vi "FP_Tracker_2.1.vi"(8 "error in (no error)":errorcluster, 11 "Settings file path":path=path "D:/Users/Dmitriy/CData/CloudStation/Tracker_repository/SubVi's/Tracker_settings.tcf") -> (0 "error out":errorcluster)   [LabVIEW 2018]
uses:
  <vilib>/Utility/config.llb/Config Data RefNum.ctl
  <vilib>/Utility/miscctls.llb/LVPoint32TypeDef.ctl
  SubVi's/Controls/CTL_Data_flow_control_cluster.ctl
  <vilib>/Instr/_visa.llb/VISA Flush IO Buffer Mask.ctl
  <vilib>/Utility/miscctls.llb/LVPointTypeDef.ctl
  <vilib>/Utility/miscctls.llb/LVOffsetAndMultiplierTypeDef.ctl
  <vilib>/Utility/miscctls.llb/LVRangeTypeDef.ctl
  <vilib>/Platform/TimedLoop/XDataNode/timing_clust.ctl
  <vilib>/Platform/TimedLoop/XDataNode/nitl_modes.ctl
  <vilib>/Platform/TimedLoop/XDataNode/wakeup.ctl
  <vilib>/Instr/_visa.llb/VISA Open Access Mode.ctl
  <vilib>/Utility/sysdir.llb/System Directory Type.ctl
  <vilib>/Utility/miscctls.llb/LVBoundsTypeDef.ctl
  <vilib>/ChannelSupport/Lossy Behavior.ctl
  <extravilib>/ChannelInstances/Lossy Stream-a[.](str)/Read With Abort.vi
  <extravilib>/ChannelInstances/Lossy Stream-a[.,.](str)/Read With Abort.vi
  <extravilib>/ChannelInstances/Lossy Stream-a[.](str)/Write With Abort.vi
  <extravilib>/ChannelInstances/Lossy Stream-a[.,.](str)/Write With Abort.vi
  <extravilib>/ChannelInstances/Lossy Stream-a[.](str)/EndpointRead.vi
  <extravilib>/ChannelInstances/Lossy Stream-a[.,.](str)/EndpointRead.vi
  <extravilib>/ChannelInstances/Lossy Stream-a[.](str)/Endpoint.vi
  <extravilib>/ChannelInstances/Lossy Stream-a[.,.](str)/Endpoint.vi
  SubVi's/SW_Globals.vi
  <vilib>/Platform/TimedLoop/scheduler/LVUserAPI/_suppVIs/Create_1kHz_TSource.vi
  <extravilib>/ChannelInstances/Lossy Stream-a[.](str)/Instantiate.vi
  <extravilib>/ChannelInstances/Lossy Stream-a[.,.](str)/Instantiate.vi
  <extravilib>/ChannelInstances/Lossy Stream-a[.](str)/)Channel.vi
  <resource>/ChannelSupport/_ChannelSupport/WaitIfNeeded.vi
  <extravilib>/ChannelInstances/Lossy Stream-a[.,.](str)/)Channel.vi
  <vilib>/Utility/file.llb/Write Delimited Spreadsheet (I64).vi
  <vilib>/Platform/TimedLoop/XDataNode/XDataNode.xnode
  <vilib>/Utility/config.llb/NI_LVConfig.lvlib
  Tracker.lvlib
  <vilib>/Utility/file.llb/Write Delimited Spreadsheet (string).vi
  <extravilib>/ChannelInstances/Lossy Stream-a[.,.](str).lvlib
  <vilib>/Platform/TimedLoop/XDataNode/XDNodeRunTimeDep.lvlib
  <vilib>/Analysis/NI_AALBase.lvlib
  <extravilib>/ChannelInstances/Lossy Stream-a[.](str).lvlib
  <vilib>/Utility/file.llb/Read Delimited Spreadsheet (string).vi
  Common_Resources.lvlib
panel:
  out "TTLs":u32[](array[numeric])
  in  "Zones preference empty initialized array":i32[](array[numeric])
  out "Timed structure (Streaming) and VISA error(s)":errorcluster
  out "VISA streaming error out":errorcluster
  out "Latest frame":string[](array[string])
  out "Serial port opened":bool
  in  "Open serial port":bool
  out "FP size change error":errorcluster
  out "FPS status":i32=80
  out "Data flow controls":T1
  in  "Streaming":bool
  out "write status":bool
  out "Last send packet size, bytes":u32
  out "PP status":string
  out "DAQ status":string
  out "Stop TTL is fired":bool
  out "Start TTL is fired":bool
  out "IO paramaters loaded from file":bool
  out "IO parameters loaded cluster":T2
  out "Settings load path":path caption="selected path"
  in  "\"Stop at\" enabled":bool
  in  "Serial OUT name":refnum<visa-resource-name>="Serial_Output"
  out "Output to the external terminal":string="00:00:00.000\t0.000000\t0.000000\t0.000000\t0.000000\t00.000000\t0.000000\t0\t0.000\r\n"
  in  "Twisted neck":bool
  in  "Bridge horizontal offset":sgl min=-70 max=70 step=0.1 format="%#.1g"
  in  "Name Prefix":string="SavedTrack"
  in  "Stop record at":dbl=600.0 caption="Stop at" min=0.0 max=43200.0 step=60.0 format="%<%H:%M:%S>t"
  out "Adv. Stim. set":bool
  in  "Save files First Call":bool=TRUE
  in  "Record start First Call":bool=TRUE
  out "Time per sample mean":dbl format="%0.2f"
  out "Time per sample SD":dbl format="%0.2f"
  out "Save iteration duration":i64
  out "standard deviation":dbl format="%0.2f"
  out "mean":dbl format="%0.2f"
  in  "Type of histogram":u8
  out "TTL 4 counter":u32
  out "TTL 3 counter":u32
  out "TTL 2 counter":u32
  out "TTL 1 counter":u32
  out "Full track plotting":u32
  out "Full track preparation":u32
  out "Main queue":refnum<queue>
  in  "Map index (analysis)":i32
  in  "Full trace color":u32(colorbox)=16711680
  out "Current TTL status":u8
  out "TTL inputs":u8[](array[numeric])
  out "TTL outputs":u8[](array[numeric])
  out "Start/Stop in config":u32
  out "Start/Stop out pulses config":u32
  out "Changed IO":bool
  out "Sync capability":u8
  in  "IO parameters string":string
  out "Reset STIM":bool
  out "Reset REG":bool
  out "Init plot":bool=TRUE
  out "Zones preference array (loaded)":dbl[][](array[numeric])
  out "Current zone":dbl[](array[numeric])
  out "Absolute timestamp (rec)":dbl[](array[numeric])
  in  "Colors for Stim. setup":T3(array[cluster])=[{"Not Selected"=1143775, "Not Selected"=1143775}, {"Not Selected"=14517504, "Not Selected"=14517504}, {"Not Selected"=1976113, "Not Selected"=1976113}, {"Not Selected"=2575993, "Not Selected"=2575993}]
  out "Record":bool
  out "Stopped":bool
  out "Reset starting pulse":bool
  out "TTL is long enough":bool
  out "Started":bool
  out "Coords":T4={"Horizontal"=316, "Vertical"=127}
  out "Button":u16=1
  out "Settings file path":path
  out "Track path":path
  out "Index of the last recorded timepoint":i32
  out "ceil(x): smallest int >= x":dbl
  out "Application Directory":path
  out "Path to the settings file":path=path "D:/Users/Dmitriy/CData/CloudStation/Tracker_repository/Tracker_settings.tcf"
  out "Eff. save interval":sgl=7.981
  out "Relative timestamp (rec)":dbl[](array[numeric])
  out "alpha rot. angle":dbl[](array[numeric])
  out "Y coord":dbl[](array[numeric])
  out "X coord":dbl[](array[numeric])
  out "Zones allocation array":i32[](array[numeric])
  out "Zones presence array":bool[](array[boolean])
  in  "Stop Button":bool
  out "Path to the latest saved temp file":path
  out "Temp file ready":bool
  out "Pixels per mm":dbl=1.1663076923076923
  out "Settings file refnum out":T5
  out "Current User":string="Researcher"
  in  "Main tab control":enum32{"Settings", "Recording", "Analysis"}(tab)
  in  "Set advanced stimulus":bool
  in  "Load settings":bool
  out "IO status indicator":T6
  in  "Set IO config":bool
  in  "Jump to Analysis":bool
  in  "Reset stimuli":bool
  in  "Stimulus presets":T7(array[cluster]) {"TTL out" items=["1"=1, "2"=2, "1 + 2"=3]; "Stimulus, s" min=0 max=10000 step=0.1; "Time, s" min=0 max=10000 step=0.1; "Event type" items=["Time spent in zone", "Future options"]}
  in  "Zone-based stimulus setup":T8(radio)=enum."Zone 13"
  out "Ready":bool=TRUE
  in  "Re-check HW connection":bool
  in  "Reset regions":bool
  in  "Start Tracking button":bool
  in  "Starting angle BORDER":i16
  in  "N segments BORDER":u8=5 min=1 max=12
  in  "N segments MIDFIELD":u8=3 max=8
  in  "Starting angle MIDFIELD":i16=30
  in  "Radius, mm MIDFIELD":u16=110
  in  "Radius, mm CENTER":u16=50 min=5 step=1
  out "Board size":string="Large"
  in  "Cage diameter, mm":u16(ring)=333 items=["180 mm"=180, "240 mm"=240, "290 mm"=290, "325 mm"=325, "327 mm"=327, "333 mm"=333]
  out "Segments diagram":picture
  out "HW info":string
  out "Port":string="Large"
  in  "Expand/hide stream panel (Set)":bool
  out "Run times distrib. indicator":bool
  out "IO pulses count":string
  in  "Bridge swap":bool
  in  "Reset barplot":bool
  out "Mouse speed digi":dbl=0.28949046360238656 caption="Mouse speed" format="%05.1f"
  out "Histograms (normalized)":dbl[](graph)=[0.0, 0.0, 0.0, 0.0, 0.0, 0.0, 0.0, 1.0, 0.0, 0.0, 0.0, 0.0, 0.0, 0.0] caption="Zone preference (normalized)"
  in  "Multiplyer of chart RX":u8(slide)=1 min=1 max=10 step=1 scale=1.0..6.0
  in  "Zones presence indicator":T9={"01"=TRUE, "02"=TRUE, "03"=TRUE, "04"=TRUE, "05"=TRUE, "06"=TRUE, "07"=TRUE, "08"=TRUE, "09"=TRUE, "10"=TRUE, "11"=TRUE, "12"=TRUE, "13"=TRUE}
  in  "Zones":bool=TRUE
  in  "Record/Stop":bool
  out "Diagram at recording":picture caption="Mouse track"
  in  "Trace, s":u16(slide)=5 max=30 step=1 scale=0.0..30.0
  in  "Data filtering":u16(ring)=5 items=["None"=0, "Kalman 1/3"=2, "Kalman 1/8"=3, "SG 3/5"=4, "SG 3/11"=5, "SG 3/31"=6]
  out "Record timestamp":dbl format="%<%H:%M:%S%3u>t"
  out "Current Time":timestamp=timestamp(3610093053.229 s since 1904-01-01) format="%<%H:%M:%S %d.%m.%Y>T"
  in  "Exit (recording)":bool
  out "Mouse speed":waveform(dbl)(graph)={"t0"=timestamp(3610093053.229 s since 1904-01-01), "dt"=1.0, "Y"=[0.28949046360238656]}
  in  "Bridge offset":sgl min=-150 max=150 step=0.1 format="%#.1g"
  out "TTL IO 1 (recording)":bool caption="IO 1"
  out "TTL IO 2 (recording)":bool caption="IO 2"
  out "TTL IO 3 (recording)":bool caption="IO 3"
  out "TTL IO 4 (recording)":bool caption="IO 4"
  out "TTL REC":bool
  out "Mouse running, perc. of time":dbl=0.28949046360238656 caption="Run, %" format="%05.2f"
  out "Zones presense indicator":bool=TRUE
  out "Speed distrib. indicator":bool
  out "Run lengts distrib. indicator":bool
  in  "Additional record settings":bool caption="Add. recording settings"
  in  "Expand/hide stream panel (Rec)":bool
  out "Key_pressed":string
  in  "Back to Settings":bool
  out "Data loading progress":dbl(slide) scale=0.0..100.0
  in  "Speed":u16(ring)=3 items=["25"=75, "10"=30, "6"=18, "4"=12, "2"=6, "1"=3, "2/3"=2, "1/3"=1]
  in  "Timeline":dbl(slide) min=0.0 step=1.0 scale=0.0..656.633 scale format="%<%H:%M:%S>t"
  in  "Multiplyer of chart RX 2":u8(slide)=1 min=1 max=10 step=1 scale=1.0..6.0
  out "Diagram at analysis":picture caption="Mouse track"
  in  "Play/Pause":bool
  out "Recorded at time":timestamp format="%<%H:%M:%S %d.%m.%Y>T"
  out "Recorded timestamp":dbl format="%<%H:%M:%S%3u>t"
  in  "Zones (analysis)":bool=TRUE caption="Zones"
  out "Mouse speed 2":waveform(dbl)(graph) caption="Mouse speed"
  out "Mouse speed digi 2":dbl format="%05.1f"
  out "Zones allocation (normalized) in analysis":dbl[](graph) caption="Zone preference (normalized)"
  out "Recorded by":string
  in  "Trace in analysis, s":u16(slide)=2 caption="Trace, s" max=30 step=1 scale=0.0..30.0
  in  "Open File":bool
  out "Bridge swap (analysis)":bool caption="Swapped"
  in  "Show heatmap (analysis)":bool caption="Heat map"
  in  "Show full track (analysis)":bool caption="Full track"
  out "Bridge Vertical offset (analysis)":sgl caption="Br. offset" min=-60 max=60 step=0.1 format="%#.1g"
  out "TTL IO 2 (analysis)":bool
  out "TTL IO 1 (analysis)":bool
  out "TTL IO 3 (analysis)":bool
  out "TTL IO 4 (analysis)":bool
  in  "Expand/hide stream panel (An)":bool
  out "Click coords, mm":cluster{"X":dbl, "Y":dbl} {"Y" format="%.1f"; "X" format="%.1f"}
  # "v.2.1.10.6"
  # "Cage segmentation"
  # "BORDER"
  # "CENTER"
  # "MIDFIELD"
  # "v.2.1.10.6"
  # "v.2.1.10.6"
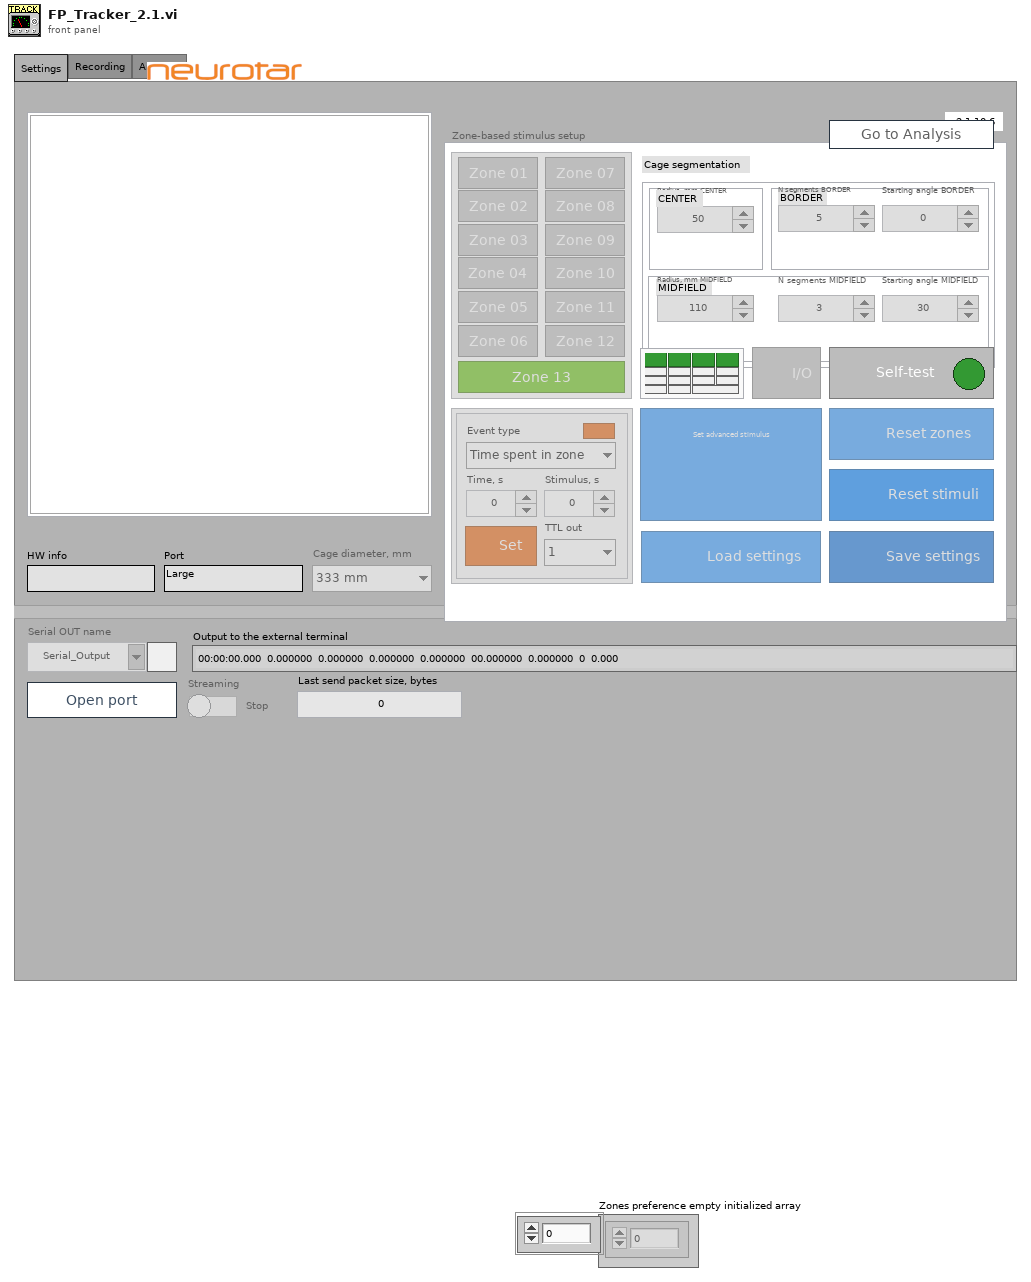
[diagram p1: front panel]
types:
  T1 = typedef "Common_Resources.lvlib/CTL_Data_flow_control_cluster.ctl" = cluster{"Data acquisition status":refnum<notifier>, "Play/Pause status":refnum<notifier>, "Complete stop":refnum<notifier>, "Temp file ready for processing":refnum<notifier>, "Has been recorded":refnum<notifier>, "Recording now":refnum<notifier>, "Path to the latest complete temp file":refnum<notifier>, "(Final) Data file is saved":refnum<notifier>, "Data loaded":refnum<notifier>}
  T2 = cluster{"SYNC configuration":u16, "IO 1 configuration":u16, "IO 2 configuration":u16, "IO 3 configuration":u16, "IO 4 configuration":u16, "Activate ext. RS-232":u16, "IO inversion config.":u16}
  T3 = cluster{"Not Selected":u32, "Not Selected":u32}[]
  T4 = typedef "LVPoint32TypeDef.ctl" = cluster{"Horizontal":i32, "Vertical":i32}
  T5 = typedef "NI_LVConfig.lvlib/Config Data RefNum.ctl" = refnum<k1>
  T6 = cluster{"IO1":bool, "IO2":bool, "IO3":bool, "IO4":bool, "Z1":bool, "Z2":bool, "Z3":bool, "Z4":bool, "St1":bool, "St2":bool, "St3":bool, "St4":bool, "Syn1":bool, "Syn2":bool, "RS-232 ext. activated":bool}
  T7 = cluster{"Event type":u16, "Time, s":sgl, "Stimulus, s":sgl, "Set/Clear":bool, "TTL out":u16, "Stim. has been set":bool}[]
  T8 = enum32{"No Selection", "Zone 01", "Zone 02", "Zone 03", "Zone 04", "Zone 05", "Zone 06", "Zone 07", "Zone 08", "Zone 09", "Zone 10", "Zone 11", "Zone 12", "Zone 13"}
  T9 = cluster{"01":bool, "02":bool, "03":bool, "04":bool, "05":bool, "06":bool, "07":bool, "08":bool, "09":bool, "10":bool, "11":bool, "12":bool, "13":bool}
  T10 = cluster{"SG coefficients 3/5":cluster{"0th order SG coefficients":dbl[], "1st order SG coefficients":dbl[]}, "SG coefficients 3/11":cluster{"0th order SG coefficients":dbl[], "1st order SG coefficients":dbl[]}, "SG coefficients 3/31":cluster{"0th order SG coefficients":dbl[], "1st order SG coefficients":dbl[]}, "SG coefficients 3/51":cluster{"0th order SG coefficients":dbl[], "1st order SG coefficients":dbl[]}}
  T11 = cluster{"Numeric Control":u32, "Numeric Control":u32}[]
  T12 = enum8{"Enabled", "Disabled", "Disabled and Grayed Out"}
  T13 = typedef "XDNodeRunTimeDep.lvlib/timing_clust.ctl" = cluster{"Expected End [f-1]":u64, "Actual End [f-1]":u64, "Finished Late? [f-1]":bool, "Expected End [i-1]":u64, "Actual End [i-1]":u64, "Finished Late? [i-1]":bool, "Expected Start [i]":u64, "Actual Start [i]":u64, "Expected Start [f]":u64, "Actual Start [f]":u64, "Source Name":string, "Structure Name":string, "Period":i64, "Deadline":i64, "Offset":i64, "Start":i64, "Priority":i32, "Timeout":i32, "Mode":T14, "Wakeup Reason":T15, "Error":errorcluster, "Source Type":string, "Secondary Source Type":string, "Global End Time":u64, "Global Start Time":u64, "Frame Duration":u64, "Iteration Duration":u64, "Assigned CPU":i32, "I/O Scan Engine Mode":u32}
  T14 = typedef "XDNodeRunTimeDep.lvlib/nitl_modes.ctl" = enum32{"No Change", "Process missed periods, maintain original phase", "Discard missed periods, maintain original phase", "Process missed periods, ignore original phase", "Discard missed periods, ignore original phase"}
  T15 = typedef "XDNodeRunTimeDep.lvlib/wakeup.ctl" = enum32{"Normal", "Aborted", "Asynchronous wakeup", "Timing source error", "Timed loop error", "Timeout"}
  T16 = cluster{"Read buffer":string, "Timestamp":timestamp}
  T17 = cluster{"Data acquisition status":refnum<notifier>, "Play/Pause status":refnum<notifier>, "Complete stop":refnum<notifier>, "Temp file ready for processing":refnum<notifier>, "Has been recorded":refnum<notifier>, "Recording now":refnum<notifier>, "Path to the latest complete temp file":refnum<notifier>, "Final CSV saved":refnum<notifier>, "Data loaded":refnum<notifier>}
  T18 = typedef "VISA Flush IO Buffer Mask.ctl" = u16
  T19 = typedef "LVBoundsTypeDef.ctl" = cluster{"Width":u32, "Height":u32}
  T20 = cluster{"Amount of border segments":u8, "Border segments starting angle":i16, "Amount of midfield segments":u8, "Midfield segments starting angle":i16, "Midfield segments outer radius, mm":u16, "Amount of central segments":u8, "Center segment outer radius, mm":u16, "Diameter of the cage, mm":u16, "R-gap between segments, mm":u8}
  T21 = typedef "LVRangeTypeDef.ctl" = cluster{"Minimum":dbl, "Maximum":dbl, "Increment":dbl, "Minor Increment":dbl, "Start":dbl}
  T22 = cluster{"Temporary file output path":path, "Density map array output path":path, "Recording settings output path":path, "Density map picture output path":path, "Layout picture output path":path, "Path to the settings file":path, "Path to TDMS file":path, "TDMS file reference":refnum<k34>}
  T23 = cluster{"Zones preference array (loaded)":dbl[][], "TTL inputs":u8[], "TTL outputs":u8[], "Stimulus presets array (loaded)":cluster{"Event type":u16, "Time, s":sgl, "Stimulus, s":sgl, "Set/Clear":bool, "TTL out":u16, "Stim. has been set":bool}[], "Absolute timestamp":dbl[], "Relative timestamp":dbl[], "X coord":dbl[], "Y coord":dbl[], "alpha rot. angle":dbl[], "Current zone":dbl[], "Acquisition settings cluster out":cluster{"Researcher name":string, "N segments MIDFIELD":u8, "N segments BORDER":u8, "Radius, mm CENTER":u16, "Radius, mm MIDFIELD":u16, "Starting angle MIDFIELD":i16, "Starting angle BORDER":i16, "Cage diameter, mm":u16, "Bridge swap":bool, "Bridge V. offset":sgl, "Twisted neck":bool, "Offset H.":sgl, "Name prefix":string, "Stop at":dbl, "\"Stop at\" enabled":bool, "Settings loaded OK":bool}, "Data column names":string[]}
  T24 = cluster{"Absolute timestamp (DBL)":dbl[], "Relative timestamp (DBL)":dbl[], "Zones normalized allocation array":dbl[][], "Coordinates and speed":dbl[][], "Current zone and TTLs":u8[][], "Acquisition settings cluster out":cluster{"Researcher name":string, "N segments MIDFIELD":u8, "N segments BORDER":u8, "Radius, mm CENTER":u16, "Radius, mm MIDFIELD":u16, "Starting angle MIDFIELD":i16, "Starting angle BORDER":i16, "Cage diameter, mm":u16, "Bridge swap":bool, "Bridge V. offset":sgl, "Twisted neck":bool, "Offset H.":sgl, "Name prefix":string, "Stop at":dbl, "\"Stop at\" enabled":bool, "Settings loaded OK":bool}, "Stimulus presets array":cluster{"Event type":u16, "Time, s":sgl, "Stimulus, s":sgl, "Set/Clear":bool, "TTL out":u16, "Stim. has been set":bool}[]}
  T25 = cluster{"Researcher name":string, "N segments MIDFIELD":u8, "N segments BORDER":u8, "Radius, mm CENTER":u16, "Radius, mm MIDFIELD":u16, "Starting angle MIDFIELD":i16, "Starting angle BORDER":i16, "Cage diameter, mm":u16, "Bridge swap":bool, "Bridge V. offset":sgl, "Twisted neck":bool, "Offset H.":sgl, "Name prefix":string, "Stop at":dbl, "\"Stop at\" enabled":bool, "Settings loaded OK":bool}
  T26 = typedef "imagedata.ctl" = cluster{"image type":i32, "image depth":i32, "image":u8[], "mask":u8[], "colors":u32[], "Rectangle":cluster{"left":i16, "top":i16, "right":i16, "bottom":i16}}
  T27 = cluster{"Fonts scale factor":dbl, "Pixels per mm":dbl, "Radius of displayed outer segments, pix":dbl, "Radius of displayed midfield segments, pix":dbl, "Radius of displayed central segment, pix":dbl}
  T28 = cluster{"Width":u16, "Style":enum32{"Solid", "Dash", "Dot", "DashDot", "DashDotDot"}}
  T29 = cluster{"N segments BORDER":u8, "Starting angle BORDER":i16, "N segments MIDFIELD":u8, "Starting angle MIDFIELD":i16, "Radius, mm MIDFIELD":u16, "Amount of central segments":u8, "Radius, mm CENTER":u16}
  T30 = typedef "LVOffsetAndMultiplierTypeDef.ctl" = cluster{"Offset":dbl, "Multiplier":dbl}
  T31 = enum32{"No Selection", "Zone 01", "Zone 02", "Zone 03", "Zone 04", "Zone 05", "Zone 06", "Zone 07", "Zone 08", "Zone 09", "Zone 10", "Zone 11", "Zone 12", "Zone 13", "Zone 14"}
  T32 = enum32{"Page Enabled", "Page Disabled", "Page Disabled & Grayed"}
  T33 = typedef "LVPointTypeDef.ctl" = cluster{"Horizontal":i16, "Vertical":i16}
  T34 = enum32{"invalid app kind", "Development System", "Run Time System", "Student Edition", "Embedded LabVIEW", "Evaluation", "Custom"}
  T35 = cluster{"Researcher name":string, "N segments MIDFIELD":u8, "N segments BORDER":u8, "Radius, mm CENTER":u16, "Radius, mm MIDFIELD":u16, "Starting angle MIDFIELD":i16, "Starting angle BORDER":i16, "Cage diameter, mm":u16, "Bridge swap":bool, "Bridge V. offset":sgl, "Twisted neck":bool, "Offset H.":sgl, "Name prefix":string, "Stop at":dbl, "\"Stop at\" enabled":bool, "Data filtering":u16, "Settings loaded OK":bool}
  T36 = cluster{"Event type":u16, "Dur., s":sgl, "Stim., s":sgl, "Set/Clear":bool, "TTL out N":u16, "Stim. has been set":bool}[]
  T37 = typedef "Common_Resources.lvlib/CTL_IO_status_indicator.ctl" = cluster{"IO1":bool, "IO2":bool, "IO3":bool, "IO4":bool, "St1":bool, "St2":bool, "St3":bool, "St4":bool, "Z1":bool, "Z2":bool, "Z3":bool, "Z4":bool, "Syn1":bool, "Syn2":bool, "RS-232 ext. activated":bool}
  T38 = cluster{"0th order SG coefficients":dbl[], "1st order SG coefficients":dbl[]}
  T39 = typedef "Lossy Behavior.ctl" = enum16{"drop oldest element", "skip this write"}
  T40 = cluster{"Offset V.":sgl, "Offset H.":sgl, "Bridge swap":bool, "Turn magnets 90 deg.":bool, "Twisted neck":bool}
  T41 = typedef "Lossy Stream-a[.](str).lvlib/)Channel.ctl" = refnum<queue>
  T42 = typedef "Lossy Stream-a[.,.](str).lvlib/)Channel.ctl" = refnum<queue>
  T43 = cluster{"Read buffer":string, "Timestamp":timestamp}[]
  T44 = typedef "LVRectTypeDef.ctl" = cluster{"Left":i16, "Top":i16, "Right":i16, "Bottom":i16}
  T45 = typedef "eventvkey.ctl" = enum16{"ASCII", "Enter", "Return", "Shift", "Ctrl", "Alt", "Cmd", "Opt", "Caps", "NumLock", "Clear", "Break", "Up", "Down", "Left", "Right", "Insert", "Delete", "Home", "End", "PageUp", "PageDown", "Escape", "Help", "Pause", "ScrollLock", "F1", "F2", "F3", "F4", "F5", "F6", "F7", "F8", "F9", "F10", "F11", "F12", "F13", "F14", "F15", "F16", "F17", "F18", "F19", "F20", "F21", "F22", "F23", "F24", "Play", "VolumeUp", "VolumeDown", "Mute", "Two Byte Char"}
  T46 = typedef "VISA Open Access Mode.ctl" = u32
  T47 = cluster{"Event type":u16, "Cond., s":sgl, "Stim., s":sgl, "Set/Clear":bool, "TTL out N":u16, "Stim. has been set":bool}
  T48 = cluster{"Offset V.":sgl, "Offset H.":sgl, "Bridge swap":bool, "Twisted neck":bool, "Name prefix":string, "Stop at":dbl, "\"Stop at\" enabled":bool}
  T49 = cluster{"N segments BORDER":u8, "Starting angle BORDER":i16, "N segments MIDFIELD":u8, "Starting angle MIDFIELD":i16, "Radius, mm MIDFIELD":u16, "Amount of central segments":u8, "Radius, mm CENTER":u16, "Bridge swap":bool, "Bridge V. offset":sgl, "Twisted neck":bool, "Offset H.":sgl, "Zones configuration":string[], "IO parameters string":string, "Cage diameter, mm":u16, "Name prefix":string, "Stop at":dbl, "\"Stop at\" enabled":bool, "Data filtering":u16}
  T50 = cluster{"SYNC configuration":bool, "IO 1 configuration":bool, "IO 2 configuration":bool, "IO 3 configuration":bool, "IO 4 configuration":bool, "Activate ext. RS-232":bool, "IO inversion config.":bool}
  T51 = cluster{"Event type":u16, "Cond., s":sgl, "Stim., s":sgl, "Set/Clear":bool, "TTL out N":u16, "Stim. has been set":bool}[]
  T52 = cluster{"Event type":u16, "Time, s":sgl, "Stimulus, s":sgl, "Set/Clear":bool, "TTL out":u16, "Stim. has been set":bool}
  T53 = typedef "System Directory Type.ctl" = i32
  T54 = cluster{"N segments BORDER":u8, "Starting angle BORDER":i16, "N segments MIDFIELD":u8, "Starting angle MIDFIELD":i16, "Radius, mm MIDFIELD":u16, u8, "Radius, mm CENTER":u16, "Cage diameter, mm":u16, i32}
  T55 = cluster{"N segments BORDER":u8, "Starting angle BORDER":i16, "N segments MIDFIELD":u8, "Starting angle MIDFIELD":i16, "Radius, mm MIDFIELD":u16, "N segments CENTER":u8, "Radius, mm CENTER":u16, "Cage diameter, mm":u16, "R-gap":i32}
  T56 = cluster{"Zone[1]":bool, "Zone[2]":bool, "Zone[3]":bool, "Zone[4]":bool, "Zone[5]":bool, "Zone[6]":bool, "Zone[7]":bool, "Zone[8]":bool, "Zone[9]":bool, "Zone[10]":bool, "Zone[11]":bool, "Zone[12]":bool, "Zone[13]":bool}
  T57 = typedef "LVStringsAndValuesArrayTypeDef_U16.ctl" = cluster{"String":string, "Value":u16}[]
  T58 = typedef "LVPositionTypeDef.ctl" = cluster{"Left":i32, "Top":i32}
  T59 = cluster{"Numeric Control":dbl, "Numeric Control":dbl}
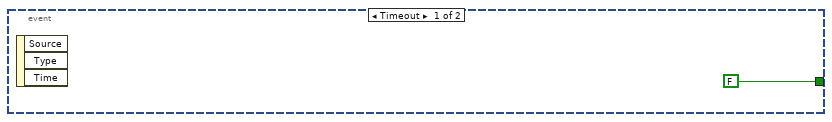
[diagram p4: hidden frame]
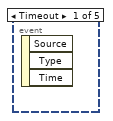
[diagram p7: hidden frame]
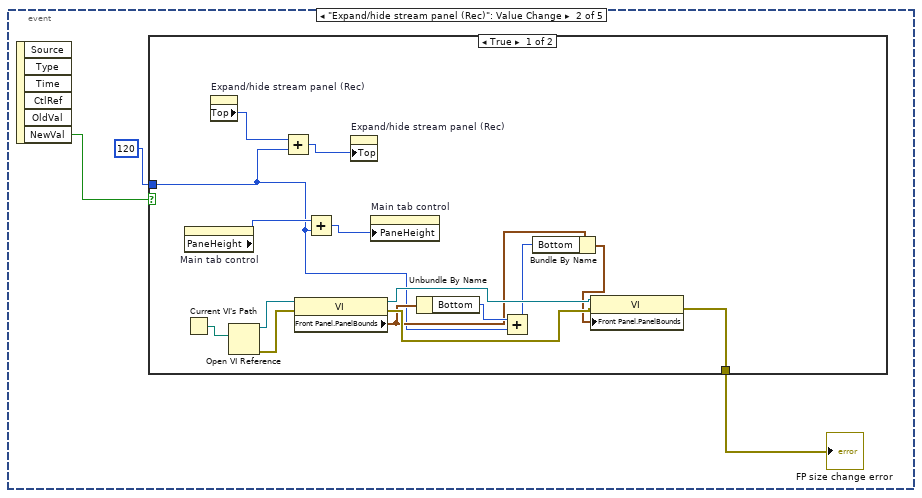
[diagram p8: hidden frame]
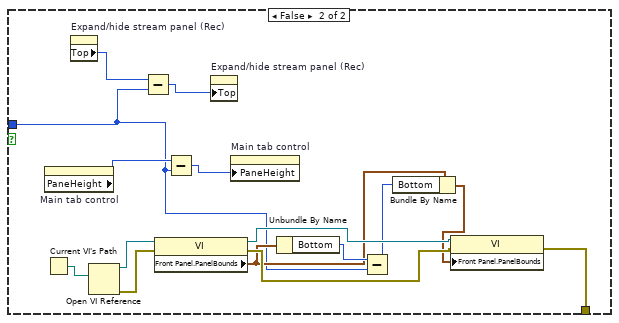
[diagram p9: hidden frame]
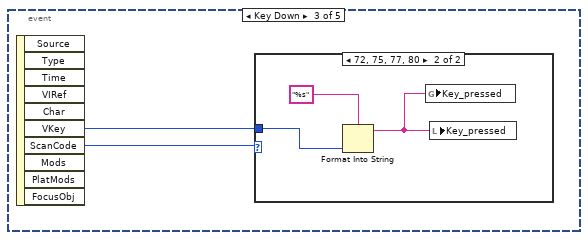
[diagram p10: hidden frame]
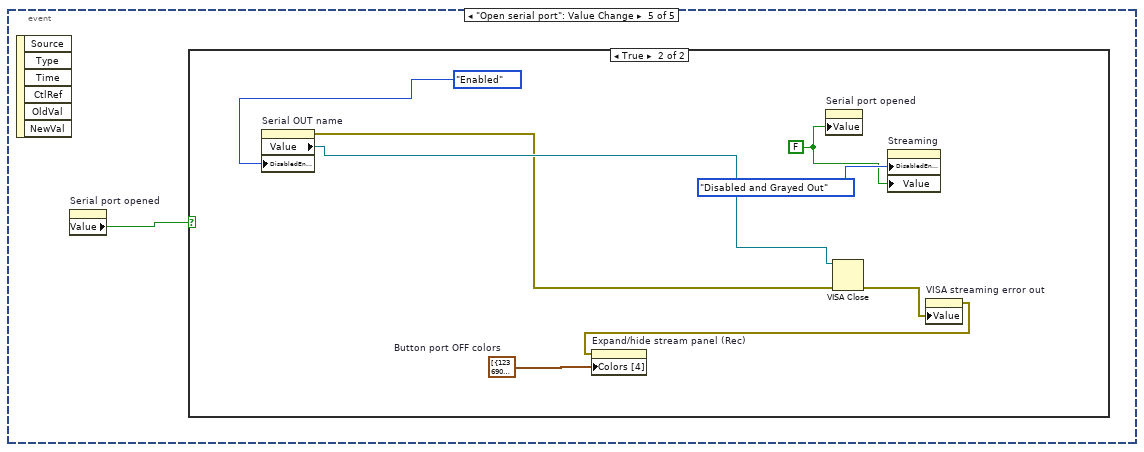
[diagram p13: hidden frame]
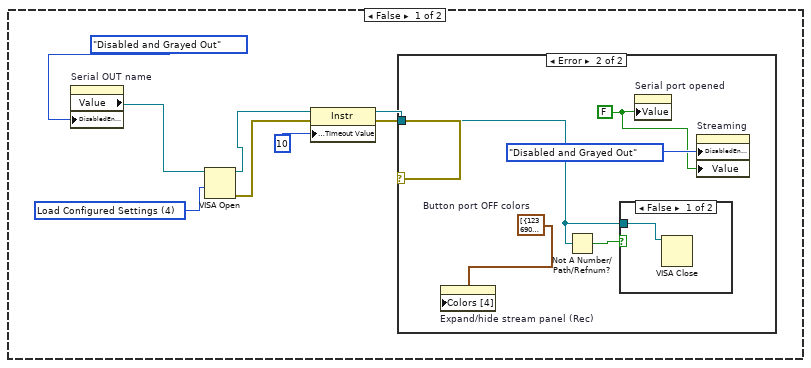
[diagram p14: hidden frame]
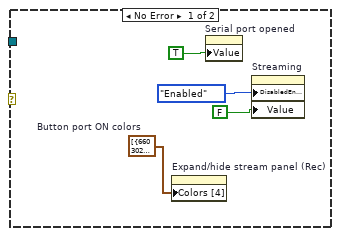
[diagram p15: hidden frame]
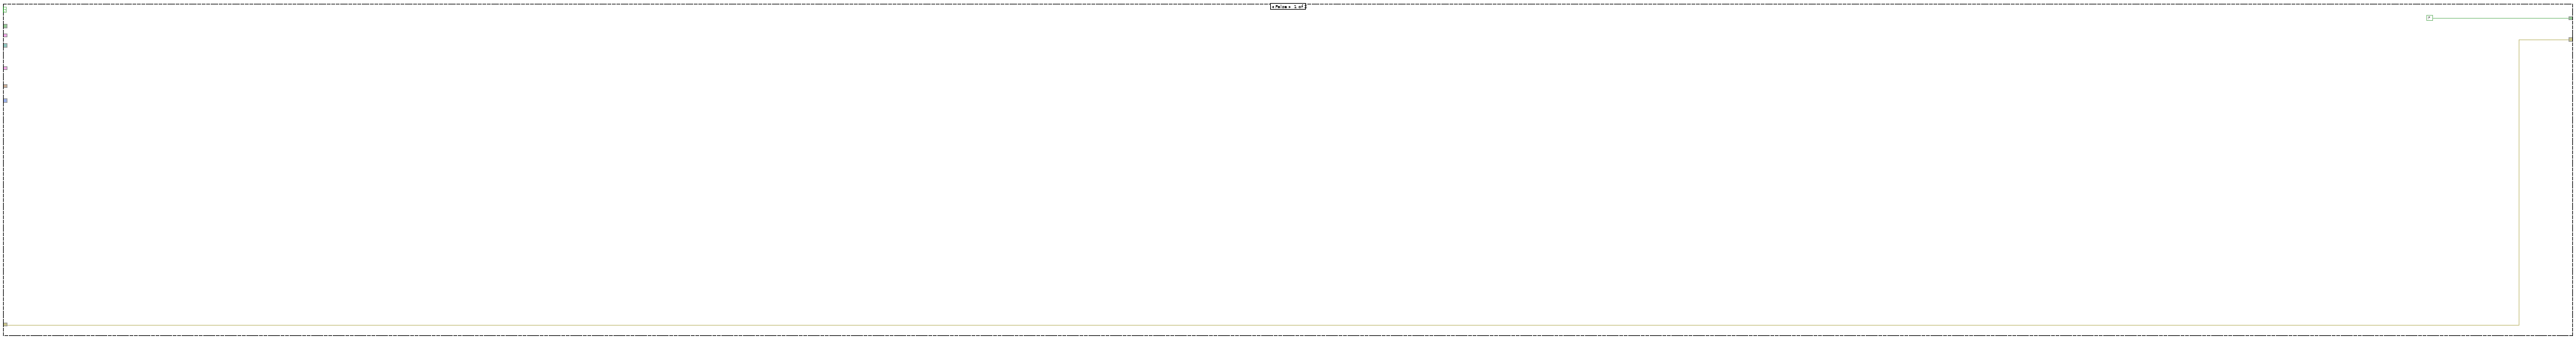
[diagram p17: hidden frame]
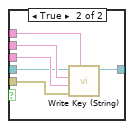
[diagram p20: hidden frame]
diagram:
  w21 = u16 3 items=["3/5", "3/11", "3/31", "3/51"] ("Select filter length")
  w23 = u16 2 items=["3/5", "3/11", "3/31", "3/51"] ("Select filter length")
  w27 = u16 1 items=["3/5", "3/11", "3/31", "3/51"] ("Select filter length")
  w31 = u16 0 items=["3/5", "3/11", "3/31", "3/51"] ("Select filter length")
  w40 = i64 37 ("Period")
  w48 = i64 23 ("Period")
  n1 = node-c288(w18, i64 1 ("Period"), 65000 ("Priority")) -> (w57:T13)
  n2 = disable-structure shown="Default" {
    disable-tunnel: [w69] -> w37
    frame Enabled {
      w68 = T12."Disabled and Grayed Out" ("Disabled")
      n3 = property on="Cage diameter, mm" class="Ring (strict)"("DisabledEnum"=w68) -> ()  [unwired: 2 in, 2 out]
      n4 = property on="Load settings" class="Bool (strict)"("DisabledEnum"=w68) -> ()  [unwired: 2 in, 2 out]
      n5 = property on="Set IO config" class="Bool"("DisabledEnum"=w68) -> ()  [unwired: 2 in, 2 out]
      n6 = property on="Starting angle MIDFIELD" class="DigNum (strict)"("DisabledEnum"=w68) -> ()  [unwired: 2 in, 2 out]
      n7 = property on="N segments MIDFIELD" class="DigNum (strict)"("DisabledEnum"=w68) -> ()  [unwired: 2 in, 2 out]
      n8 = property on="Radius, mm MIDFIELD" class="DigNum (strict)"("DisabledEnum"=w68) -> ()  [unwired: 2 in, 2 out]
      n9 = property on="Starting angle BORDER" class="DigNum (strict)"("DisabledEnum"=w68) -> ()  [unwired: 2 in, 2 out]
      n10 = property on="N segments BORDER" class="DigNum (strict)"("DisabledEnum"=w68) -> ()  [unwired: 2 in, 2 out]
      n11 = property on="Radius, mm CENTER" class="DigNum (strict)"("DisabledEnum"=w68) -> ()  [unwired: 2 in, 2 out]
      n12 = property on="Start Tracking button" class="Bool"("DisabledEnum"=w68) -> ()  [unwired: 2 in, 2 out]
      n13 = property on="Reset stimuli" class="Bool (strict)"("DisabledEnum"=w68) -> ()  [unwired: 2 in, 2 out]
      n14 = property on="Reset regions" class="Bool (strict)"("DisabledEnum"=w68) -> (error out=w69:errorcluster)  [unwired: 2 in, 1 out]
      n15 = property on="Zone-based stimulus setup" class="RadioBtnsControl (strict)"("DisabledEnum"=w68) -> ()  [unwired: 2 in, 2 out]
      n16 = property on="Set advanced stimulus" class="Bool (strict)"("DisabledEnum"=w68) -> ()  [unwired: 2 in, 2 out]
    }
  }
  n17 = property on="Re-check HW connection" class="Bool"(error in=w37, "DisabledEnum"=T12."Disabled and Grayed Out" ("Disabled")) -> (error out=w62:errorcluster)  [unwired: 1 in, 1 out]
  n18 = property on="Ready" class="Bool (strict)"(error in=w62, "Value"=FALSE ("Ready"), "Colors [4]"=T11 [{"Numeric Control"=16749459, "Numeric Control"=16749459}, {"Numeric Control"=1988894, "Numeric Control"=3381555}, {"Numeric Control"=4934475, "Numeric Control"=7895160}, {"Numeric Control"=994319, "Numeric Control"=1657881}]) -> (error out=w33:errorcluster)  [unwired: 1 in, 1 out]
  n19 = node-c288(w18, i64 1201 ("Period"), 50 ("Priority")) -> (w46:T13)
  n20 = timed-loop {
    tunnel: w67 -> [w70]
    tunnel: [w73] -> w38
    tunnel: [w89] -> w1
    tunnel: [w74] -> w64
    tunnel: [w88] -> w17
    tunnel: w33 -> [w84]
    tunnel: [w77] -> w58
    timing: w46 -> [_]
    timing-out: [_] -> w45
    stop <- w72 stop-if-true
    n21 = node-c288() -> ()  [unwired: 1 in, 1 out]
    n22 = property on="Re-check HW connection" class="Bool"(error in=w84, "DisabledEnum"=T12."Enabled" ("Disabled")) -> (error out=w83:errorcluster)  [unwired: 1 in, 1 out]
    n23 = First Call?() -> (First Call?: T/F=w75:bool)
    n24 = property on="Ready" class="Bool (strict)"(error in=w83) -> (error out=w87:errorcluster, "Value"=w86:bool)  [unwired: 1 in, 1 out]
    n25 = Or(x=w75, y="Re-check HW connection") -> (x .or. y?=w76:bool)
    n26 = Not(x=w86) -> (.not. x?=w82:bool)
    n27 = And(x=w82, y=w76) -> (x .and. y?=w81:bool)
    n28 = case shown="True" w81 {
      tunnel: w70 -> [w95 w125]
      tunnel: [w93 w124] -> w89
      tunnel: [w95 w123] -> w74
      tunnel: [w92 w122] -> w88
      tunnel: [w96 w97] -> w78
      tunnel: [FALSE ("Instrument OK?") w112] -> w73
      tunnel: w87 -> [w96 w100]
      frame False {
        n29 = local read "Data flow controls"() -> (w92:T1)
        n30 = local read "Main queue"() -> (w93:refnum<queue>)
      }
      frame True {
        w121 = T16 {"Read buffer"="", "Timestamp"=timestamp(3605695211.9516535 s since 1904-01-01)}  # Data frame example
        n31 = call <vilib>:"Set Busy.vi"("error in (no error)"=w100) -> ("error out"=w99:errorcluster)  [unwired: 9 in, 1 out]
        n32 = property on="Ready" class="Bool (strict)"(error in=w99, "Colors [4]"=T11 [{"Numeric Control"=16749459, "Numeric Control"=16176658}, {"Numeric Control"=1988894, "Numeric Control"=3381555}, {"Numeric Control"=4934475, "Numeric Control"=7895160}, {"Numeric Control"=994319, "Numeric Control"=1657881}]) -> (error out=w110:errorcluster)  [unwired: 1 in, 1 out]
        n33 = Obtain Queue(name (unnamed)="Data flow", element data type=w121, error in (no error)=w110) -> (queue out=w124:refnum<queue>, error out=w119:errorcluster)  [unwired: 2 in, 1 out]
        "Main queue" <- w124
        n34 = call "HW_Setup.vi"("error in"=w119, "Traget FPS"=80, "VISA resource name in"=w125) -> ("FPS status"=→"FPS status":i32, "Instrument OK?"=w112:bool, "Data flow controls"=w122:T1, "VISA resource name out"=w123:refnum<visa-resource-name>, "Version information"=w109:string, "Sensor board size"=w102:string, "error out"=w98:errorcluster)  [unwired: 1 in, 1 out]
        "Ready" <- w112
        "Board size" <- w102
        "Data flow controls" <- w122
        n35 = String Length(string=w109) -> (length=w116:i32)
        n36 = Equal?(x=w109, y="1.1.4") -> (x = y?=w106:bool)
        n37 = Greater Than 0?(x=w116) -> (x > 0?=w115:bool)
        n38 = Concatenate Strings(w102, ", FW: " ("string"), w109) -> (w114:string)
        n39 = Select(t=u8 0, s=w106, f=u8 1) -> (s? t:f=→"Sync capability":u8)
        n40 = Select(t=w114, s=w115, f="Not connected") -> (s? t:f=→"HW info":string)
        n41 = call <vilib>:"Unset Busy.vi"("error in (no error)"=w98) -> ("error out"=w97:errorcluster)  [unwired: 10 in]
      }
    }
    n42 = property on="Jump to Analysis" class="Bool (strict)"() -> ("Value"=w71:bool)  [unwired: 2 in, 2 out]
    n43 = Or(x=w73, y=w71) -> (x .or. y?=w72:bool)
    n44 = global write "SW_Globals.vi" "VISA resource name"(w74) -> ()
    n45 = property on="Ready" class="Bool (strict)"(error in=w78, "Colors [4]"=T11 [{"Numeric Control"=16749459, "Numeric Control"=16749459}, {"Numeric Control"=1988894, "Numeric Control"=3381555}, {"Numeric Control"=4934475, "Numeric Control"=7895160}, {"Numeric Control"=994319, "Numeric Control"=1657881}]) -> (error out=w77:errorcluster)  [unwired: 1 in, 1 out]
    n46 = node-c288() -> ()  [unwired: 1 in, 1 out]
  }
  n47 = node-c288(w45) -> ()  [unwired: 1 out]
  n48 = property on="Re-check HW connection" class="Bool"(error in=w58, "DisabledEnum"=T12."Disabled and Grayed Out" ("Disabled")) -> (error out=w35:errorcluster)  [unwired: 1 in, 1 out]
  n49 = timed-loop "In this loop raw data from the device is obtained and TTLs are fired" {
    tunnel: w64 -> [w148]
    tunnel: w35 -> [w147]
    tunnel: w17 -> [w127]
    tunnel: w1 -> [w152]
    timing: w57 -> [_]
    timing-out: [_] -> w56
    stop <- w129 stop-if-true
    # "In this loop raw data from the device is obtained and TTLs are fired"
    n50 = node-c288() -> (w146:i64)  [unwired: 1 in]
    n51 = Unbundle By Name(w127) -> ("Complete stop"=w136:refnum<notifier>, "Recording now"=w135:refnum<notifier>, "Has been recorded"=w134:refnum<notifier>)
    n52 = disable-structure shown="Disabled" {
      disable-tunnel: w146 -> [w184 _]
      frame Disabled {
        n53 = Build Array(w184) -> (w182:i64[])
        n54 = call "FL_Last_N_Samples_1D.vi"("BufferLengthSamples"=u32 500, "Input Array"=w182) -> ("Output Array"=w183:dbl[])
        n55 = call <vilib>:"Std Deviation and Variance.vi"("X"=w183) -> ("mean"=→"mean":dbl, "standard deviation"=→"standard deviation":dbl)  [unwired: 1 in, 1 out]
      }
      frame Enabled {
      }
    }
    n56 = property on="Start/Stop out pulses config" class="DigNum (strict)"() -> ("Value"=w149:u32)  [unwired: 2 in, 2 out]
    n57 = Get Notifier Status(notifier=w134) -> (current notification=w133:bool)  [unwired: 1 in, 4 out]
    n58 = Get Notifier Status(notifier=w136) -> (current notification=w129:bool)  [unwired: 1 in, 4 out]
    n59 = Get Notifier Status(notifier=w135) -> (current notification=w131:bool)  [unwired: 1 in, 4 out]
    n60 = Not(x=w131) -> (.not. x?=w130:bool)
    n61 = Greater Than 0?(x=w149) -> (x > 0?=w150:bool)
    n62 = And(x=w130, y=w133) -> (x .and. y?=w132:bool)
    n63 = case "Inside this case structure TTL can be fired at the start of the recording" shown="True" w131 {
      tunnel: w150 -> [_ w198]
      tunnel: w147 -> [w187 w197]
      tunnel: [w187 w196] -> w153
      tunnel: w148 -> [w188 w195]
      tunnel: [w188 w194] -> w155
      tunnel: [w186 w193] -> w154
      tunnel: w152 -> [w186 w192]
      tunnel: w149 -> [_ w191]
      frame False {
        n64 = First Call?() -> (First Call?: T/F=w185:bool)
        n65 = case shown="True" w185 {
          frame False {
          }
          frame True {
            n66 = Get Date/Time In Seconds() -> (seconds since 1Jan1904=w189:timestamp)
            n67 = global write "SW_Globals.vi" "Recording start timestamp"(w189) -> ()
          }
        }
      }
      frame True {
        n68 = property on="Start TTL is fired" class="Bool (strict)"() -> ("Value"=w190:bool)  [unwired: 2 in, 2 out]
        n69 = case shown="False" w190 {
          tunnel: w198 -> [w215 _]
          tunnel: w197 -> [w214 w257]
          tunnel: [w199 w257] -> w196
          tunnel: w195 -> [w213 w256]
          tunnel: [w212 w256] -> w194
          tunnel: [w210 w255] -> w193
          tunnel: w192 -> [w211 w255]
          tunnel: w191 -> [w202 _]
          tunnel: w191 -> [w201 _]
          frame False {
            n70 = flat-sequence {
              tunnel: w211 -> [w228]
              tunnel: w213 -> [w229]
              tunnel: w214 -> [w226]
              tunnel: w215 -> [w227]
              tunnel: [w227] -> w209
              tunnel: [w226] -> w208
              tunnel: [w229] -> w207
              tunnel: [w228] -> w206
              tunnel: w201 -> [w216]
              tunnel: [w234] -> w205
              tunnel: [w239] -> w204
              tunnel: [w238] -> w203
              tunnel: w209 -> [w231]
              tunnel: w208 -> [w237]
              tunnel: w207 -> [w236]
              tunnel: w206 -> [w240]
              tunnel: w202 -> [w230]
              tunnel: [w251] -> w199
              tunnel: [w253] -> w210
              tunnel: [w254] -> w212
              tunnel: w203 -> [w251]
              tunnel: w204 -> [w253]
              tunnel: w205 -> [w254]
              frame #0 {
                n71 = Number To Boolean Array(number=w216) -> (Boolean array=w220:bool[])
                n72 = Index Array(array=w220, index=3) -> (element=w222:bool)
                n73 = Index Array(array=w220, index=2) -> (element=w223:bool)
                n74 = Index Array(array=w220, index=1) -> (element=w224:bool)
                n75 = Index Array(array=w220, index=0) -> (element=w225:bool)
                n76 = property on="TTL IO 4 (recording)" class="Bool (strict)"("Value"=w222) -> ()  [unwired: 2 in, 2 out]
                n77 = property on="TTL IO 3 (recording)" class="Bool (strict)"("Value"=w223) -> ()  [unwired: 2 in, 2 out]
                n78 = property on="TTL IO 2 (recording)" class="Bool (strict)"("Value"=w224) -> ()  [unwired: 2 in, 2 out]
                n79 = property on="TTL IO 1 (recording)" class="Bool (strict)"("Value"=w225) -> ()  [unwired: 2 in, 2 out]
              }
              frame #1 {
                n80 = call "SW_Fire_TTL_at_start_universal.vi"("TTL port(s) config to fire"=w230, "TTL pulse length, ms"=100.0, "error in (no error)"=w237, "Serial Port In"=w236, "Close VISA (T)"=FALSE, "Start/stop signaling (F)"=w231) -> ("error out"=w235:errorcluster, "Serial Port Out"=w234:refnum<visa-resource-name>)  [unwired: 3 in, 1 out]
                n81 = Flush Queue(queue=w240, error in (no error)=w235) -> (queue out=w239:refnum<queue>, error out=w238:errorcluster)  [unwired: 1 out]
              }
              frame #2 {
                n82 = Get Date/Time In Seconds() -> (seconds since 1Jan1904=w252:timestamp)
                n83 = Number To Boolean Array(number=u32 0) -> (Boolean array=w247:bool[])
                n84 = global write "SW_Globals.vi" "Recording start timestamp"(w252) -> ()
                n85 = Index Array(array=w247, index=2) -> (element=w244:bool)
                n86 = Index Array(array=w247, index=1) -> (element=w243:bool)
                n87 = Index Array(array=w247, index=0) -> (element=w242:bool)
                n88 = Index Array(array=w247, index=3) -> (element=w245:bool)
                n89 = property on="TTL IO 3 (recording)" class="Bool (strict)"("Value"=w244) -> ()  [unwired: 2 in, 2 out]
                n90 = property on="TTL IO 2 (recording)" class="Bool (strict)"("Value"=w243) -> ()  [unwired: 2 in, 2 out]
                n91 = property on="TTL IO 1 (recording)" class="Bool (strict)"("Value"=w242) -> ()  [unwired: 2 in, 2 out]
                n92 = property on="TTL IO 4 (recording)" class="Bool (strict)"("Value"=w245) -> ()  [unwired: 2 in, 2 out]
              }
            }
            n93 = property on="Start TTL is fired" class="Bool (strict)"(error in=w199, "Value"=TRUE ("Start TTL is fired")) -> ()  [unwired: 1 in, 2 out]
          }
          frame True {
          }
        }
      }
    }
    n94 = Or(x=w132, y=w129) -> (x .or. y?=w156:bool)
    n95 = disable-structure shown="Disabled" {
      disable-tunnel: w138 -> [w178 _]
      disable-tunnel: w137 -> [w177 _]
      frame Disabled {
        n96 = Subtract(x=w178, y=w177) -> (x-y=w172:dbl)
        n97 = Multiply(x=1000.0, y=w172) -> (x*y=w170:dbl)
        n98 = Build Array(w170) -> (w171:dbl[])
        n99 = call "FL_Last_N_Samples_1D.vi"("BufferLengthSamples"=u32 1000, "Input Array"=w171) -> ("Output Array"=w173:dbl[])
        n100 = call <vilib>:"Std Deviation and Variance.vi"("X"=w173) -> ("mean"=→"Time per sample mean":dbl, "standard deviation"=→"Time per sample SD":dbl)  [unwired: 1 in, 1 out]
      }
      frame Enabled {
      }
    }
    n101 = disable-structure shown="Disabled" {
      disable-tunnel: w127 -> [w165 _]
      frame Disabled {
        n102 = Unbundle By Name(w165) -> ("Data acquisition status"=w164:refnum<notifier>, "Play/Pause status"=w162:refnum<notifier>)
        n103 = Get Notifier Status(notifier=w164) -> (current notification=→"DAQ status":string)  [unwired: 1 in, 4 out]
        n104 = Get Notifier Status(notifier=w162) -> (current notification=→"PP status":string)  [unwired: 1 in, 4 out]
      }
      frame Enabled {
      }
    }
    n105 = flat-sequence {
      tunnel: w153 -> [w259]
      tunnel: w154 -> [w260]
      tunnel: w155 -> [w261]
      tunnel: w127 -> [w262]
      tunnel: [w262] -> w145
      tunnel: [w261] -> w144
      tunnel: [w260] -> w143
      tunnel: [w259] -> w142
      tunnel: [w258] -> w137
      tunnel: w145 -> [w268]
      tunnel: w144 -> [w265]
      tunnel: w143 -> [w264]
      tunnel: w142 -> [w263]
      tunnel: [w269] -> w141
      tunnel: [w267] -> w140
      tunnel: [w266] -> w139
      tunnel: [w271] -> w159
      tunnel: [w272] -> w160
      tunnel: [w273] -> _
      tunnel: w141 -> [w273]
      tunnel: w140 -> [w272]
      tunnel: w139 -> [w271]
      tunnel: [w270] -> w138
      frame #0 {
        n106 = call <vilib>:"High Resolution Relative Seconds.vi"() -> ("relative seconds"=w258:dbl)
      }
      frame #1 {
        n107 = call "HW_Stream_raw_data_enq.vi"("error in"=w263, "Queue in"=w264, "Data flow controls in"=w268, "VISA resource name in"=w265) -> ("error out"=w266:errorcluster, "Data flow controls out"=w269:T17, "VISA resource name out"=w267:refnum<visa-resource-name>)  [unwired: 4 in, 1 out]
      }
      frame #2 {
        n108 = call <vilib>:"High Resolution Relative Seconds.vi"() -> ("relative seconds"=w270:dbl)
      }
    }
    n109 = case "Inside this case structure TTL can be fired at the end of the recording" shown="True" w156 {
      selector: w156 -> [w298 w304]
      tunnel: w160 -> [w299 w307]
      tunnel: [w300 w309] -> w158
      tunnel: w159 -> [w300 w308]
      tunnel: [w299 w306] -> w157
      tunnel: w150 -> [_ w305]
      tunnel: [w298 w304] -> w151
      tunnel: w149 -> [_ w303]
      tunnel: w149 -> [_ w302]
      frame False {
      }
      frame True {
        n110 = property on="Stop TTL is fired" class="Bool (strict)"() -> ("Value"=w301:bool)  [unwired: 2 in, 2 out]
        n111 = case shown="False" w301 {
          tunnel: [w311 w357] -> w309
          tunnel: w308 -> [w322 w357]
          tunnel: w307 -> [w321 w356]
          tunnel: [w320 w356] -> w306
          tunnel: w305 -> [w319 _]
          tunnel: w303 -> [w312 _]
          tunnel: w302 -> [w313 _]
          frame False {
            n112 = flat-sequence {
              tunnel: w319 -> [w334]
              tunnel: w321 -> [w335]
              tunnel: w322 -> [w333]
              tunnel: [w333] -> w316
              tunnel: [w335] -> w315
              tunnel: [w334] -> w314
              tunnel: w313 -> [w323]
              tunnel: [w343] -> w318
              tunnel: [w342] -> w317
              tunnel: w316 -> [w340]
              tunnel: w315 -> [w337]
              tunnel: w314 -> [w338]
              tunnel: w312 -> [w336]
              tunnel: [w355] -> w320
              tunnel: [w354] -> w311
              tunnel: w318 -> [w354]
              tunnel: w317 -> [w355]
              frame #0 {
                n113 = Number To Boolean Array(number=w323) -> (Boolean array=w329:bool[])
                n114 = Index Array(array=w329, index=3) -> (element=w327:bool)
                n115 = Index Array(array=w329, index=2) -> (element=w326:bool)
                n116 = Index Array(array=w329, index=1) -> (element=w325:bool)
                n117 = Index Array(array=w329, index=0) -> (element=w324:bool)
                n118 = property on="TTL IO 4 (recording)" class="Bool (strict)"("Value"=w327) -> ()  [unwired: 2 in, 2 out]
                n119 = property on="TTL IO 3 (recording)" class="Bool (strict)"("Value"=w326) -> ()  [unwired: 2 in, 2 out]
                n120 = property on="TTL IO 2 (recording)" class="Bool (strict)"("Value"=w325) -> ()  [unwired: 2 in, 2 out]
                n121 = property on="TTL IO 1 (recording)" class="Bool (strict)"("Value"=w324) -> ()  [unwired: 2 in, 2 out]
              }
              frame #1 {
                n122 = call "SW_Fire_TTL_at_stop_universal.vi"("TTL port(s) config to fire"=w336, "TTL pulse length, ms"=200.0, "error in (no error)"=w340, "Serial Port In"=w337, "Close VISA (T)"=FALSE, "Start/stop signaling (F)"=w338) -> ("error out"=w343:errorcluster, "Serial Port Out"=w342:refnum<visa-resource-name>)  [unwired: 3 in, 1 out]
              }
              frame #2 {
                n123 = Number To Boolean Array(number=u32 0) -> (Boolean array=w347:bool[])
                n124 = Index Array(array=w347, index=2) -> (element=w350:bool)
                n125 = Index Array(array=w347, index=1) -> (element=w351:bool)
                n126 = Index Array(array=w347, index=0) -> (element=w352:bool)
                n127 = Index Array(array=w347, index=3) -> (element=w349:bool)
                n128 = property on="TTL IO 3 (recording)" class="Bool (strict)"("Value"=w350) -> ()  [unwired: 2 in, 2 out]
                n129 = property on="TTL IO 2 (recording)" class="Bool (strict)"("Value"=w351) -> ()  [unwired: 2 in, 2 out]
                n130 = property on="TTL IO 1 (recording)" class="Bool (strict)"("Value"=w352) -> ()  [unwired: 2 in, 2 out]
                n131 = property on="TTL IO 4 (recording)" class="Bool (strict)"("Value"=w349) -> ()  [unwired: 2 in, 2 out]
              }
            }
            n132 = property on="Stop TTL is fired" class="Bool (strict)"(error in=w311, "Value"=TRUE ("Start/Stop TTL is fired")) -> ()  [unwired: 1 in, 2 out]
          }
          frame True {
          }
        }
      }
    }
    n133 = case shown="True" w151 {
      tunnel: w157 -> [w280 w283]
      tunnel: w158 -> [w279 w284]
      tunnel: [w280 w281] -> w128
      tunnel: [w279 w282] -> w126
      frame False {
      }
      frame True {
        n134 = First Call?() -> (First Call?: T/F=w285:bool)
        n135 = case shown="True" w285 {
          tunnel: w284 -> [w286 w294]
          tunnel: w283 -> [w287 w293]
          tunnel: [w287 w289] -> w281
          tunnel: [w286 w291] -> w282
          frame False {
          }
          frame True {
            w288 = T18 16 items=["Flush Receive Buffer"=16, "Write Transmit Buffer to Device"=32, "Flush Receive Buffer (No I/O)"=64, "Flush Transmit Buffer"=128] ("Mask")
            n136 = Concatenate Strings("SYNC=0" ("string"), "\r") -> (w297:string)
            n137 = VISA Write(VISA resource name=w293, write buffer=w297, error in (no error)=w294) -> (VISA resource name out=w290:refnum<visa-resource-name>, error out=w292:errorcluster)  [unwired: 1 out]
            n138 = VISA Flush I/O Buffer(VISA resource name=w290, mask (16)=w288, error in (no error)=w292) -> (VISA resource name out=w289:refnum<visa-resource-name>, error out=w291:errorcluster)
          }
        }
      }
    }
    n139 = case shown="True" w129 {
      tunnel: w127 -> [_ w168]
      tunnel: w126 -> [_ w167]
      tunnel: w128 -> [_ w166]
      frame False {
      }
      frame True {
        n140 = call "HW_Stop_acq_and_close_VISA.vi"("error in"=w167, "Data flow controls in"=w168, "VISA resource name in"=w166) -> ()  [unwired: 2 out]
      }
    }
    n141 = node-c288(w126) -> ()  [unwired: 1 out]
  }
  n142 = case shown="False" w38 {
    frame True {
      w358 = T12."Enabled" ("Disabled")
      n143 = global read "SW_Globals.vi" "IO inversion config."() -> (w359:u16)
      n144 = global read "SW_Globals.vi" "VISA resource name"() -> (w361:refnum<visa-resource-name>)
      n145 = global read "SW_Globals.vi" "IO ports config"() -> (w360:bool[])
      n146 = property on="Load settings" class="Bool (strict)"("DisabledEnum"=w358) -> ()  [unwired: 2 in, 2 out]
      n147 = call "HW_Set_IO_Dir_on_ECU.vi"("IO ports config"=w360, "VISA resource name"=w361, "IO inversion config."=w359) -> ()  [unwired: 1 in, 2 out]
      n148 = property on="Cage diameter, mm" class="Ring (strict)"("DisabledEnum"=w358) -> ()  [unwired: 2 in, 2 out]
      n149 = property on="Set IO config" class="Bool"("DisabledEnum"=w358) -> ()  [unwired: 2 in, 2 out]
      n150 = property on="Starting angle MIDFIELD" class="DigNum (strict)"("DisabledEnum"=w358) -> ()  [unwired: 2 in, 2 out]
      n151 = property on="N segments MIDFIELD" class="DigNum (strict)"("DisabledEnum"=w358) -> ()  [unwired: 2 in, 2 out]
      n152 = property on="Radius, mm MIDFIELD" class="DigNum (strict)"("DisabledEnum"=w358) -> ()  [unwired: 2 in, 2 out]
      n153 = property on="Starting angle BORDER" class="DigNum (strict)"("DisabledEnum"=w358) -> ()  [unwired: 2 in, 2 out]
      n154 = property on="N segments BORDER" class="DigNum (strict)"("DisabledEnum"=w358) -> ()  [unwired: 2 in, 2 out]
      n155 = property on="Radius, mm CENTER" class="DigNum (strict)"("DisabledEnum"=w358) -> ()  [unwired: 2 in, 2 out]
      n156 = property on="Start Tracking button" class="Bool"("DisabledEnum"=w358) -> ()  [unwired: 2 in, 2 out]
      n157 = property on="Reset stimuli" class="Bool (strict)"("DisabledEnum"=w358) -> ()  [unwired: 2 in, 2 out]
      n158 = property on="Reset regions" class="Bool (strict)"("DisabledEnum"=w358) -> ()  [unwired: 2 in, 2 out]
      n159 = property on="Zone-based stimulus setup" class="RadioBtnsControl (strict)"("DisabledEnum"=w358) -> ()  [unwired: 2 in, 2 out]
      n160 = property on="Set advanced stimulus" class="Bool (strict)"("DisabledEnum"=w358) -> ()  [unwired: 2 in, 2 out]
    }
    frame False {
      w362 = T12."Disabled and Grayed Out" ("Disabled")
      n161 = disable-structure shown="Disabled" {
        disable-tunnel: w362 -> [w363 _]
        frame Disabled {
          n162 = property on="Load settings" class="Bool (strict)"("DisabledEnum"=w363) -> ()  [unwired: 2 in, 2 out]
        }
        frame Enabled {
        }
      }
      n163 = property on="Set advanced stimulus" class="Bool (strict)"("DisabledEnum"=w362) -> ()  [unwired: 2 in, 2 out]
      n164 = property on="Cage diameter, mm" class="Ring (strict)"("DisabledEnum"=w362) -> ()  [unwired: 2 in, 2 out]
      n165 = property on="Set IO config" class="Bool"("DisabledEnum"=w362) -> ()  [unwired: 2 in, 2 out]
      n166 = property on="Starting angle MIDFIELD" class="DigNum (strict)"("DisabledEnum"=w362) -> ()  [unwired: 2 in, 2 out]
      n167 = property on="N segments MIDFIELD" class="DigNum (strict)"("DisabledEnum"=w362) -> ()  [unwired: 2 in, 2 out]
      n168 = property on="Radius, mm MIDFIELD" class="DigNum (strict)"("DisabledEnum"=w362) -> ()  [unwired: 2 in, 2 out]
      n169 = property on="Starting angle BORDER" class="DigNum (strict)"("DisabledEnum"=w362) -> ()  [unwired: 2 in, 2 out]
      n170 = property on="N segments BORDER" class="DigNum (strict)"("DisabledEnum"=w362) -> ()  [unwired: 2 in, 2 out]
      n171 = property on="Radius, mm CENTER" class="DigNum (strict)"("DisabledEnum"=w362) -> ()  [unwired: 2 in, 2 out]
      n172 = property on="Start Tracking button" class="Bool"("DisabledEnum"=w362) -> ()  [unwired: 2 in, 2 out]
      n173 = property on="Reset stimuli" class="Bool (strict)"("DisabledEnum"=w362) -> ()  [unwired: 2 in, 2 out]
      n174 = property on="Reset regions" class="Bool (strict)"("DisabledEnum"=w362) -> ()  [unwired: 2 in, 2 out]
      n175 = property on="Zone-based stimulus setup" class="RadioBtnsControl (strict)"("DisabledEnum"=w362) -> ()  [unwired: 2 in, 2 out]
      n176 = property on="Set advanced stimulus" class="Bool (strict)"("DisabledEnum"=w362) -> ()  [unwired: 2 in, 2 out]
    }
  }
  n177 = node-c288(w56) -> ()  [unwired: 1 out]
  n178 = node-c288(w18, i64 139 ("Period"), 100 ("Priority")) -> (w54:T13)  [unwired: 1 in]
  n179 = timed-loop "This loop is used only for data loading purposes (that is why it is made relatively slow)" {
    tunnel: w17 -> [w368]
    timing: w54 -> [_]
    timing-out: [_] -> w53
    stop <- w365 stop-if-true
    n180 = node-c288() -> ()  [unwired: 1 in, 1 out]
    n181 = Unbundle By Name(w368) -> ("Has been recorded"=w367:refnum<notifier>, "(Final) Data file is saved"=w374:refnum<notifier>, "Data loaded"=w373:refnum<notifier>, "Complete stop"=w366:refnum<notifier>)
    n182 = Get Notifier Status(notifier=w367) -> (current notification=w370:bool)  [unwired: 1 in, 4 out]
    n183 = Get Notifier Status(notifier=w374) -> (current notification=w372:bool)  [unwired: 1 in, 4 out]
    n184 = Get Notifier Status(notifier=w373) -> (current notification=w369:bool)  [unwired: 1 in, 4 out]
    n185 = Get Notifier Status(notifier=w366) -> (current notification=w365:bool)  [unwired: 1 in, 4 out]
    n186 = Not(x=w369) -> (.not. x?=w371:bool)
    n187 = Compound Arithmetic op=AND(w370, w372, w371) -> (w364:bool)
    n188 = case shown="True" w364 {
      tunnel: w368 -> [_ w502]
      frame False {
      }
      frame True {
        w417 = FALSE
        w423 = T12."Disabled and Grayed Out" ("Disabled")
        w446 = 7
        # "Y coord"
        # "X coord"
        # "Background color"
        # "Histogram"
        # "Diagram with zones"
        # "Diagram no zones"
        n189 = call <vilib>:"Set Busy.vi"() -> ("error out"=w377:errorcluster)  [unwired: 10 in, 1 out]
        n190 = property on="Show heatmap (analysis)" class="Bool (strict)"(error in=w377, "DisabledEnum"=w423, "Val(Sgnl)"=w417) -> (error out=w422:errorcluster)  [unwired: 1 in, 1 out]
        n191 = property on="Show full track (analysis)" class="Bool (strict)"("DisabledEnum"=w423, "Val(Sgnl)"=w417) -> (error out=w421:errorcluster)  [unwired: 2 in, 1 out]
        n192 = property on="Zones (analysis)" class="Bool (strict)"("DisabledEnum"=w423, "Val(Sgnl)"=w417) -> (error out=w420:errorcluster)  [unwired: 2 in, 1 out]
        n193 = property on="Play/Pause" class="Bool (strict)"("DisabledEnum"=w423) -> (error out=w419:errorcluster)  [unwired: 2 in, 1 out]
        n194 = Merge Errors(w422, w421, w420, w419) -> (w418:errorcluster)
        n195 = global read "SW_Globals.vi" "Cluster of paths"() -> (w382:T22)
        n196 = property on="Data loading progress" class="Slide (strict)"(error in=w418, "DisabledEnum"=T12."Disabled" ("Disabled"), "Value"=0.0 ("Data loading progress")) -> (error out=w500:errorcluster)  [unwired: 1 in, 1 out]
        n197 = Unbundle By Name(w382) -> ("Path to TDMS file"=w397:path)
        n198 = control-ref of="Data loading progress"() -> (w503:refnum<vi>)
        n199 = property on="Play/Pause" class="Bool (strict)"(error in=w500, "DisabledEnum"=T12."Disabled and Grayed Out" ("Disabled")) -> (error out=w498:errorcluster)  [unwired: 1 in, 1 out]
        n200 = call <vilib>:"Get File Extension.vi"("file"=w397) -> ("lowercase file extension"=w396:string)  [unwired: 6 in, 4 out]
        n201 = Equal?(x=w396, y="tdms") -> (x = y?=w393:bool)
        n202 = case shown="True" w393 {
          tunnel: w503 -> [w538 w546]
          tunnel: w502 -> [w540 w545]
          tunnel: w498 -> [w537 w544]
          tunnel: [w536 w543] -> w460
          tunnel: [_ w542] -> w415
          tunnel: w382 -> [w539 w541]
          tunnel: [w535 _] -> w392
          frame False {
            # "Load CSV"
            n203 = call "SW_Load_data_for_Analysis.vi"("Data flow controls"=w540, "Cluster of paths input"=w539, "Progress bar reference"=w538, "error in (no error)"=w537) -> ("Loaded data"=w535:T23, "error out"=w536:errorcluster)  [unwired: 3 in, 11 out]
          }
          frame True {
            # "Load TDMS"
            n204 = call "SW_Load_data_for_Analysis_from_TDMS.vi"("error in (no error)"=w544, "Progress bar reference"=w546, "Cluster of paths input"=w541, "Data flow controls"=w545) -> ("error out"=w543:errorcluster, "Loaded data"=w542:T24)  [unwired: 3 in, 3 out]
          }
        }
        n205 = case shown="True" w393 {
          tunnel: w415 -> [_ w534]
          tunnel: [w511 w533] -> w391
          tunnel: [w526 w532] -> w414
          tunnel: [w525 w531] -> w413
          tunnel: [w524 w530] -> w412
          tunnel: [w513 w529] -> w408
          tunnel: [w523 w528] -> w405
          tunnel: [w512 w527] -> w399
          tunnel: w392 -> [w522 _]
          frame False {
            n206 = Unbundle By Name(w522) -> ("Absolute timestamp"=w525:dbl[], "Relative timestamp"=w524:dbl[], "Zones preference array (loaded)"=w523:dbl[][], "Stimulus presets array (loaded)"=w526:T7, "Acquisition settings cluster out"=w511:T25, "X coord"=w521:dbl[], "Y coord"=w520:dbl[], "alpha rot. angle"=w519:dbl[], "alpha rot. angle"=w518:dbl[], "Current zone"=w515:dbl[], "TTL inputs"=w517:u8[], "TTL outputs"=w516:u8[])
            n207 = To Unsigned Byte Integer(number=w515) -> (unsigned 8bit integer=w514:u8[])
            n208 = Build Array(w521, w520, w519, w518) -> (w512:dbl[][])
            n209 = Build Array(w514, w517, w516) -> (w513:u8[][])
          }
          frame True {
            n210 = Unbundle By Name(w534) -> ("Absolute timestamp (DBL)"=w531:dbl[], "Relative timestamp (DBL)"=w530:dbl[], "Zones normalized allocation array"=w528:dbl[][], "Coordinates and speed"=w527:dbl[][], "Current zone and TTLs"=w529:u8[][], "Stimulus presets array"=w532:T7, "Acquisition settings cluster out"=w533:T25)
          }
        }
        "Relative timestamp (rec)" <- w412
        "Absolute timestamp (rec)" <- w413
        "Zones preference array (loaded)" <- w405
        n211 = Index Array "TTL Inputs"(array=w408, index (row)=1) -> (element=→"TTL inputs":u8[])  [unwired: 1 in]
        n212 = Index Array "TTL Outputs"(array=w408, index (row)=2) -> (element=→"TTL outputs":u8[])  [unwired: 1 in]
        n213 = Index Array "X coord"(array=w399, index (row)=0) -> (element=w403:dbl[])  [unwired: 1 in]
        "X coord" <- w403
        n214 = Index Array "Current zone"(array=w408, index (row)=0) -> (element=→"Current zone":u8[])  [unwired: 1 in]
        n215 = Index Array "Y coord"(array=w399, index (row)=1) -> (element=w401:dbl[])  [unwired: 1 in]
        "Y coord" <- w401
        n216 = Unbundle By Name(w391) -> ("Twisted neck"=w390:bool, "Offset H."=w389:sgl, "Name prefix"=w388:string, "Stop at"=w387:dbl, "\"Stop at\" enabled"=w386:bool)
        n217 = property on="Data loading progress" class="Slide (strict)"(error in=w460, "DisabledEnum"=T12."Disabled and Grayed Out" ("Disabled")) -> (error out=w427:errorcluster)  [unwired: 1 in, 1 out]
        n218 = Index Array "alpha"(array=w399, index (row)=2) -> (element=→"alpha rot. angle":dbl[])  [unwired: 1 in]
        n219 = property on="Twisted neck" class="Bool (strict)"("Value"=w390) -> ()  [unwired: 2 in, 2 out]
        n220 = property on="\"Stop at\" enabled" class="Bool (strict)"("Value"=w386) -> ()  [unwired: 2 in, 2 out]
        n221 = property on="Bridge horizontal offset" class="DigNum (strict)"("Value"=w389) -> ()  [unwired: 2 in, 2 out]
        n222 = property on="Name Prefix" class="Str"("Value"=w388) -> ()  [unwired: 2 in, 2 out]
        n223 = property on="Stop record at" class="DigNum (strict)"("Value"=w387) -> ()  [unwired: 2 in, 2 out]
        n224 = for {
          tunnel: w414 -> [w632] mode=indexing
          tunnel: [w630] -> w384 mode=indexing if=w629
          i -> [w631]
          n225 = Unbundle By Name(w632) -> ("Stim. has been set"=w629:bool)
          n226 = To Unsigned Byte Integer(number=w631) -> (unsigned 8bit integer=w630:u8)
        }
        n227 = Unbundle By Name(w391) -> ("Bridge V. offset"=w416:sgl, "Bridge swap"=→"Bridge swap (analysis)":bool, "Cage diameter, mm"=w468:u16, "N segments BORDER"=w467:u8, "Starting angle BORDER"=w466:i16, "N segments MIDFIELD"=w465:u8, "Starting angle MIDFIELD"=w464:i16, "Radius, mm MIDFIELD"=w463:u16, "Radius, mm CENTER"=w462:u16, "Researcher name"=w488:string)
        "Bridge Vertical offset (analysis)" <- w416
        n228 = Array Max & Min(array=w412) -> (max value=w495:dbl, max index (indices)=→"Index of the last recorded timepoint":i32, min value=w494:dbl)  [unwired: 1 out]
        n229 = property on="Bridge offset" class="DigNum (strict)"("Value"=w416) -> ()  [unwired: 2 in, 2 out]
        n230 = Concatenate Strings("Recorded by " ("string"), w488) -> (→"Recorded by":string)
        n231 = Compound Arithmetic op=unknown(w467, w465, u32 1 ("value")) -> (w476:u32)
        n232 = Round To Nearest(number=w494) -> (nearest integer value=w492:dbl)
        n233 = global write "SW_Globals.vi" "Active segments amount"(w476) -> ()
        n234 = Bundle By Name(cluster=T20 {"Amount of border segments"=8, "Border segments starting angle"=0, "Amount of midfield segments"=4, "Midfield segments starting angle"=0, "Midfield segments outer radius, mm"=60, "Amount of central segments"=1, "Center segment outer radius, mm"=30, "Diameter of the cage, mm"=180, "R-gap between segments, mm"=10} ("Input cluster of parameters"), "Diameter of the cage, mm"=w468, "Amount of border segments"=w467, "Border segments starting angle"=w466, "Amount of midfield segments"=w465, "Midfield segments starting angle"=w464, "Midfield segments outer radius, mm"=w463, "Center segment outer radius, mm"=w462) -> (w385:T20)
        n235 = property on="Timeline" class="Slide (strict)"(error in=w427, "Scale.Maximum"=w495, "Scale.Minimum"=w492, "Value"=w492, "DisabledEnum"=T12."Disabled and Grayed Out" ("Disabled")) -> (error out=w489:errorcluster)  [unwired: 1 in, 1 out]
        n236 = Unbundle By Name(w382) -> ("Layout picture output path"=w381:path)
        n237 = Increment(x=w476) -> (x+1=w475:u32)
        n238 = property on="Diagram at analysis" class="Pict"(error in=w489) -> (error out=w383:errorcluster, "Bounds"=w470:T19)  [unwired: 1 in, 1 out]
        n239 = flat-sequence "Full track preparation (array of clusters)" {
          tunnel: [w589] -> w434
          tunnel: w424 -> [w599]
          tunnel: w425 -> [w598]
          tunnel: w401 -> [w597]
          tunnel: w403 -> [w595]
          tunnel: [w593] -> w440
          tunnel: [w596] -> w439
          tunnel: w434 -> [w596]
          tunnel: [w628] -> w441
          tunnel: w440 -> [w628]
          tunnel: w439 -> [w627]
          tunnel: [w627] -> w437
          tunnel: [w626] -> w438
          frame #0 {
            n240 = Tick Count (ms)() -> (millisecond timer value=w589:u32)
          }
          frame #1 {
            n241 = Array Size(array=w595) -> (size(s)=w594:i32)
            n242 = for {
              N: w594 -> [w601]
              tunnel: w595 -> [w617]
              tunnel: w597 -> [w616]
              tunnel: [w611] -> w591 mode=indexing
              tunnel: w598 -> [w614]
              tunnel: w599 -> [w610]
              i -> [w602]
              n243 = Increment(x=w602) -> (x+1=w603:i32)
              n244 = Equal?(x=w602, y=w603) -> (x = y?=w604:bool)
              n245 = Quotient & Remainder(x=w602, y=1200) -> (x-y*floor(x/y)=w606:i32)  [unwired: 1 out]
              n246 = Equal To 0?(x=w606) -> (x = 0?=w605:bool)
              n247 = Or(x=w604, y=w605) -> (x .or. y?=w600:bool)
              n248 = Index Array(array=w617, index=w602) -> (element=w608:dbl)
              n249 = Index Array(array=w616, index=w602) -> (element=w609:dbl)
              n250 = case shown="True" w600 {
                tunnel: w602 -> [_ w622]
                tunnel: w601 -> [_ w621]
                frame False {
                }
                frame True {
                  n251 = Increment(x=w622) -> (x+1=w623:i32)
                  n252 = Divide(x=w623, y=w621) -> (x/y=w625:dbl)
                  n253 = Multiply(x=w625, y=20.0) -> (x*y=w620:dbl)
                  n254 = Add(x=40.0, y=w620) -> (x+y=w618:dbl)
                  n255 = local write "Data loading progress"(w618) -> ()
                }
              }
              n256 = Multiply(x=w614, y=w608) -> (x*y=w613:dbl)
              n257 = Multiply(x=w614, y=w609) -> (x*y=w612:dbl)
              n258 = Bundle(w613, w612) -> (w615:cluster{dbl, dbl})  [unwired: 1 in]
              n259 = Add(x=w615, y=w610) -> (x+y=w611:cluster{dbl, dbl})
            }
            n260 = Delete From Array(array=w591, length=1, index=0) -> (array with subset deleted=w593:cluster{dbl, dbl}[])  [unwired: 1 out]
          }
          frame #2 {
            n261 = Tick Count (ms)() -> (millisecond timer value=w626:u32)
          }
        }
        n262 = call <vilib>:"Check if File or Folder Exists.vi"("path"=w381) -> ("file or folder exists?"=w380:bool)  [unwired: 8 in, 2 out]
        n263 = Bundle By Name(cluster=T21 {"Minimum"=0.0, "Maximum"=14.0, "Increment"=1.0, "Minor Increment"=1.0, "Start"=0.0} ("X Scale.Range"), "Maximum"=w475) -> (w474:T21)
        n264 = global write "SW_Globals.vi" "Regions to track"(w384) -> ()
        n265 = property on="Diagram at analysis" class="Pict"() -> ("Bounds"=w455:T19)  [unwired: 2 in, 2 out]
        n266 = case shown="False" w380 {
          tunnel: w385 -> [w510 _]
          tunnel: w384 -> [w508 _]
          tunnel: w383 -> [w507 _]
          tunnel: w381 -> [w504 _]
          frame False {
            n267 = call "SW_Generate_Segmented_Plot_v3.vi"("Draw Area Size"=cluster{"Width":dbl, "Height":dbl} {"Width"=1200.0, "Height"=1200.0}, "Regions to mark set"=w508, "Input cluster of parameters"=w510, "Error In"=w507) -> ("Zones layout output"=w506:picture)  [unwired: 6 in, 5 out]
            n268 = call <vilib>:"Picture to Pixmap.vi"("picture"=w506) -> ("image data"=w505:T26)  [unwired: 9 in, 1 out]
            n269 = call <vilib>:"Write PNG File.vi"("image data"=w505, "path to PNG file"=w504) -> ()  [unwired: 8 in, 2 out]
          }
          frame True {
          }
        }
        n270 = control-ref of="Zones allocation array"() -> (w482:refnum<vi>)
        n271 = property on="Zones allocation (normalized) in analysis" class="WFGraph (strict)"("XScale.Range"=w474) -> ()  [unwired: 2 in, 2 out]
        n272 = call "SW_Generate_Segmented_Plot_v3.vi"("Draw Area Size"=w470, "Regions to mark set"=w384, "Input cluster of parameters"=w385, "Error In"=w383) -> ("Zones layout output"=w445:picture, "No zones image"=w443:picture, "Array of the pixel to color correspondences"=w472:u32[][], "Array of the segment to color correspondences"=w473:u32[][], "Cluster of image geometrical and scaling parameters"=w471:T27, "Error Out"=w461:errorcluster)  [unwired: 6 in]
        n273 = control-ref of="Diagram at analysis"() -> (w426:refnum<vi>)
        n274 = global write "SW_Globals.vi" "Diagram"(w445) -> ()
        n275 = Unbundle By Name(w471) -> ("Pixels per mm"=w425:dbl)
        n276 = property class="Arr (strict)"(reference=w482, error in=w461) -> (reference out=w480:refnum<vi>, error out=w479:errorcluster, "Value"=w483:i32[])
        n277 = global write "SW_Globals.vi" "Diagram no zones"(w443) -> ()
        n278 = global write "SW_Globals.vi" "Array of the pixel to color correspondences"(w472) -> ()
        n279 = global write "SW_Globals.vi" "Array of the segment to color correspondences"(w473) -> ()
        n280 = Quotient & Remainder(x=w455, y=T19 {"Width"=2, "Height"=2}) -> (floor(x/y)=w424:T19)  [unwired: 1 out]
        n281 = call <vilib>:"Picture to Pixmap.vi"("picture"=w443) -> ("image data"=w444:T26)  [unwired: 9 in, 1 out]
        n282 = call <vilib>:"Picture to Pixmap.vi"("picture"=w445) -> ("image data"=w459:T26)  [unwired: 9 in, 1 out]
        n283 = call <vilib>:"Unflatten Pixmap.vi"("image data"=w444) -> ("24-bit pixmap"=w442:u32[][])  [unwired: 4 in, 6 out]
        n284 = call <vilib>:"Unflatten Pixmap.vi"("image data"=w459) -> ("24-bit pixmap"=w458:u32[][])  [unwired: 4 in, 6 out]
        n285 = Array Size(array=w483) -> (size(s)=w485:i32)
        n286 = call "SW_Gen_2D_Histogram.vi"("Picture reference in"=w426, "Pixels per mm"=w425, "Y coord array"=w401, "X coord array"=w403, "Bounds"=w424) -> ("8-bit density map"=w378:u8[][], "24-bit pixmap"=w379:u32[][])  [unwired: 4 in, 1 out]
        n287 = local write "Pixels per mm"(w425) -> ()
        n288 = Array Size(array=w379) -> (size(s)=w454:i32[])
        n289 = Initialize Array(0 ("element"), w485) -> (w481:i32[])
        n290 = property class="Arr (strict)"(reference=w480, error in=w479, "Value"=w481) -> ()  [unwired: 2 out]
        n291 = Index Array(array=w454, index=0) -> (element=w450:i32)
        n292 = Index Array(array=w454, index=1) -> (element=w448:i32)
        n293 = Subtract(x=w450, y=w446) -> (x-y=w449:i32)
        n294 = Subtract(x=w448, y=w446) -> (x-y=w447:i32)
        n295 = Index Array(array=w379, index (row)=w449, index (col)=w447) -> (element=w451:u32)
        n296 = Subtract(x=w438, y=w437) -> (x-y=→"Full track preparation":u32)
        n297 = flat-sequence {
          tunnel: w441 -> [w548]
          tunnel: w443 -> [w549]
          tunnel: w445 -> [w550]
          tunnel: [w550] -> w433
          tunnel: [w549] -> w432
          tunnel: [w548] -> w431
          tunnel: [w547] -> w429
          tunnel: w457 -> [w579]
          tunnel: w435 -> [w565]
          tunnel: w433 -> [w551]
          tunnel: w432 -> [w574]
          tunnel: w431 -> [w562]
          tunnel: w378 -> [w554]
          tunnel: [w588] -> w430
          frame #0 {
            n298 = Tick Count (ms)() -> (millisecond timer value=w547:u32)
          }
          frame #1 {
            w563 = T28 {"Width"=2, "Style"=enum."Solid"} ("pen")
            n299 = global read "SW_Globals.vi" "Cluster of paths"() -> (w559:T22)
            n300 = call <vilib>:"Flatten Pixmap.vi"("24-bit pixmap"=w565) -> ("image data"=w553:T26)  [unwired: 10 in]
            n301 = call <vilib>:"Flatten Pixmap.vi"("24-bit pixmap"=w579) -> ("image data"=w552:T26)  [unwired: 10 in]
            n302 = call <vilib>:"Draw Flattened Pixmap.vi"("image data"=w553) -> ("new picture"=w560:picture)  [unwired: 8 in]
            n303 = call <vilib>:"Draw Flattened Pixmap.vi"("image data"=w552) -> ("new picture"=w567:picture)  [unwired: 8 in]
            n304 = Unbundle By Name(w559) -> ("Density map array output path"=w555:path, "Density map picture output path"=w557:path)
            n305 = call <vilib>:"Check if File or Folder Exists.vi"("path"=w557) -> ("file or folder exists?"=w558:bool)  [unwired: 8 in, 2 out]
            n306 = call <vilib>:"Check if File or Folder Exists.vi"("path"=w555) -> ("file or folder exists?"=w556:bool)  [unwired: 8 in, 2 out]
            n307 = call "SW_Make_Track_overlay.vi"("Pen properties"=w563, "Full track array"=w562, "Full trace color"="Full trace color", "Picture in"=w551) -> ("Picture out"=w576:picture)  [unwired: 3 in]
            n308 = call "SW_Make_Track_overlay.vi"("Pen properties"=w563, "Full track array"=w562, "Full trace color"="Full trace color", "Picture in"=w560) -> ("Picture out"=w561:picture)  [unwired: 3 in]
            n309 = call "SW_Make_Track_overlay.vi"("Pen properties"=w563, "Full track array"=w562, "Full trace color"="Full trace color", "Picture in"=w567) -> ("Picture out"=w566:picture)  [unwired: 3 in]
            n310 = call "SW_Make_Track_overlay.vi"("Pen properties"=w563, "Full track array"=w562, "Full trace color"="Full trace color", "Picture in"=w574) -> ("Picture out"=w577:picture)  [unwired: 3 in]
            n311 = global write "SW_Globals.vi" "Density map with zones"(w567) -> ()
            n312 = global write "SW_Globals.vi" "Density map no zones"(w560) -> ()
            n313 = call <vilib>:"Picture to Pixmap.vi"("picture"=w576) -> ("image data"=w575:T26)  [unwired: 9 in, 1 out]
            n314 = call <vilib>:"Picture to Pixmap.vi"("picture"=w561) -> ("image data"=w571:T26)  [unwired: 9 in, 1 out]
            n315 = call <vilib>:"Picture to Pixmap.vi"("picture"=w566) -> ("image data"=w570:T26)  [unwired: 9 in, 1 out]
            n316 = call <vilib>:"Picture to Pixmap.vi"("picture"=w577) -> ("image data"=w578:T26)  [unwired: 9 in, 1 out]
            n317 = call <vilib>:"Draw Flattened Pixmap.vi"("image data"=w575) -> ("new picture"=w573:picture)  [unwired: 8 in]
            n318 = call <vilib>:"Draw Flattened Pixmap.vi"("image data"=w571) -> ("new picture"=w569:picture)  [unwired: 8 in]
            n319 = call <vilib>:"Draw Flattened Pixmap.vi"("image data"=w570) -> ("new picture"=w568:picture)  [unwired: 8 in]
            n320 = call <vilib>:"Draw Flattened Pixmap.vi"("image data"=w578) -> ("new picture"=w572:picture)  [unwired: 8 in]
            n321 = global write "SW_Globals.vi" "Full track with zones"(w573) -> ()
            n322 = global write "SW_Globals.vi" "Full track with no zones"(w572) -> ()
            n323 = global write "SW_Globals.vi" "Density map with zones and full track"(w568) -> ()
            n324 = global write "SW_Globals.vi" "Density map with no zones and with full track"(w569) -> ()
            n325 = case shown="False" w558 {
              tunnel: w557 -> [w583 _]
              tunnel: w552 -> [w582 _]
              frame False {
                n326 = call <vilib>:"Write PNG File.vi"("image data"=w582, "path to PNG file"=w583) -> ()  [unwired: 8 in, 2 out]
              }
              frame True {
              }
            }
            n327 = case shown="False" w556 {
              tunnel: w555 -> [w581 _]
              tunnel: w554 -> [w580 _]
              frame False {
                n328 = call-poly <vilib>:"Write Delimited Spreadsheet.vi"("file path (dialog if empty)"=w581, "2D data"=w580) -> ()  [unwired: 12 in, 2 out]
              }
              frame True {
              }
            }
          }
          frame #2 {
            w587 = T12."Enabled" ("Disabled")
            n329 = local write "Data loading progress"(100.0 ("Data loading progress")) -> ()
            n330 = property on="Zones (analysis)" class="Bool (strict)"("DisabledEnum"=w587) -> ()  [unwired: 2 in, 2 out]
            n331 = property on="Play/Pause" class="Bool (strict)"("DisabledEnum"=w587) -> ()  [unwired: 2 in, 2 out]
            n332 = property on="Show full track (analysis)" class="Bool (strict)"("DisabledEnum"=w587, "Val(Sgnl)"=TRUE ("Value (Signaling)")) -> (error out=w584:errorcluster)  [unwired: 2 in, 1 out]
            n333 = property on="Show heatmap (analysis)" class="Bool (strict)"("DisabledEnum"=w587) -> ()  [unwired: 2 in, 2 out]
            n334 = Tick Count (ms)() -> (millisecond timer value=w588:u32)
            n335 = call <vilib>:"Unset Busy.vi"("error in (no error)"=w584) -> ()  [unwired: 10 in, 1 out]
          }
        }
        n336 = call "SW_Create_density_overlay.vi"("Background color"=w451, "Density histogram"=w379, "Diagram with zones"=w458, "Diagram no zones"=w442) -> ("Density map with zones"=w457:u32[][], "Density map no zones"=w435:u32[][])
        n337 = Subtract(x=w430, y=w429) -> (x-y=→"Full track plotting":u32)
      }
    }
    n338 = node-c288() -> ()  [unwired: 1 in, 1 out]
  }
  n339 = node-c288(w53) -> ()  [unwired: 1 out]
  n340 = disable-structure shown="Disabled" {
    disable-tunnel: _ -> [w634 _]
    disable-tunnel: _ -> [w633 _]
    frame Disabled {
      n341 = node-c288(w633, i64 499 ("Period"), 800 ("Priority")) -> (w639:T13)
      n342 = timed-loop "Loop where temporary files are transferred to permanent location and data saved" {
        tunnel: w634 -> [w666]
        tunnel: [w651] -> w637
        timing: w639 -> [_]
        timing-out: [_] -> w638
        stop <- w652 stop-if-true
        n343 = node-c288() -> (→"Save iteration duration":i64)  [unwired: 1 in]
        n344 = flat-sequence {
          tunnel: w666 -> [w927]
          tunnel: [w927] -> w665
          tunnel: w665 -> [w928]
          tunnel: [w930] -> w663
          tunnel: [w929] -> w662
          tunnel: [w928] -> w664
          frame #0 {
            n345 = Wait (ms)(milliseconds to wait=u32 521) -> ()  [unwired: 1 out]
          }
          frame #1 {
            n346 = Unbundle By Name(w928) -> ("Path to the latest complete temp file"=w930, "Temp file ready for processing"=w929)
          }
        }
        n347 = Get Notifier Status(notifier=w662) -> (error out=w661:errorcluster)  [unwired: 1 in, 4 out]
        n348 = Get Notifier Status(notifier=w663, error in (no error)=w661) -> (current notification=w657:path)  [unwired: 4 out]
        n349 = feedback-in #1(w657) -> ()
        n350 = feedback #1(path "") -> (w659:path)
        n351 = local read "Starting angle MIDFIELD"() -> (w647:i16)
        n352 = local read "Starting angle BORDER"() -> (w649:i16)
        n353 = local read "N segments MIDFIELD"() -> (w648:u8)
        n354 = local read "Radius, mm MIDFIELD"() -> (w646:u16)
        n355 = local read "N segments BORDER"() -> (w650:u8)
        n356 = Not Equal?(x=w659, y=w657) -> (x != y?=w658:bool)
        n357 = local read "Radius, mm CENTER"() -> (w644:u16)
        n358 = Not Equal?(x=path "", y=w657) -> (x != y?=w656:bool)
        n359 = Bundle By Name(cluster=T29 {"N segments BORDER"=0, "Starting angle BORDER"=0, "N segments MIDFIELD"=0, "Starting angle MIDFIELD"=0, "Radius, mm MIDFIELD"=0, "Amount of central segments"=0, "Radius, mm CENTER"=0} ("output cluster 2"), "N segments BORDER"=w650, "Starting angle BORDER"=w649, "N segments MIDFIELD"=w648, "Starting angle MIDFIELD"=w647, "Radius, mm MIDFIELD"=w646, "Amount of central segments"=u8 1, "Radius, mm CENTER"=w644) -> (w643:T29)
        n360 = And(x=w656, y=w658) -> (x .and. y?=w653:bool)
        n361 = local read "Cage diameter, mm"() -> (w642:u16)
        n362 = global read "SW_Globals.vi" "Cluster of paths"() -> (w667:T22)
        n363 = case shown="True" w653 {
          tunnel: w667 -> [_ w691]
          tunnel: w664 -> [_ w690]
          tunnel: errorcluster {"status"=FALSE, "code"=0, "source"=""} ("error constant") -> [w672 w689]
          tunnel: w653 -> [_ w688]
          tunnel: w657 -> [_ w687]
          tunnel: [FALSE w678] -> w652
          tunnel: [w672 w679] -> w651
          tunnel: w643 -> [_ w682]
          tunnel: w642 -> [_ w681]
          frame False {
          }
          frame True {
            n364 = flat-sequence {
              tunnel: w687 -> [w761]
              tunnel: w688 -> [w760]
              tunnel: w691 -> [w746]
              tunnel: w689 -> [w759]
              tunnel: [w758] -> w695
              tunnel: w690 -> [w757]
              tunnel: [w757] -> w694
              tunnel: [w746] -> w685
              tunnel: w682 -> [w745]
              tunnel: w681 -> [w744]
              tunnel: w695 -> [w901]
              tunnel: [w901] -> w693
              tunnel: [w900] -> w692
              tunnel: w694 -> [w900]
              tunnel: w685 -> [w899]
              tunnel: [w899] -> w684
              tunnel: w693 -> [w909]
              tunnel: w692 -> [w908]
              tunnel: w684 -> [w905]
              tunnel: [w910] -> w676
              tunnel: [w913] -> w675
              tunnel: [w908] -> w674
              tunnel: [w905] -> w673
              tunnel: [w923] -> w683
              tunnel: [w924] -> w677
              tunnel: [w921] -> w680
              tunnel: [w925] -> w686
              tunnel: w676 -> [w925]
              tunnel: w675 -> [w921]
              tunnel: w674 -> [w924]
              tunnel: w673 -> [w923]
              frame #0 {
                n365 = Unbundle By Name(w746) -> ("Density map array output path"=w751:path, "Layout picture output path"=w754:path, "Recording settings output path"=w753:path, "Density map picture output path"=w752:path, "Path to the settings file"=w743:path)
                n366 = case shown="True" "Save files First Call" {
                  selector: "Save files First Call" -> [w762 w775]
                  tunnel: [w765 w878] -> w750
                  tunnel: w761 -> [w765 w878]
                  tunnel: w751 -> [w763 w865]
                  tunnel: w754 -> [_ w863]
                  tunnel: w753 -> [_ w861]
                  tunnel: w752 -> [_ w833]
                  tunnel: w759 -> [w764 w830]
                  tunnel: [w764 w829] -> w749
                  tunnel: [w763 w770] -> w747
                  tunnel: w745 -> [_ w792]
                  tunnel: w744 -> [_ w790]
                  tunnel: w743 -> [_ w810]
                  tunnel: [w762 w775] -> w742
                  frame False {
                  }
                  frame True {
                    w809 = "Vertical offset" ("key")
                    w802 = "Mouse snout orientation swap?" ("key")
                    w776 = "Recording settings" ("key")
                    n367 = Unbundle By Name(w792) -> ("N segments BORDER"=w791:u8, "Starting angle BORDER"=w789:i16, "N segments MIDFIELD"=w788:u8, "Starting angle MIDFIELD"=w787:i16, "Radius, mm MIDFIELD"=w786:u16, "Radius, mm CENTER"=w784:u16)
                    n368 = property on="Save files First Call" class="Bool (strict)"("Value"=FALSE ("Save files First Call")) -> ()  [unwired: 2 in, 2 out]
                    n369 = Bundle By Name(cluster=T20 {"Amount of border segments"=8, "Border segments starting angle"=0, "Amount of midfield segments"=4, "Midfield segments starting angle"=0, "Midfield segments outer radius, mm"=60, "Amount of central segments"=1, "Center segment outer radius, mm"=30, "Diameter of the cage, mm"=180, "R-gap between segments, mm"=10} ("Input cluster of parameters"), "Diameter of the cage, mm"=w790, "Amount of border segments"=w791, "Border segments starting angle"=w789, "Amount of midfield segments"=w788, "Midfield segments starting angle"=w787, "Midfield segments outer radius, mm"=w786, "Center segment outer radius, mm"=w784) -> (w785:T20)
                    n370 = global read "SW_Globals.vi" "Regions to track"() -> (w795:u8[])
                    n371 = Build Array("X1_raw", "Y1_raw", "X2_raw", "Y2_raw", "Absolute_timestamp", "Relative_timestamp", "R", "phi", "alpha", "X", "Y", "w", "Current_zone", "Zones_preference", "TTL_inputs", "TTL_outputs", "Speed_mm_per_s", "Frame_OK") -> (w766:string[])
                    n372 = call-poly <vilib>:"Write Delimited Spreadsheet.vi"("file path (dialog if empty)"=w865, "1D data"=w766, "append to file? (new file:F)"=FALSE, "error in (no error)"=w830) -> ("new file path (Not A Path if cancelled)"=w771:path, "error out"=w768:errorcluster)  [unwired: 10 in]
                    n373 = Set Permissions(7:i16 384 ("permissions"), 8:w768, 11:w771) -> (0:w767:errorcluster, 3:w770:path)  [unwired: 2 in]
                    n374 = call "SW_Generate_Segmented_Plot_v3.vi"("Draw Area Size"=cluster{"Width":dbl, "Height":dbl} {"Width"=1200.0, "Height"=1200.0}, "Regions to mark set"=w795, "Input cluster of parameters"=w785, "Error In"=w767) -> ("Zones layout output"=w796:picture, "Error Out"=w797:errorcluster)  [unwired: 6 in, 4 out]
                    n375 = call <vilib>:"Picture to Pixmap.vi"("picture"=w796) -> ("image data"=w862:T26)  [unwired: 9 in, 1 out]
                    n376 = local read "Current User"() -> (w836:string)
                    n377 = call <vilib>:"Write PNG File.vi"("error in (no error)"=w797, "image data"=w862, "path to PNG file"=w863) -> ("error out"=w843:errorcluster)  [unwired: 7 in, 1 out]
                    n378 = call <vilib>:"Open Config Data.vi"("error in (no error)"=w843, "configuration file path"=w861) -> ("refnum"=w841:T5)  [unwired: 7 in, 2 out]
                    n379 = Strip Path(path=w833) -> (name=w832:string)  [unwired: 1 out]
                    n380 = call <vilib>:"Write Key (String).vi"("section"=w776, "value"=w836, "key"="Researcher", "refnum"=w841) -> ("error out"=w838:errorcluster, "refnum out"=w840:T5)  [unwired: 5 in, 1 out]
                    n381 = Unbundle By Name(w792) -> ("N segments MIDFIELD"=w828:u8, "N segments BORDER"=w827:u8, "Radius, mm CENTER"=w826:u16, "Radius, mm MIDFIELD"=w825:u16, "Starting angle MIDFIELD"=w824:i16, "Starting angle BORDER"=w823:i16)
                    n382 = call <vilib>:"Write Key (String).vi"("section"=w776, "error in (no error)"=w838, "value"=w832, "key"="Track name", "refnum"=w840) -> ("error out"=w837:errorcluster, "refnum out"=w839:T5)  [unwired: 4 in, 1 out]
                    n383 = call <vilib>:"Write Key (I32).vi"("section"=w776, "error in (no error)"=w837, "value"=w828, "key"="Amount of midfield segments", "refnum"=w839) -> ("error out"=w859:errorcluster, "refnum out"=w858:T5)  [unwired: 4 in, 1 out]
                    n384 = call <vilib>:"Write Key (I32).vi"("section"=w776, "error in (no error)"=w859, "value"=w827, "key"="Amount of border segments", "refnum"=w858) -> ("error out"=w855:errorcluster, "refnum out"=w856:T5)  [unwired: 4 in, 1 out]
                    n385 = call <vilib>:"Write Key (I32).vi"("section"=w776, "error in (no error)"=w855, "value"=w826, "key"="Center segment outer radius, mm", "refnum"=w856) -> ("error out"=w852:errorcluster, "refnum out"=w853:T5)  [unwired: 4 in, 1 out]
                    n386 = call <vilib>:"Write Key (I32).vi"("section"=w776, "error in (no error)"=w852, "value"=w825, "key"="Midfield segments outer radius, mm", "refnum"=w853) -> ("error out"=w849:errorcluster, "refnum out"=w850:T5)  [unwired: 4 in, 1 out]
                    n387 = call <vilib>:"Write Key (I32).vi"("section"=w776, "error in (no error)"=w849, "value"=w824, "key"="Midfield segments starting angle", "refnum"=w850) -> ("error out"=w847:errorcluster, "refnum out"=w846:T5)  [unwired: 4 in, 1 out]
                    n388 = call <vilib>:"Write Key (I32).vi"("section"=w776, "error in (no error)"=w847, "value"=w823, "key"="Border segments starting angle", "refnum"=w846) -> ("error out"=w845:errorcluster, "refnum out"=w844:T5)  [unwired: 4 in, 1 out]
                    n389 = local read "Current User"() -> (w801:string)
                    n390 = property on="Bridge offset" class="DigNum (strict)"() -> ("Value"=w808:sgl)  [unwired: 2 in, 2 out]
                    n391 = call <vilib>:"Write Key (I32).vi"("section"=w776, "error in (no error)"=w845, "value"=w790, "key"="Cage diameter, mm", "refnum"=w844) -> ("error out"=w815:errorcluster, "refnum out"=w812:T5)  [unwired: 4 in, 1 out]
                    n392 = call <vilib>:"Open Config Data.vi"("configuration file path"=w810) -> ("error out"=w807:errorcluster, "refnum"=w805:T5)  [unwired: 8 in, 1 out]
                    n393 = property on="Bridge swap" class="Bool (strict)"() -> ("Value"=w803:bool)  [unwired: 2 in, 2 out]
                    n394 = call <vilib>:"Write Key (Double).vi"("use system decimal point (T)"=FALSE, "section"=w801, "error in (no error)"=w807, "value"=w808, "key"=w809, "refnum"=w805) -> ("error out"=w804:errorcluster, "refnum out"=w800:T5)  [unwired: 3 in, 1 out]
                    n395 = call <vilib>:"Write Key (Double).vi"("use system decimal point (T)"=FALSE, "section"=w776, "error in (no error)"=w815, "value"=w808, "key"=w809, "refnum"=w812) -> ("error out"=w814:errorcluster, "refnum out"=w813:T5)  [unwired: 3 in, 1 out]
                    n396 = call <vilib>:"Write Key (Boolean).vi"("section"=w801, "error in (no error)"=w804, "value"=w803, "key"=w802, "refnum"=w800) -> ("error out"=w799:errorcluster, "refnum out"=w798:T5)  [unwired: 4 in, 1 out]
                    n397 = call <vilib>:"Write Key (Boolean).vi"("section"=w776, "error in (no error)"=w814, "value"=w803, "key"=w802, "refnum"=w813) -> ("error out"=w819:errorcluster, "refnum out"=w820:T5)  [unwired: 4 in, 1 out]
                    n398 = call <vilib>:"Close Config Data.vi"("error in (no error)"=w799, "refnum"=w798) -> ()  [unwired: 8 in, 2 out]
                    n399 = property on="Stimulus presets" class="Arr (strict)"(error in=w819) -> (error out=w779:errorcluster, "Value"=w821:T7)  [unwired: 1 in, 1 out]
                    n400 = for {
                      tunnel: w821 -> [w891] mode=indexing
                      tunnel: w820 -> [w884]
                      tunnel: [w888] -> w780
                      tunnel: w776 -> [w879]
                      i -> [w887]
                      n401 = Unbundle By Name(w891) -> ("Stim. has been set"=w889:bool)
                      n402 = Flatten To JSON(anything=w891) -> (JSON string=w890:string, 11:w881:errorcluster)  [unwired: 2 in]
                      n403 = Format Value(string ("")="Zone " ("string"), format string="%02d", value (0)=w887) -> (output string=w882:string)
                      n404 = call <vilib>:"Remove Key.vi"("section"=w879, "error in (no error)"=w881, "key"=w882, "refnum"=w884) -> ("error out"=w880:errorcluster, "refnum out"=w883:T5)  [unwired: 5 in, 1 out]
                      n405 = case shown="False" w889 {
                        tunnel: w890 -> [_ w898]
                        tunnel: w880 -> [_ w897]
                        tunnel: [w892 w896] -> w888
                        tunnel: w882 -> [_ w895]
                        tunnel: w883 -> [w892 w894]
                        tunnel: w879 -> [_ w893]
                        frame False {
                        }
                        frame True {
                          n406 = call <vilib>:"Write Key (String).vi"("section"=w893, "error in (no error)"=w897, "value"=w898, "key"=w895, "refnum"=w894) -> ("refnum out"=w896:T5)  [unwired: 4 in, 2 out]
                        }
                      }
                    }
                    n407 = property on="IO parameters string" class="Str"(error in=w779) -> (error out=w781:errorcluster, "Value"=w782:string)  [unwired: 1 in, 1 out]
                    n408 = call <vilib>:"Write Key (String).vi"("section"=w776, "error in (no error)"=w781, "value"=w782, "key"="IO ports configuration", "refnum"=w780) -> ("error out"=w778:errorcluster, "refnum out"=w777:T5)  [unwired: 4 in, 1 out]
                    n409 = call <vilib>:"Close Config Data.vi"("error in (no error)"=w778, "refnum"=w777) -> ("error out"=w829:errorcluster)  [unwired: 8 in, 1 out]
                  }
                }
                n410 = call-poly <vilib>:"Read Delimited Spreadsheet.vi"("file path (dialog if empty)"=w750, "error in (no error)"=w749) -> ("all rows"=w741:string[][], "error out"=w748:errorcluster)  [unwired: 8 in, 4 out]
                n411 = Array Subset(array=w741, index (row)=1 ("index")) -> (w740:string[][])  [unwired: 3 in]
                n412 = Select(t=w740, s=w742, f=w741) -> (s? t:f=w737:string[][])
                n413 = call-poly <vilib>:"Write Delimited Spreadsheet.vi"("file path (dialog if empty)"=w747, "format (%s)"="%s", "2D data"=w737, "append to file? (new file:F)"=TRUE, "error in (no error)"=w748) -> ("error out"=w758:errorcluster)  [unwired: 9 in, 1 out]
                "Path to the latest saved temp file" <- w761
                "Temp file ready" <- w760
              }
              frame #1 {
                n414 = Wait (ms)(milliseconds to wait=u32 257 ("millisecond multiple")) -> ()  [unwired: 1 out]
              }
              frame #2 {
                n415 = Unbundle By Name(w908) -> ("Recording now"=w904, "Has been recorded"=w903, "Path to the latest complete temp file"=w919, "Temp file ready for processing"=w920)
                n416 = Send Notification(notification=FALSE, notifier=w920, error in (no error)=w909) -> (error out=w918:errorcluster)  [unwired: 1 out]
                n417 = Get Notifier Status(notifier=w919, error in (no error)=w918) -> (current notification=w906:path, error out=w917:errorcluster)  [unwired: 3 out]
                n418 = Delete(path (use dialog)=w906, error in=w917) -> (error out=w912:errorcluster)  [unwired: 3 in, 2 out]
                n419 = Get Notifier Status(notifier=w903, error in (no error)=w912) -> (current notification=w914:bool, error out=w911:errorcluster)  [unwired: 3 out]
                n420 = Get Notifier Status(notifier=w904, error in (no error)=w911) -> (current notification=w916:bool, error out=w910:errorcluster)  [unwired: 3 out]
                n421 = Not(x=w916) -> (.not. x?=w915:bool)
                n422 = And(x=w915, y=w914) -> (x .and. y?=w913:bool)
              }
              frame #3 {
                n423 = Wait (ms)(milliseconds to wait=u32 257 ("millisecond multiple")) -> ()  [unwired: 1 out]
              }
            }
            n424 = case "Case Here data saving will be finalized" shown="True" w680 {
              selector: w680 -> [w697 w710]
              tunnel: w686 -> [w696 w699]
              tunnel: [w697 w710] -> w678
              tunnel: w683 -> [_ w711]
              tunnel: [w696 w707] -> w679
              tunnel: w677 -> [_ w704]
              frame False {
              }
              frame True {
                n425 = Unbundle By Name(w711) -> ("Density map picture output path"=w705:path, "Density map array output path"=w701:path)
                n426 = Set Permissions(7:i16 438 ("permissions"), 8:w699, 11:w701) -> (0:w698:errorcluster, 3:w702:path)  [unwired: 2 in]
                n427 = while {
                  tunnel: w702 -> [w720]
                  tunnel: w705 -> [w718]
                  tunnel: w698 -> [w722]
                  tunnel: [w721] -> w708
                  tunnel: w704 -> [w719]
                  tunnel: [w719] -> w703
                  i -> [w715]
                  stop <- w712 stop-if-true
                  n428 = flat-sequence {
                    tunnel: w722 -> [w726]
                    tunnel: w720 -> [w724]
                    tunnel: w718 -> [w723]
                    tunnel: [w725] -> w717
                    tunnel: [w723] -> w714
                    tunnel: w717 -> [w729]
                    tunnel: [w729] -> w716
                    tunnel: w714 -> [w727]
                    tunnel: [w727] -> w713
                    tunnel: [w736] -> w721
                    tunnel: w716 -> [w736]
                    tunnel: w715 -> [w732]
                    tunnel: w713 -> [w731]
                    tunnel: [w730] -> w712
                    frame #0 {
                      n429 = Move(source path=w724, error in=w726, 10:w723) -> (error out=w725:errorcluster)  [unwired: 2 in, 2 out]
                    }
                    frame #1 {
                      n430 = Wait (ms)(milliseconds to wait=u32 500) -> ()  [unwired: 1 out]
                    }
                    frame #2 {
                      n431 = call <vilib>:"Check if File or Folder Exists.vi"("path"=w731) -> ("file or folder exists?"=w735:bool)  [unwired: 8 in, 2 out]
                      n432 = Greater?(x=w732, y=9) -> (0:w734:bool)
                      n433 = Or(x=w734, y=w735) -> (x .or. y?=w730:bool)
                    }
                  }
                }
                n434 = Unbundle By Name(w703) -> ("(Final) Data file is saved"=w709)
                n435 = Send Notification(notification=TRUE, notifier=w709, error in (no error)=w708) -> (error out=w707:errorcluster)  [unwired: 1 out]
              }
            }
          }
        }
        n436 = node-c288() -> ()  [unwired: 1 in, 1 out]
      }
      "error out" <- w637
      n437 = node-c288(w638) -> ()  [unwired: 1 out]
    }
    frame Enabled {
    }
  }
  n438 = while {
    stop <- w937 stop-if-true
    # "Only deals with application closing and stopping"
    n439 = event shown="[1] Panel Close?" {
      selector: _ -> [_ _]
      dyn-events: _ -> [_ _]
      timeout: 500 -> [_ _]
      tunnel: [FALSE TRUE] -> w937
      event Timeout {
        n440 = event-data() -> ()  [unwired: 1 in, 3 out]
      }
      event Panel Close? {
        w943 = T18 128 items=["Flush Receive Buffer"=16, "Write Transmit Buffer to Device"=32, "Flush Receive Buffer (No I/O)"=64, "Flush Transmit Buffer"=128] ("Mask")
        w941 = FALSE ("Serial port opened")
        n441 = event-data() -> ()  [unwired: 1 in, 4 out]
        n442 = property on="Serial OUT name" class="VISAName"() -> (error out=w944:errorcluster, "Value"=w942:refnum<visa-resource-name>)  [unwired: 2 in, 1 out]
        n443 = VISA Flush I/O Buffer(VISA resource name=w942, mask (16)=w943, error in (no error)=w944) -> (VISA resource name out=w945:refnum<visa-resource-name>, error out=w946:errorcluster)
        n444 = VISA Clear(VISA resource name=w945, error in (no error)=w946) -> (VISA resource name out=w948:refnum<visa-resource-name>, error out=w947:errorcluster)
        n445 = VISA Close(VISA resource name=w948, error in (no error)=w947) -> (error out=w950:errorcluster)
        n446 = call <vilib>:"Clear Errors.vi"("error in (no error)"=w950) -> ("error out"=w951:errorcluster)  [unwired: 5 in, 1 out]
        n447 = property on="Serial port opened" class="Bool (strict)"(error in=w951, "Value"=w941) -> (error out=w949:errorcluster)  [unwired: 1 in, 1 out]
        n448 = property on="Streaming" class="Bool (strict)"(error in=w949, "Value"=w941) -> (error out=w955:errorcluster)  [unwired: 1 in, 1 out]
        n449 = Current VI's Path() -> (path=w952:path)
        n450 = Open VI Reference(vi path=w952, error in (no error)=w955) -> (vi reference=w953:refnum<vi>, error out=w954:errorcluster)  [unwired: 4 in]
        n451 = invoke class="VI" method="FP.Close"(reference=w953, error in=w954) -> ()  [unwired: 1 in, 3 out]
        n452 = event-data() -> ()  [unwired: 2 in, 1 out]
      }
    }
  }
  n453 = flat-sequence "Things to run at the very beginning of the program" {
    tunnel: [w966] -> w67
    tunnel: [w1086] -> w36
    tunnel: [w994] -> w18
    frame #0 {
      w956 = ""
      w957 = T11 [{"Numeric Control"=12369084, "Numeric Control"=12369084}, {"Numeric Control"=16757760, "Numeric Control"=16757760}, {"Numeric Control"=1976113, "Numeric Control"=8355711}, {"Numeric Control"=3355443, "Numeric Control"=6710886}]  # Button port OFF colors
      w1040 = T11 [{"Numeric Control"=9868950, "Numeric Control"=15790320}, {"Numeric Control"=8388608, "Numeric Control"=8388608}, {"Numeric Control"=4934475, "Numeric Control"=7895160}, {"Numeric Control"=994319, "Numeric Control"=1657881}]  # TTL IO In colors
      w1041 = T11 [{"Numeric Control"=9868950, "Numeric Control"=15790320}, {"Numeric Control"=1988894, "Numeric Control"=3381555}, {"Numeric Control"=4934475, "Numeric Control"=7895160}, {"Numeric Control"=994319, "Numeric Control"=1657881}]  # TTL IO Out colors
      w1064 = T12."Enabled" ("Disabled")
      w1095 = FALSE ("Recording has been started with TTL")
      w971 = "Researcher"
      w1123 = enum32{"Settings", "Recording", "Analysis"}."Settings" ("Main tab control")
      w1130 = enum32{"Settings", "Recording", "Analysis"}."Analysis" ("Main tab control")
      w1138 = enum32{"Settings", "Recording", "Analysis"}."Recording" ("Main tab control")
      n454 = property on="Open serial port" class="Bool (strict)"("Value"=FALSE ("Open serial port")) -> ()  [unwired: 2 in, 2 out]
      n455 = property on="Expand/hide stream panel (Rec)" class="Bool (strict)"("Value"=FALSE ("Expand/hide stream panel (Rec)")) -> ()  [unwired: 2 in, 2 out]
      n456 = property on="Streaming" class="Bool (strict)"("DisabledEnum"=T12."Disabled and Grayed Out" ("Disabled")) -> ()  [unwired: 2 in, 2 out]
      n457 = property on="IO paramaters loaded from file" class="Bool (strict)"("Value"=FALSE ("IO paramaters loaded from file")) -> ()  [unwired: 2 in, 2 out]
      n458 = call-poly <vilib>:"Create Timing Source.vi"("error in (no error)"="error in (no error)", "name (in)"="1 kHz") -> ("error out"=w993:errorcluster, "name (out)"=w994:string)  [unwired: 8 in]
      n459 = property on="Jump to Analysis" class="Bool (strict)"(error in=w993, "Value"=FALSE ("Jump to Analysis")) -> (error out=w1034:errorcluster)  [unwired: 1 in, 1 out]
      n460 = property on="IO parameters string" class="Str"(error in=w1034, "Value"="[12,1,1,0,0,0]" ("IO parameters string")) -> (error out=w1062:errorcluster)  [unwired: 1 in, 1 out]
      n461 = property on="Pane" class="Pane"(error in=w1062) -> (error out=w1072:errorcluster, "Decos[]"=w1073:refnum<vi>[])  [unwired: 1 in, 1 out]
      n462 = for {
        tunnel: w1073 -> [w1160] mode=indexing
        tunnel: w1072 -> [w1158]
        tunnel: [w1157] -> w1066
        n463 = property class="Decor"(reference=w1160, error in=w1158, "Visible"=FALSE) -> (error out=w1157:errorcluster)  [unwired: 1 out]
      }
      n464 = property on="Bridge offset" class="DigNum (strict)"(error in=w1066, "DisabledEnum"=w1064) -> (error out=w1065:errorcluster)  [unwired: 1 in, 1 out]
      n465 = property on="Back to Settings" class="Bool (strict)"(error in=w1065, "DisabledEnum"=w1064, "Visible"=FALSE) -> (error out=w1075:errorcluster)  [unwired: 1 in, 1 out]
      n466 = call "FL_Gen_Bins_for_RunTimes.vi"("Min time, s"=0.5 ("Min run, m"), "N bins"=u16 11, "Max time, s"=10.0 ("Max run, m")) -> ("Bins array"=w1001:dbl[])  [unwired: 1 in]
      n467 = Array Size(array=w1001) -> (size(s)=w1003:i32)
      n468 = Initialize Array(u32 0 ("element"), w1003) -> (w1005:u32[])
      n469 = global write "SW_Globals.vi" "Run Times distribution array"(w1005) -> ()
      n470 = call "FL_Gen_Bins_for_RunLengths.vi"("Min run, m"=0.2, "N bins"=u16 11, "Max run, m"=2.0) -> ("Bins array"=w1009:dbl[])  [unwired: 1 in]
      n471 = Array Size(array=w1009) -> (size(s)=w1011:i32)
      n472 = Initialize Array(u32 0 ("element"), w1011) -> (w1008:u32[])
      n473 = global write "SW_Globals.vi" "Run Lengts distribution array"(w1008) -> ()
      n474 = global write "SW_Globals.vi" "Run Times bins array"(w1001) -> ()
      n475 = property on="Expand/hide stream panel (Rec)" class="Bool (strict)"("Colors [4]"=w957) -> ()  [unwired: 2 in, 2 out]
      n476 = global write "SW_Globals.vi" "Run Lengths bins array"(w1009) -> ()
      n477 = property class="App"() -> ("App.Kind"=w1109:T34)  [unwired: 2 in, 2 out]
      n478 = property on="Ready" class="Bool (strict)"(error in=w1075, "Value"=FALSE ("Ready")) -> (error out=w1033:errorcluster)  [unwired: 1 in, 1 out]
      n479 = global write "SW_Globals.vi" "Run time, s"(0.0 ("Run time, s")) -> ()
      n480 = case shown="\"invalid app kind\", Default" w1109 {
        tunnel: [w1187 w1188 w1189] -> w1102
        frame "invalid app kind", Default {
          n481 = call <vilib>:"Application Directory.vi"() -> ("Application Directory"=w1187:path)
          "Application Directory" <- w1187
        }
        frame "Run Time System" {
          n482 = call <vilib>:"Application Directory.vi"() -> ("Application Directory"=w1188:path)
        }
        frame "Development System" {
          n483 = Current VI's Path() -> (path=w1190:path)
          n484 = Strip Path(path=w1190) -> (stripped path=w1189:path)  [unwired: 1 out]
        }
      }
      n485 = property on="TTL 1 counter" class="DigNum (strict)"("Value"=0 ("TTL 1 counter")) -> ()  [unwired: 2 in, 2 out]
      n486 = property on="TTL 2 counter" class="DigNum (strict)"("Value"=0 ("TTL 1 counter")) -> ()  [unwired: 2 in, 2 out]
      n487 = property on="TTL 3 counter" class="DigNum (strict)"("Value"=0 ("TTL 1 counter")) -> ()  [unwired: 2 in, 2 out]
      n488 = property on="TTL 4 counter" class="DigNum (strict)"("Value"=0 ("TTL 1 counter")) -> ()  [unwired: 2 in, 2 out]
      n489 = global write "SW_Globals.vi" "Recording start timestamp"(timestamp(0 s since 1904-01-01) ("Recording start timestamp")) -> ()
      n490 = call "SW_Generate_Color_Ramp.vi"() -> ("Colors array"=w1115:u32[])  [unwired: 2 in]
      n491 = property on="Zone-based stimulus setup" class="RadioBtnsControl (strict)"(error in=w1033, "Value"=T31."No Selection" ("Stimulus")) -> (error out=w1094:errorcluster)  [unwired: 1 in, 1 out]
      n492 = property on="Pane" class="Pane"("Origin"=T33 {"Horizontal"=0, "Vertical"=0}) -> ()  [unwired: 2 in, 2 out]
      n493 = global write "SW_Globals.vi" "Color ramp array"(w1115) -> ()
      n494 = Build Path(base path=w1102, name or relative path=path "Tracker_settings.tcf") -> (appended path=w1097:path)
      "Path to the settings file" <- w1097
      n495 = call "FL_Gen_Bins_for_Speed.vi"("Speed min"=8.0, "N bins"=u16 10, "Speed max"=300.0) -> ("Bins array"=w1027:dbl[])  [unwired: 1 in]
      n496 = global read "SW_Globals.vi" "Cluster of paths"() -> (w1098:T22)
      n497 = call <vilib>:"Open Config Data.vi"("error in (no error)"=w1094, "create file if necessary (T)"=FALSE, "configuration file path"=w1097) -> ("error out"=w1148:errorcluster, "refnum"=w1147:T5)  [unwired: 6 in, 1 out]
      n498 = Array Size(array=w1027) -> (size(s)=w1026:i32)
      n499 = Initialize Array(u32 0 ("element"), w1026) -> (w1025:u32[])
      n500 = global write "SW_Globals.vi" "Speed bins array"(w1027) -> ()
      n501 = Bundle By Name(cluster=w1098, "Path to the settings file"=w1097) -> (w1096:T22)
      n502 = call <vilib>:"Get Key Names.vi"("section"="Users", "error in (no error)"=w1148, "refnum"=w1147) -> ("error out"=w1144:errorcluster, "key names"=w1140:string[], "refnum out"=w1145:T5)  [unwired: 5 in, 1 out]
      n503 = property on="Type of histogram" class="DigNum (strict)"("Value"=u8 0 ("Type of histogram")) -> (error out=w1007:errorcluster)  [unwired: 2 in, 1 out]
      n504 = property on="Histograms (normalized)" class="WFGraph (strict)"(error in=w1007, "XScale.Ofst&Mult"=T30 {"Offset"=1.0, "Multiplier"=0.0} ("X Scale.Offset and Multiplier"), "XScale.ScaleFit"=u8 0 ("X Scale.Scale Fit"), "YScale.Mapping Mode"=u8 0 ("Y Scale.Mapping Mode"), "Plot.Fill/Pt. Color"=u32 15790320 ("Plot.Fill/Point Color"), "XScale.Range"=T21 {"Minimum"=0.0, "Maximum"=14.0, "Increment"=1.0, "Minor Increment"=1.0, "Start"=0.0} ("X Scale.Range")) -> ()  [unwired: 1 in, 2 out]
      n505 = global write "SW_Globals.vi" "Speed distribution array"(w1025) -> ()
      n506 = call <vilib>:"Read Key (U32).vi"("section"="Defaults", "error in (no error)"=w1144, "key"="Default User", "refnum"=w1145) -> ("error out"=w970:errorcluster, "value"=w1141:u32, "refnum out"=w1119:T5)  [unwired: 4 in, 1 out]
      n507 = global write "SW_Globals.vi" "Cluster of paths"(w1096) -> ()
      n508 = Index Array(array=w1140, index=w1141) -> ()  [unwired: 1 out]
      n509 = call "SW_Load_settings_to_main_tab.vi"("Refnum in"=w1119, "User Name"=w971, "error in (no error)"=w970) -> ("VISA resource name"=w966:string, "Refnum out"=→"Settings file refnum out":T5, "IO parameters cluster"=w969:T2, "Settings cluster out"=w967:T35, "Stimulus presets array"=w968:T36, "error out"=w1054:errorcluster)  [unwired: 2 in]
      "Port" <- w966
      n510 = Unbundle By Name(w967) -> ("Name prefix"=w986:string, "Twisted neck"=w985:bool, "Offset H."=w982:sgl, "Stop at"=w984:dbl, "\"Stop at\" enabled"=w983:bool, "N segments MIDFIELD"=w980:u8, "N segments BORDER"=w979:u8, "Radius, mm CENTER"=w978:u16, "Radius, mm MIDFIELD"=w977:u16, "Starting angle MIDFIELD"=w976:i16, "Starting angle BORDER"=w975:i16, "Cage diameter, mm"=w973:u16, "Bridge swap"=w974:bool, "Bridge V. offset"=w981:sgl, "Data filtering"=w962:u16)
      n511 = case "Let's set flag for alternative magnets orintation" shown="240" w973 {
        frame 180, Default {
          n512 = global write "SW_Globals.vi" "Alternative magnets orientation"(FALSE ("Alternative magnets orientation")) -> ()
        }
        frame 240 {
          n513 = global write "SW_Globals.vi" "Alternative magnets orientation"(FALSE ("Alternative magnets orientation")) -> ()
        }
        frame 290 {
          n514 = global write "SW_Globals.vi" "Alternative magnets orientation"(FALSE ("Alternative magnets orientation")) -> ()
        }
        frame 325 {
          n515 = global write "SW_Globals.vi" "Alternative magnets orientation"(FALSE ("Alternative magnets orientation")) -> ()
        }
        frame 327 {
          n516 = global write "SW_Globals.vi" "Alternative magnets orientation"(TRUE ("Alternative magnets orientation")) -> ()
        }
        frame 333 {
          n517 = global write "SW_Globals.vi" "Alternative magnets orientation"(FALSE ("Alternative magnets orientation")) -> ()
        }
      }
      n518 = local write "Name Prefix"(w986) -> ()
      n519 = local write "Twisted neck"(w985) -> ()
      n520 = local write "Bridge horizontal offset"(w982) -> ()
      n521 = local write "Stop record at"(w984) -> ()
      n522 = local write "\"Stop at\" enabled"(w983) -> ()
      n523 = local write "N segments MIDFIELD"(w980) -> ()
      n524 = local write "N segments BORDER"(w979) -> ()
      n525 = local write "Radius, mm CENTER"(w978) -> ()
      n526 = local write "Radius, mm MIDFIELD"(w977) -> ()
      n527 = local write "Bridge offset"(w981) -> ()
      n528 = local write "Starting angle MIDFIELD"(w976) -> ()
      n529 = local write "Starting angle BORDER"(w975) -> ()
      n530 = local write "Cage diameter, mm"(w973) -> ()
      n531 = local write "Data filtering"(w962) -> ()
      n532 = Unbundle By Name(w969) -> ("SYNC configuration"=w1057:u16, "IO 1 configuration"=w998:u16, "IO 2 configuration"=w997:u16)
      n533 = call "SW_get_config_of_Zones_and_IO.vi"("Sync parameters cluster input"=w969) -> ("Zones out config bin"=w1050:bool[], "Ports IO config (OUT is FALSE)"=w1032:bool[], "IO inversion config."=w992:u16)  [unwired: 1 out]
      n534 = global write "SW_Globals.vi" "IO inversion config."(w992) -> ()
      n535 = property on="Bridge swap" class="Bool (strict)"(error in=w1054, "DisabledEnum"=T12."Enabled" ("Disabled"), "Value"=w974) -> (error out=w1100:errorcluster)  [unwired: 1 in, 1 out]
      n536 = call "SW_get_config_for_Start_Stop_pulses.vi"("Sync parameters cluster input"=w969) -> ("Start/Stop out pulses config"=→"Start/Stop out pulses config":u32, "Start/Stop in config"=→"Start/Stop in config":u32, "Start/Stop in config bin"=w1052:bool[], "Start/Stop out pulses config bin"=w1051:bool[])
      n537 = call "SW_Gen_Available_TTL_outputs_array.vi"("IO 2 configuration"=w997, "IO 1 configuration"=w998, "SYNC configuration"=w1057) -> ("Available TTL outputs array"=w1056:cluster{"String":string, "Value":i32}[])
      n538 = global write "SW_Globals.vi" "IO parameters cluster"(w969) -> ()
      n539 = global write "SW_Globals.vi" "Start/Stop out pulses config bin"(w1051) -> ()
      n540 = property on="TTL out" class="Ring (strict)"("StringsAndValues[]"=w1056) -> ()  [unwired: 2 in, 2 out]
      n541 = global write "SW_Globals.vi" "Zones out config bin"(w1050) -> ()
      n542 = global write "SW_Globals.vi" "Start/Stop in config bin"(w1052) -> ()
      n543 = global write "SW_Globals.vi" "IO ports config"(w1032) -> ()
      n544 = call "SW_get_IO_ports_representation.vi"("Sync parameters cluster input"=w969) -> ("IO status indicator"=→"IO status indicator":T37)
      n545 = property on="Main tab control" class="TabCtl (strict)"(error in=w1100, "Value"=w1138) -> (error out=w1135:errorcluster, "Pages"=w1139:refnum<vi>[])  [unwired: 1 in, 1 out]
      n546 = Index Array(array=w1032, index=0) -> (element=w1045:bool)
      n547 = Index Array(array=w1032, index=1) -> (element=w1044:bool)
      n548 = Index Array(array=w1032, index=2) -> (element=w1043:bool)
      n549 = Index Array(array=w1032, index=3) -> (element=w1042:bool)
      n550 = To Long Integer(number=w1138) -> (32bit integer=w1137:i32)
      n551 = Select(t=w1040, s=w1045, f=w1041) -> (s? t:f=w1039:T11)
      n552 = Select(t=w1040, s=w1044, f=w1041) -> (s? t:f=w1038:T11)
      n553 = Select(t=w1040, s=w1042, f=w1041) -> (s? t:f=w1036:T11)
      n554 = Index Array(array=w1139, index=w1137) -> (element=w1136:refnum<vi>)
      n555 = Select(t=w1040, s=w1043, f=w1041) -> (s? t:f=w1037:T11)
      n556 = property class="Page"(reference=w1136, error in=w1135, "PageEnb"=T32."Page Disabled & Grayed" ("Page Enabled State")) -> (error out=w1133:errorcluster)  [unwired: 1 out]
      n557 = property on="TTL IO 1 (recording)" class="Bool (strict)"("Colors [4]"=w1039) -> ()  [unwired: 2 in, 2 out]
      n558 = property on="TTL IO 3 (recording)" class="Bool (strict)"("Colors [4]"=w1037) -> ()  [unwired: 2 in, 2 out]
      n559 = property on="TTL IO 2 (recording)" class="Bool (strict)"("Colors [4]"=w1038) -> ()  [unwired: 2 in, 2 out]
      n560 = property on="TTL IO 1 (analysis)" class="Bool"("Colors [4]"=w1039) -> ()  [unwired: 2 in, 2 out]
      n561 = property on="TTL IO 4 (recording)" class="Bool (strict)"("Colors [4]"=w1036) -> ()  [unwired: 2 in, 2 out]
      n562 = property on="Main tab control" class="TabCtl (strict)"(error in=w1133, "Value"=w1130) -> (error out=w1132:errorcluster, "Pages"=w1131:refnum<vi>[])  [unwired: 1 in, 1 out]
      n563 = To Long Integer(number=w1130) -> (32bit integer=w1129:i32)
      n564 = property on="TTL IO 3 (analysis)" class="Bool"("Colors [4]"=w1037) -> ()  [unwired: 2 in, 2 out]
      n565 = property on="TTL IO 2 (analysis)" class="Bool"("Colors [4]"=w1038) -> ()  [unwired: 2 in, 2 out]
      n566 = Index Array(array=w1131, index=w1129) -> (element=w1128:refnum<vi>)
      n567 = property on="TTL IO 4 (analysis)" class="Bool"("Colors [4]"=w1036) -> ()  [unwired: 2 in, 2 out]
      n568 = global write "SW_Globals.vi" "TTL recording start signal has been successfully reset"(w1095) -> ()
      n569 = property class="Page"(reference=w1128, error in=w1132, "PageEnb"=T32."Page Disabled & Grayed" ("Page Enabled State")) -> (error out=w1120:errorcluster)  [unwired: 1 out]
      n570 = global write "SW_Globals.vi" "Recording has been stopped with TTL"(w1095) -> ()
      n571 = global write "SW_Globals.vi" "Recording has been started with TTL"(w1095) -> ()
      n572 = property on="Main tab control" class="TabCtl (strict)"(error in=w1120, "Value"=w1123) -> (error out=w1121:errorcluster, "Pages"=w1122:refnum<vi>[])  [unwired: 1 in, 1 out]
      n573 = To Long Integer(number=w1123) -> (32bit integer=w1124:i32)
      n574 = for {
        tunnel: w968 -> [w1165] mode=indexing
        tunnel: [w1164] -> w1076 mode=indexing if=w1163
        i -> [w1162]
        n575 = Greater Than 0?(x=w1162) -> (x > 0?=w1161:bool)
        n576 = Unbundle By Name(w1165) -> ("Stim. has been set"=w1163:bool)
        n577 = case shown="True" w1161 {
          tunnel: w1163 -> [_ w1176]
          tunnel: w1162 -> [_ w1172]
          frame False {
          }
          frame True {
            w1170 = refnum<vi> refnum  # Boolean
            n578 = property on="Colors for Stim. setup" class="Arr (strict)"() -> ("Value"=w1175:T3)  [unwired: 2 in, 2 out]
            n579 = Decrement(x=w1172) -> (x-1=w1166:i32)
            n580 = property on="Zone-based stimulus setup" class="RadioBtnsControl (strict)"() -> ("Controls[]"=w1173:refnum<vi>[])  [unwired: 2 in, 2 out]
            n581 = Select(t=w1175, s=w1176, f=T11 [{"Numeric Control"=12369084, "Numeric Control"=12369084}, {"Numeric Control"=6603023, "Numeric Control"=6603023}, {"Numeric Control"=1976113, "Numeric Control"=1976113}, {"Numeric Control"=2575993, "Numeric Control"=2575993}] ("Colors [4] 2")) -> (s? t:f=w1168:T11)
            n582 = Index Array(array=w1173, index=w1166) -> (element=w1171:refnum<vi>)
            n583 = To More Specific Class(target class=w1170, reference=w1171) -> (specific class reference=w1169:refnum<vi>)  [unwired: 1 in, 1 out]
            n584 = property class="Bool"(reference=w1169, "Colors [4]"=w1168, "Value"=FALSE) -> ()  [unwired: 1 in, 2 out]
          }
        }
        n585 = To Unsigned Byte Integer(number=w1162) -> (unsigned 8bit integer=w1164:u8)
      }
      n586 = global write "SW_Globals.vi" "Key_pressed"(w956) -> ()
      n587 = global write "SW_Globals.vi" "Regions to track"(u8[] [] ("Regions to track")) -> ()
      n588 = Index Array(array=w1122, index=w1124) -> (element=w1125:refnum<vi>)
      n589 = property class="Page"(reference=w1125, error in=w1121, "PageEnb"=T32."Page Enabled" ("Page Enabled State")) -> (error out=w1118:errorcluster)  [unwired: 1 out]
      n590 = property on="Record/Stop" class="Bool (strict)"(error in=w1118, "Value"=FALSE ("Record/Stop")) -> (error out=w1117:errorcluster)  [unwired: 1 in, 1 out]
      n591 = Flatten To String(anything="Zones presence indicator") -> (data string=w1106:string)  [unwired: 3 in, 2 out]
      n592 = String Length(string=w1106) -> (length=w1105:i32)
      n593 = global write "SW_Globals.vi" "Regions to track"(w1076) -> ()
      n594 = property on="Play/Pause" class="Bool (strict)"(error in=w1117, "Value"=FALSE ("Play/Pause")) -> (error out=w1101:errorcluster)  [unwired: 1 in, 1 out]
      n595 = global write "SW_Globals.vi" "Zone-based stimulus presets"(w968) -> ()
      n596 = property on="Stimulus presets" class="Arr (strict)"("Value"=w968) -> (error out=w1082:errorcluster)  [unwired: 2 in, 1 out]
      n597 = Initialize Array(FALSE, w1105) -> (w1015:bool[])
      "Zones presence array" <- w1015
      n598 = Initialize Array(0, w1105) -> (→"Zones allocation array":i32[])
      n599 = global write "SW_Globals.vi" "Speed detection threshold, mm/s"(1000.0 ("Speed detection threshold, mm/s")) -> ()
      n600 = property on="Stimulus presets" class="Arr (strict)"(error in=w1082, "Index Values"=u32[] [0], "DisabledEnum"=T12."Disabled and Grayed Out" ("Disabled")) -> (error out=w1061:errorcluster)  [unwired: 1 in, 1 out]
      n601 = property on="Record timestamp" class="DigNum (strict)"(error in=w1101, "DisabledEnum"=T12."Disabled and Grayed Out" ("Disabled"), "Value"=0.0 ("Record timestamp")) -> (error out=w1086:errorcluster)  [unwired: 1 in, 1 out]
      n602 = global write "SW_Globals.vi" "Zones presence array"(w1015) -> ()
      n603 = global write "SW_Globals.vi" "Run time threshold, s"(4.0 ("Run time threshold, s")) -> ()
      n604 = global write "SW_Globals.vi" "Run time pause, s"(5.0 ("Run time pause, s")) -> ()
      n605 = global write "SW_Globals.vi" "Run time stim, s"(1.0 ("Run time stim, s")) -> ()
      n606 = property on="Data filtering" class="Ring (strict)"(error in=w1061, "DisabledEnum"=T12."Enabled" ("Disabled")) -> (error out=w1060:errorcluster)  [unwired: 1 in, 1 out]
      n607 = property on="N segments BORDER" class="DigNum (strict)"(error in=w1060) -> (error out=w1087:errorcluster, "Value"=w1091:u8)  [unwired: 1 in, 1 out]
      n608 = property on="N segments MIDFIELD" class="DigNum (strict)"(error in=w1087) -> (error out=w1079:errorcluster, "Value"=w1090:u8)  [unwired: 1 in, 1 out]
      n609 = property on="Zone-based stimulus setup" class="RadioBtnsControl (strict)"(error in=w1079) -> (error out=w1085:errorcluster, "Controls[]"=w1089:refnum<vi>[])  [unwired: 1 in, 1 out]
      n610 = Compound Arithmetic op=ADD(w1091, w1090, u8 1 ("value")) -> (w1088:u8)
      n611 = for {
        tunnel: w1089 -> [w1186] mode=indexing
        tunnel: w1088 -> [w1182]
        tunnel: w1085 -> [w1177]
        tunnel: [w1179] -> w1084
        i -> [w1178]
        n612 = Increment(x=w1178) -> (x+1=w1181:i32)
        n613 = Greater Or Equal?(x=w1182, y=w1181) -> (x >= y?=w1180:bool)
        n614 = Select(t=T12."Enabled" ("Disabled"), s=w1180, f=T12."Disabled and Grayed Out") -> (s? t:f=w1184:T12)
        n615 = property class="Ctl"(reference=w1186, error in=w1177, "DisabledEnum"=w1184) -> (error out=w1179:errorcluster)  [unwired: 1 out]
      }
      n616 = property on="Zone-based stimulus setup" class="RadioBtnsControl (strict)"(error in=w1084, "Value"=T8."No Selection" ("Stim. setup")) -> (error out=w1071:errorcluster)  [unwired: 1 in, 1 out]
      n617 = property on="Pane" class="Pane"(error in=w1071) -> ("Decos[]"=w1070:refnum<vi>[])  [unwired: 1 in, 2 out]
      n618 = Index Array(array=w1070, index=2) -> (element=w1068:refnum<vi>)
      n619 = property class="Decor"(reference=w1068, "Visible"=TRUE) -> ()  [unwired: 1 in, 2 out]
      "Current User" <- w971
      "Start TTL is fired" <- FALSE ("Start/Stop TTL is fired")
      "Stop TTL is fired" <- FALSE ("Start/Stop TTL is fired")
      "Serial port opened" <- FALSE ("Serial port opened")
      "Key_pressed" <- w956
    }
  }
  n620 = node-c288(w18, i64 2 ("Period"), 100 ("Priority"), 1000 ("Timeout")) -> (w15:T13)  [unwired: 1 in]
  n621 = call "SW_SG_coefficients_3-51.vi"("Select filter length"=w23, "Point of interest (can be used for extrapolation)"=0) -> ("SG coefficients"=w22:T38)  [unwired: 1 in]
  n622 = call "SW_SG_coefficients_3-51.vi"("Select filter length"=w27, "Point of interest (can be used for extrapolation)"=0) -> ("SG coefficients"=w25:T38)  [unwired: 1 in]
  n623 = call "SW_SG_coefficients_3-51.vi"("Select filter length"=w31, "Point of interest (can be used for extrapolation)"=0) -> ("SG coefficients"=w28:T38)  [unwired: 1 in]
  n624 = call "SW_SG_coefficients_3-51.vi"("Select filter length"=w21, "Point of interest (can be used for extrapolation)"=0) -> ("SG coefficients"=w19:T38)  [unwired: 1 in]
  n625 = Bundle By Name(cluster=T10 {"SG coefficients 3/5"={"0th order SG coefficients"=[], "1st order SG coefficients"=[]}, "SG coefficients 3/11"={"0th order SG coefficients"=[], "1st order SG coefficients"=[]}, "SG coefficients 3/31"={"0th order SG coefficients"=[], "1st order SG coefficients"=[]}, "SG coefficients 3/51"={"0th order SG coefficients"=[], "1st order SG coefficients"=[]}} ("Input cluster of SG coefficients"), "SG coefficients 3/5"=w28, "SG coefficients 3/11"=w25, "SG coefficients 3/31"=w22, "SG coefficients 3/51"=w19) -> (w29:T10)
  n626 = node-c288(w18, w48, 900 ("Priority")) -> (w50:T13)
  n627 = timed-loop "This loop is all about temporary data processing and streaming to the interface part" {
    tunnel: w17 -> [w1210]
    tunnel: w1 -> [w1209]
    tunnel: [w1198] -> w65
    timing: w50 -> [_]
    timing-out: [_] -> w49
    tunnel: w48 -> [w1197]
    tunnel: w29 -> [w1192]
    tunnel: [w1191] -> w16
    i -> [w1208]
    stop <- w1196 stop-if-true
    n628 = node-c288() -> ()  [unwired: 1 in, 1 out]
    n629 = Unbundle By Name(w1210) -> ("Complete stop"=w1211:refnum<notifier>, "Play/Pause status"=w1205:refnum<notifier>)
    n630 = flat-sequence {
      tunnel: w1210 -> [w1216]
      tunnel: w1197 -> [w1226]
      tunnel: w1208 -> [w1225]
      tunnel: w1206 -> [w1224]
      tunnel: w1195 -> [w1223]
      tunnel: [w1222] -> w1204
      tunnel: w1202 -> [w1221]
      tunnel: w1201 -> [w1220]
      tunnel: w1199 -> [w1219]
      tunnel: [w1218] -> w1198
      tunnel: w1193 -> [w1217]
      tunnel: [w1216] -> w1194
      tunnel: w1192 -> [w1215]
      tunnel: [w1214] -> w1191
      tunnel: w1205 -> [w1349]
      tunnel: w1204 -> [w1340]
      tunnel: [w1348] -> w1203
      tunnel: w1194 -> [w1338]
      tunnel: w1193 -> [w1347]
      frame #0 {
        n631 = case shown="\"Play\"" w1221 {
          tunnel: w1216 -> [_ w1317]
          tunnel: w1226 -> [_ w1316]
          tunnel: w1225 -> [_ w1315]
          tunnel: w1224 -> [_ w1314]
          tunnel: w1223 -> [_ w1311]
          tunnel: [w1227 w1298] -> w1222
          tunnel: w1220 -> [w1227 w1307]
          tunnel: w1219 -> [_ w1310]
          tunnel: [_ w1305] -> w1218
          tunnel: w1217 -> [_ w1244]
          tunnel: w1215 -> [_ w1236]
          tunnel: [_ w1233] -> w1214
          frame "Pause", Default {
          }
          frame "Play" {
            w1252 = "." ("string")
            n632 = property on="Bridge horizontal offset" class="DigNum (strict)"() -> ("Value"=w1237:sgl)  [unwired: 2 in, 2 out]
            n633 = property on="Bridge offset" class="DigNum (strict)"() -> ("Value"=w1238:sgl)  [unwired: 2 in, 2 out]
            n634 = property on="Twisted neck" class="Bool (strict)"() -> ("Value"=w1239:bool)  [unwired: 2 in, 2 out]
            n635 = global read "SW_Globals.vi" "Alternative magnets orientation"() -> (w1242:bool)
            n636 = property on="Bridge swap" class="Bool (strict)"(error in=w1307) -> (error out=w1306:errorcluster, "Value"=w1243:bool)  [unwired: 1 in, 1 out]
            n637 = local read "Pixels per mm"() -> (w1308:dbl)
            n638 = Bundle By Name(cluster=T40 {"Offset V."=0.0, "Offset H."=0.0, "Bridge swap"=FALSE, "Turn magnets 90 deg."=FALSE, "Twisted neck"=FALSE} ("Offsets, swaps and rotations"), "Offset V."=w1238, "Offset H."=w1237, "Bridge swap"=w1243, "Turn magnets 90 deg."=w1242, "Twisted neck"=w1239) -> (w1240:T40)
            n639 = property on="Diagram at recording" class="Pict"() -> ("Bounds"=w1309:T19)  [unwired: 2 in, 2 out]
            n640 = call "FL_Preprocess_and_save_incrementally_TDMS.vi"("Temporary file output path"=w1311, "Loop iteration"=w1315, "Offsets, swaps and rotations"=w1240, "Loop speed in ms"=w1316, "Save every N seconds"=u32 8, "error in (no error)"=w1306, "Filter type"="Data filtering", "Sensor read input"=w1314, "Input cluster of SG coefficients"=w1236, "tdms file in"=w1244, "Pixels per mm"=w1308, "Data flow controls in"=w1317, "Diagram at recording bounds"=w1309, "Sensor board size"=w1310) -> ("Eff. save interval"=→"Eff. save interval":sgl, "Latest sensor output (decoded)"=w1234:string[][], "Fire TTL"=w1245:bool, "TTL out N"=w1246:u8, "Current TTL status"=w1291:u8, "error out"=w1299:errorcluster)
            "Current TTL status" <- w1291
            n641 = for {
              tunnel: w1234 -> [w1319] mode=indexing
              tunnel: [w1318] -> w1233
              n642 = call <extravilib>:"Write.vi"("element"=w1319) -> ("channel"=w1318:T41)  [unwired: 8 in, 2 out]
            }
            n643 = Index Array "TTL inputs"(array=w1234, index (col)=14) -> (element=w1229:string[])  [unwired: 1 in]
            n644 = property on="Start/Stop in config" class="DigNum (strict)"() -> ("Value"=w1295:u32)  [unwired: 2 in, 2 out]
            n645 = Decimal String To Number(string=w1229, default (0L)=u8 0 ("default (0 I32)")) -> (number=w1296:u8[])  [unwired: 1 in, 1 out]
            n646 = call <extravilib>:"Write.vi"("size (1)"=5, "lossy behavior (drop oldest)"=Lossy_Behavior."drop oldest element", "element"=w1234) -> ("channel"=w1305:T42)  [unwired: 6 in, 2 out]
            n647 = Greater Than 0?(x=w1295) -> (x > 0?=w1297:bool)
            n648 = Search 1D Array(1D array=w1296, element=w1295) -> (index of element=w1294:i32)  [unwired: 1 in]
            n649 = Greater Or Equal To 0?(x=w1294) -> (x >= 0?=w1293:bool)
            n650 = And(x=w1297, y=w1293) -> (x .and. y?=w1301:bool)
            n651 = call <vilib>:"High Resolution Relative Seconds.vi"() -> ("relative seconds"=w1232:dbl)
            n652 = feedback-in #2(w1232) -> ()
            n653 = feedback #2(w1232) -> (w1231:dbl)
            n654 = Subtract(x=w1232, y=w1231) -> (x-y=w1230:dbl)
            n655 = call "FL_Get_TTL_in_pulse_length_2.vi"("Time since the last frame, s"=w1230, "Latest sensor input (decoded)"=w1229) -> ("TTL pulse length, ms"=w1228:u32)
            n656 = case shown="True" w1301 {
              tunnel: w1228 -> [_ w1325]
              frame False {
              }
              frame True {
                n657 = global read "SW_Globals.vi" "Recording has been started with TTL"() -> (w1333:bool)
                n658 = feedback #3(FALSE) -> (w1336:bool)
                n659 = Not(x=w1336) -> (.not. x?=w1337:bool)
                n660 = Greater Or Equal?(x=w1325, y=u32 225) -> (x >= y?=w1323:bool)
                n661 = global read "SW_Globals.vi" "Recording has been stopped with TTL"() -> (w1328:bool)
                n662 = And(x=w1337, y=w1323) -> (x .and. y?=w1334:bool)
                n663 = Not(x=w1323) -> (.not. x?=w1332:bool)
                n664 = local write "TTL is long enough"(w1323) -> ()
                n665 = And(x=w1333, y=w1332) -> (x .and. y?=w1331:bool)
                n666 = Or(x=w1334, y=w1333) -> (x .or. y?=w1322:bool)
                n667 = feedback-in #3(w1322) -> ()
                n668 = global read "SW_Globals.vi" "TTL recording start signal has been successfully reset"() -> (w1330:bool)
                n669 = Or(x=w1330, y=w1331) -> (x .or. y?=w1324:bool)
                n670 = local write "Started"(w1322) -> ()
                n671 = Compound Arithmetic op=AND(w1324, w1322, w1323) -> (w1329:bool)
                n672 = global write "SW_Globals.vi" "Recording has been started with TTL"(w1322) -> ()
                n673 = global write "SW_Globals.vi" "TTL recording start signal has been successfully reset"(w1324) -> ()
                n674 = Or(x=w1329, y=w1328) -> (x .or. y?=w1321:bool)
                n675 = local write "Reset starting pulse"(w1324) -> ()
                n676 = local write "Stopped"(w1321) -> ()
                n677 = Not(x=w1321) -> (.not. x?=w1327:bool)
                n678 = global write "SW_Globals.vi" "Recording has been stopped with TTL"(w1321) -> ()
                n679 = Compound Arithmetic op=AND(w1322, w1324, w1327) -> (w1320:bool)
                n680 = local write "Record"(w1320) -> ()
                n681 = property on="Record/Stop" class="Bool (strict)"("Value"=w1320) -> ()  [unwired: 2 in, 2 out]
                n682 = property on="TTL REC" class="Bool (strict)"("Value"=w1320) -> ()  [unwired: 2 in, 2 out]
              }
            }
            n683 = Number To Boolean Array(number=w1291) -> (Boolean array=w1287:bool[])
            n684 = Index Array(array=w1287, index=0) -> (element=w1279:bool)
            "TTL IO 1 (recording)" <- w1279
            n685 = Index Array(array=w1287, index=1) -> (element=w1259:bool)
            "TTL IO 2 (recording)" <- w1259
            n686 = Index Array(array=w1287, index=2) -> (element=w1258:bool)
            "TTL IO 3 (recording)" <- w1258
            n687 = Index Array(array=w1287, index=3) -> (element=w1260:bool)
            "TTL IO 4 (recording)" <- w1260
            n688 = feedback #4(TRUE) -> (w1262:bool)
            n689 = feedback-in #4(w1260) -> ()
            n690 = feedback #5(TRUE) -> (w1272:bool)
            n691 = feedback-in #5(w1258) -> ()
            n692 = feedback #6(TRUE) -> (w1284:bool)
            n693 = feedback-in #6(w1279) -> ()
            n694 = feedback #7(TRUE) -> (w1273:bool)
            n695 = feedback-in #7(w1259) -> ()
            n696 = Not(x=w1262) -> (.not. x?=w1263:bool)
            n697 = Not(x=w1272) -> (.not. x?=w1270:bool)
            n698 = Not(x=w1284) -> (.not. x?=w1283:bool)
            n699 = Not(x=w1273) -> (.not. x?=w1275:bool)
            n700 = local read "TTL 4 counter"() -> (w1265:u32)
            n701 = And(x=w1263, y=w1260) -> (x .and. y?=w1264:bool)
            n702 = local read "TTL 3 counter"() -> (w1268:u32)
            n703 = local read "TTL 1 counter"() -> (w1281:u32)
            n704 = And(x=w1270, y=w1258) -> (x .and. y?=w1269:bool)
            n705 = local read "TTL 2 counter"() -> (w1277:u32)
            n706 = And(x=w1283, y=w1279) -> (x .and. y?=w1282:bool)
            n707 = And(x=w1275, y=w1259) -> (x .and. y?=w1276:bool)
            n708 = Increment(x=w1265) -> (x+1=w1266:u32)
            n709 = Increment(x=w1268) -> (x+1=w1267:u32)
            n710 = Increment(x=w1281) -> (x+1=w1280:u32)
            n711 = Select(t=w1266, s=w1264, f=w1265) -> (s? t:f=w1254:u32)
            "TTL 4 counter" <- w1254
            n712 = Increment(x=w1277) -> (x+1=w1278:u32)
            n713 = Select(t=w1267, s=w1269, f=w1268) -> (s? t:f=w1255:u32)
            "TTL 3 counter" <- w1255
            n714 = Select(t=w1280, s=w1282, f=w1281) -> (s? t:f=w1257:u32)
            "TTL 1 counter" <- w1257
            n715 = Select(t=w1278, s=w1276, f=w1277) -> (s? t:f=w1256:u32)
            "TTL 2 counter" <- w1256
            n716 = Number To Decimal String(number=w1257) -> (decimal integer string=w1253:string)  [unwired: 1 in]
            n717 = Number To Decimal String(number=w1256) -> (decimal integer string=w1251:string)  [unwired: 1 in]
            n718 = Number To Decimal String(number=w1255) -> (decimal integer string=w1250:string)  [unwired: 1 in]
            n719 = Number To Decimal String(number=w1254) -> (decimal integer string=w1249:string)  [unwired: 1 in]
            n720 = global read "SW_Globals.vi" "IO inversion config."() -> (w1247:u16)
            n721 = global read "SW_Globals.vi" "VISA resource name"() -> (w1300:refnum<visa-resource-name>)
            n722 = call "SW_Fire_TTL_during_the_acquisition_universal.vi"("IO inversion config."=w1247, "error in (no error)"=w1299, "Serial Port In"=w1300, "TTL port(s) config to fire"=w1246, "Fire TTL"=w1245) -> ("error out"=w1298:errorcluster)  [unwired: 6 in]
            n723 = Concatenate Strings(w1253, w1252, w1251, w1252, w1250, w1252, w1249) -> (→"IO pulses count":string)
          }
        }
      }
      frame #1 {
        n724 = Unbundle By Name(w1338) -> ("Recording now"=w1346:refnum<notifier>, "Has been recorded"=w1345:refnum<notifier>)
        n725 = Get Notifier Status(notifier=w1345) -> (current notification=w1343:bool)  [unwired: 1 in, 4 out]
        n726 = Get Notifier Status(notifier=w1346) -> (current notification=w1344:bool)  [unwired: 1 in, 4 out]
        n727 = Not(x=w1344) -> (.not. x?=w1342:bool)
        n728 = And(x=w1343, y=w1342) -> (x .and. y?=w1341:bool)
        n729 = case shown="True" w1341 {
          tunnel: w1347 -> [_ w1359]
          tunnel: w1340 -> [w1350 w1358]
          tunnel: [w1350 w1351] -> w1339
          tunnel: w1338 -> [_ w1355]
          frame False {
          }
          frame True {
            n730 = Unbundle By Name(w1355) -> ("(Final) Data file is saved"=w1354:refnum<notifier>)
            n731 = TDMS Close(8:w1358, 11:w1359) -> (0:w1357:errorcluster)  [unwired: 1 out]
            n732 = call <vilib>:"Clear Errors.vi"("error in (no error)"=w1357, "specific error code to clear (0: all)"=-2501) -> ("error out"=w1352:errorcluster)  [unwired: 4 in, 1 out]
            n733 = Send Notification(notification=TRUE, notifier=w1354, error in (no error)=w1352) -> (error out=w1351:errorcluster)  [unwired: 1 out]
          }
        }
        n734 = Get Notifier Status(notifier=w1349, error in (no error)=w1339) -> (current notification=w1348:string)  [unwired: 4 out]
      }
    }
    n735 = Flush Queue(queue=w1209) -> (remaining elements=w1206:T43, error out=w1201:errorcluster)  [unwired: 1 in, 1 out]
    n736 = local read "Board size"() -> (w1199:string)
    n737 = global read "SW_Globals.vi" "Cluster of paths"() -> (w1207:T22)
    n738 = Get Notifier Status(notifier=w1211) -> (current notification=w1196:bool)  [unwired: 1 in, 4 out]
    n739 = Unbundle By Name(w1207) -> ("Temporary file output path"=w1195:path, "TDMS file reference"=w1193:refnum<k34>)
    n740 = feedback-in #8(w1203) -> ()
    n741 = feedback #8("Pause" ("String")) -> (w1202:string)
    n742 = node-c288() -> ()  [unwired: 1 in, 1 out]
  }
  n743 = timed-loop {
    timing: w15 -> [_]
    timing-out: [_] -> w14
    tunnel: w17 -> [w1361]
    tunnel: w16 -> [w1362]
    stop <- w1360 stop-if-true
    n744 = node-c288() -> ()  [unwired: 1 in, 1 out]
    n745 = Unbundle By Name(w1361) -> ("Complete stop"=w1365:refnum<notifier>)
    n746 = Get Notifier Status(notifier=w1365) -> (current notification=w1360:bool)  [unwired: 1 in, 4 out]
    n747 = event shown="[3] Key Up" {
      selector: _ -> [_ _ _ _ _]
      dyn-events: _ -> [_ _ _ _ _]
      timeout: 0 -> [_ _ _ _ _]
      event Timeout {
        n748 = event-data() -> ()  [unwired: 1 in, 3 out]
      }
      event "Expand/hide stream panel (Rec)": Value Change {
        n749 = event-data() -> ("NewVal"=w1401:bool)  [unwired: 1 in, 5 out]
        n750 = case shown="True" w1401 {
          tunnel: [w1406 w1421] -> w1400
          tunnel: 120 ("y") -> [w1402 w1417]
          frame True {
            n751 = Current VI's Path() -> (path=w1412:path)
            n752 = property on="Main tab control" class="TabCtl (strict)"() -> ("PaneHeight"=w1414:u32)  [unwired: 2 in, 2 out]
            n753 = property on="Expand/hide stream panel (Rec)" class="Bool (strict)"() -> ("Top"=w1416:i32)  [unwired: 2 in, 2 out]
            n754 = Open VI Reference(vi path=w1412) -> (vi reference=w1411:refnum<vi>, error out=w1410:errorcluster)  [unwired: 5 in]
            n755 = Add(x=w1416, y=w1402) -> (x+y=w1415:i32)
            n756 = property class="VI"(reference=w1411, error in=w1410) -> (reference out=w1408:refnum<vi>, error out=w1407:errorcluster, "Front Panel.PanelBounds"=w1405:T44)
            n757 = Add(x=w1414, y=w1402) -> (x+y=w1413:u32)
            n758 = property on="Expand/hide stream panel (Rec)" class="Bool (strict)"("Top"=w1415) -> ()  [unwired: 2 in, 2 out]
            n759 = property on="Main tab control" class="TabCtl (strict)"("PaneHeight"=w1413) -> ()  [unwired: 2 in, 2 out]
            n760 = Unbundle By Name(w1405) -> ("Bottom"=w1409:i16)
            n761 = Add(x=w1409, y=w1402) -> (x+y=w1404:i32)
            n762 = Bundle By Name(cluster=w1405, "Bottom"=w1404) -> (w1403:T44)
            n763 = property class="VI"(reference=w1408, error in=w1407, "Front Panel.PanelBounds"=w1403) -> (error out=w1406:errorcluster)  [unwired: 1 out]
          }
          frame False {
            n764 = Current VI's Path() -> (path=w1427:path)
            n765 = property on="Main tab control" class="TabCtl (strict)"() -> ("PaneHeight"=w1429:u32)  [unwired: 2 in, 2 out]
            n766 = property on="Expand/hide stream panel (Rec)" class="Bool (strict)"() -> ("Top"=w1431:i32)  [unwired: 2 in, 2 out]
            n767 = Open VI Reference(vi path=w1427) -> (vi reference=w1426:refnum<vi>, error out=w1425:errorcluster)  [unwired: 5 in]
            n768 = Subtract(x=w1431, y=w1417) -> (x-y=w1430:i32)
            n769 = property class="VI"(reference=w1426, error in=w1425) -> (reference out=w1423:refnum<vi>, error out=w1422:errorcluster, "Front Panel.PanelBounds"=w1420:T44)
            n770 = Subtract(x=w1429, y=w1417) -> (x-y=w1428:u32)
            n771 = property on="Expand/hide stream panel (Rec)" class="Bool (strict)"("Top"=w1430) -> ()  [unwired: 2 in, 2 out]
            n772 = property on="Main tab control" class="TabCtl (strict)"("PaneHeight"=w1428) -> ()  [unwired: 2 in, 2 out]
            n773 = Unbundle By Name(w1420) -> ("Bottom"=w1424:i16)
            n774 = Subtract(x=w1424, y=w1417) -> (x-y=w1419:i32)
            n775 = Bundle By Name(cluster=w1420, "Bottom"=w1419) -> (w1418:T44)
            n776 = property class="VI"(reference=w1423, error in=w1422, "Front Panel.PanelBounds"=w1418) -> (error out=w1421:errorcluster)  [unwired: 1 out]
          }
        }
        "FP size change error" <- w1400
      }
      event Key Down {
        n777 = event-data() -> ("VKey"=w1433:T45, "ScanCode"=w1432:i16)  [unwired: 1 in, 8 out]
        n778 = case shown="72, 75, 77, 80" w1432 {
          tunnel: w1433 -> [_ w1435]
          frame Default {
          }
          frame 72, 75, 77, 80 {
            n779 = Format Into String(format string="%s", w1435) -> (resulting string=w1434:string)  [unwired: 2 in, 1 out]
            n780 = global write "SW_Globals.vi" "Key_pressed"(w1434) -> ()
            n781 = local write "Key_pressed"(w1434) -> ()
          }
        }
      }
      event Key Up {
        n782 = event-data() -> ("ScanCode"=w1437:i16)  [unwired: 1 in, 6 out]
        n783 = case shown="72, 75, 77, 80" w1437 {
          frame Default {
          }
          frame 72, 75, 77, 80 {
            w1438 = ""
            n784 = global write "SW_Globals.vi" "Key_pressed"(w1438) -> ()
            n785 = local write "Key_pressed"(w1438) -> ()
          }
        }
      }
      event "Open serial port": Value Change {
        n786 = event-data() -> ()  [unwired: 1 in, 6 out]
        n787 = property on="Serial port opened" class="Bool (strict)"() -> ("Value"=w1439:bool)  [unwired: 2 in, 2 out]
        n788 = case shown="True" w1439 {
          frame False {
            w1445 = T46 4 items=["VISA Defaults"=0, "Exclusive Lock"=1, "Load Configured Settings"=4] ("Access Mode")
            n789 = property on="Serial OUT name" class="VISAName"("DisabledEnum"=T12."Disabled and Grayed Out" ("Disabled")) -> ("Value"=w1441:refnum<visa-resource-name>)  [unwired: 2 in, 2 out]
            n790 = VISA Open(access mode=w1445, VISA resource name=w1441) -> (VISA resource name=w1446:refnum<visa-resource-name>, error out=w1447:errorcluster)  [unwired: 3 in]
            n791 = property class="Instr"(reference=w1446, error in=w1447, "General Settings:Timeout Value"=u32 10) -> (reference out=w1442:refnum<visa-resource-name>, error out=w1443:errorcluster)
            n792 = case shown="Error" w1443 {
              tunnel: w1442 -> [_ w1455]
              frame No Error {
                w1448 = T11 [{"Numeric Control"=6603023, "Numeric Control"=6603023}, {"Numeric Control"=3381555, "Numeric Control"=3381555}, {"Numeric Control"=1976113, "Numeric Control"=8355711}, {"Numeric Control"=3355443, "Numeric Control"=6710886}]  # Button port ON colors
                n793 = property on="Expand/hide stream panel (Rec)" class="Bool (strict)"("Colors [4]"=w1448) -> ()  [unwired: 2 in, 2 out]
                n794 = property on="Serial port opened" class="Bool (strict)"("Value"=TRUE ("Serial port opened")) -> ()  [unwired: 2 in, 2 out]
                n795 = property on="Streaming" class="Bool (strict)"("DisabledEnum"=T12."Enabled" ("Disabled"), "Value"=FALSE ("Streaming")) -> ()  [unwired: 2 in, 2 out]
              }
              frame Error {
                w1452 = T11 [{"Numeric Control"=12369084, "Numeric Control"=12369084}, {"Numeric Control"=16757760, "Numeric Control"=16757760}, {"Numeric Control"=1976113, "Numeric Control"=8355711}, {"Numeric Control"=3355443, "Numeric Control"=6710886}]  # Button port OFF colors
                w1453 = FALSE ("Serial port opened")
                n796 = property on="Expand/hide stream panel (Rec)" class="Bool (strict)"("Colors [4]"=w1452) -> ()  [unwired: 2 in, 2 out]
                n797 = Not A Number/Path/Refnum?(number/path/refnum=w1455) -> (NaN/Path/Refnum?=w1456:bool)
                n798 = case shown="False" w1456 {
                  tunnel: w1455 -> [w1457 _]
                  frame False {
                    n799 = VISA Close(VISA resource name=w1457) -> ()  [unwired: 1 in, 1 out]
                  }
                  frame True {
                  }
                }
                n800 = property on="Serial port opened" class="Bool (strict)"("Value"=w1453) -> ()  [unwired: 2 in, 2 out]
                n801 = property on="Streaming" class="Bool (strict)"("DisabledEnum"=T12."Disabled and Grayed Out" ("Disabled"), "Value"=w1453) -> ()  [unwired: 2 in, 2 out]
              }
            }
          }
          frame True {
            w1458 = T11 [{"Numeric Control"=12369084, "Numeric Control"=12369084}, {"Numeric Control"=16757760, "Numeric Control"=16757760}, {"Numeric Control"=1976113, "Numeric Control"=8355711}, {"Numeric Control"=3355443, "Numeric Control"=6710886}]  # Button port OFF colors
            w1463 = FALSE ("Serial port opened")
            n802 = property on="Serial OUT name" class="VISAName"("DisabledEnum"=T12."Enabled" ("Disabled")) -> (error out=w1461:errorcluster, "Value"=w1462:refnum<visa-resource-name>)  [unwired: 2 in, 1 out]
            n803 = property on="Serial port opened" class="Bool (strict)"("Value"=w1463) -> ()  [unwired: 2 in, 2 out]
            n804 = VISA Close(VISA resource name=w1462, error in (no error)=w1461) -> (error out=w1460:errorcluster)
            n805 = property on="Streaming" class="Bool (strict)"("DisabledEnum"=T12."Disabled and Grayed Out" ("Disabled"), "Value"=w1463) -> ()  [unwired: 2 in, 2 out]
            n806 = property on="VISA streaming error out" class="Clust (strict)"("Value"=w1460) -> (error out=w1459:errorcluster)  [unwired: 2 in, 1 out]
            n807 = property on="Expand/hide stream panel (Rec)" class="Bool (strict)"(error in=w1459, "Colors [4]"=w1458) -> ()  [unwired: 1 in, 2 out]
          }
        }
      }
    }
    n808 = property on="Serial port opened" class="Bool (strict)"() -> ("Value"=w1363:bool)  [unwired: 2 in, 2 out]
    n809 = case shown="True" w1363 {
      tunnel: w1362 -> [_ w1394]
      tunnel: w1361 -> [_ w1371]
      frame False {
      }
      frame True {
        w1376 = "\t"
        n810 = call <extravilib>:"Read.vi"("channel"=w1394) -> ("element"=w1374:string[])  [unwired: 5 in, 5 out]
        "Latest frame" <- w1374
        n811 = Unbundle By Name(w1371) -> ("Recording now"=w1370:refnum<notifier>)
        n812 = Index Array "Timestamp"(array=w1374, index=5) -> (element=w1367:string)
        n813 = Index Array "R"(array=w1374, index=6) -> (element=w1388:string)
        n814 = Index Array "phi"(array=w1374, index=7) -> (element=w1387:string)
        n815 = Index Array "X"(array=w1374, index=9) -> (element=w1381:string)
        n816 = Index Array "w"(array=w1374, index=11) -> (element=w1379:string)
        n817 = Index Array "Y"(array=w1374, index=10) -> (element=w1380:string)
        n818 = Index Array "alpha"(array=w1374, index=8) -> (element=w1382:string)
        n819 = Index Array "Zone"(array=w1374, index=12) -> (element=w1377:string)
        n820 = Get Notifier Status(notifier=w1370) -> (current notification=w1368:bool)  [unwired: 1 in, 4 out]
        n821 = Select(t=w1367, s=w1368, f="00:00:00.000") -> (s? t:f=w1369:string)
        n822 = property on="Streaming" class="Bool (strict)"() -> ("Value"=w1392:bool)  [unwired: 2 in, 2 out]
        n823 = Index Array "Speed"(array=w1374, index=16) -> (element=w1373:string)
        n824 = Concatenate Strings(w1369, w1376, w1388, w1376, w1387, w1376, w1382, w1376, w1381, w1376, w1380, w1376, w1379, w1376, w1377, w1376, w1373, "\r\n") -> (w1391:string)
        n825 = property on="Output to the external terminal" class="Str"("Value"=w1391) -> ()  [unwired: 2 in, 2 out]
        n826 = case shown="True" w1392 {
          tunnel: w1391 -> [_ w1397]
          frame False {
          }
          frame True {
            n827 = property on="Serial OUT name" class="VISAName"() -> ("Value"=w1396:refnum<visa-resource-name>)  [unwired: 2 in, 2 out]
            n828 = VISA Write(VISA resource name=w1396, write buffer=w1397) -> (return count=→"Last send packet size, bytes":u32, error out=→"VISA streaming error out":errorcluster)  [unwired: 1 in, 1 out]
          }
        }
      }
    }
    n829 = node-c288() -> ()  [unwired: 1 in, 1 out]
  }
  n830 = disable-structure shown="Disabled" {
    frame Disabled {
      n831 = Greater Than 0?() -> (x > 0?=w1469:bool)  [unwired: 1 in]
      n832 = case shown="True" w1469 {
        tunnel: [_ w1472] -> w1470
        frame False {
        }
        frame True {
          n833 = local read "TTLs"() -> (w1473:u32[])
          n834 = Build Array(w1473, w1472) -> (w1471:u32[][])
          n835 = local write "TTLs"(w1471) -> ()
        }
      }
      "TTLs" <- u32[] [] ("TTLs")
    }
    frame Enabled {
    }
  }
  n836 = node-c288(w14) -> (w11:errorcluster)
  n837 = property on="Serial OUT name" class="VISAName"(error in=w11) -> (error out=w8:errorcluster, "Value"=w9:refnum<visa-resource-name>)  [unwired: 1 in, 1 out]
  n838 = VISA Close(VISA resource name=w9, error in (no error)=w8) -> (error out=→"Timed structure (Streaming) and VISA error(s)":errorcluster)
  n839 = node-c288(w49) -> ()  [unwired: 1 out]
  n840 = node-c288(w18, w40, 200 ("Priority")) -> (w42:T13)  [unwired: 1 in]
  n841 = Tick Count (ms)() -> (millisecond timer value=w66:u32)
  n842 = timed-loop {
    tunnel: w1 -> [w1487]
    tunnel: w17 -> [w1474]
    tunnel: w36 -> [w1485]
    tunnel: w66 -> [w1484]
    tunnel: w65 -> [w1483]
    timing: w42 -> [_]
    timing-out: [_] -> w41
    tunnel: w40 -> [w1476]
    i -> [w1486]
    stop <- w1480 stop-if-true
    n843 = node-c288() -> ()  [unwired: 1 in, 1 out]
    n844 = Unbundle By Name(w1474) -> ("Complete stop"=w1481:refnum<notifier>)
    n845 = property on="Main tab control" class="TabCtl (strict)"(error in=w1485) -> (error out=w1475:errorcluster, "Value"=w1488:enum32{"Settings", "Recording", "Analysis"})  [unwired: 1 in, 1 out]
    n846 = Send Notification(notification="Stop Button", notifier=w1481) -> (notifier out=w1477:refnum<notifier>, error out=w1478:errorcluster)  [unwired: 1 in]
    n847 = case shown="\"Recording\"" w1488 {
      tunnel: w1475 -> [w1495 _ _]
      tunnel: w1487 -> [_ w2238 _]
      tunnel: w1476 -> [_ w2240 w2726]
      tunnel: w1486 -> [_ _ _]
      tunnel: w1474 -> [w1491 w2173 w2728]
      tunnel: w1484 -> [_ w2235 _]
      tunnel: w1483 -> [_ w2228 _]
      frame "Settings", Default {
        n848 = flat-sequence {
          tunnel: w1495 -> [w1499]
          tunnel: [w1499] -> w1492
          tunnel: [w1546] -> w1493
          tunnel: w1492 -> [w1546]
          tunnel: [w1905] -> w1494
          tunnel: w1493 -> [w1905]
          tunnel: w1494 -> [w1947]
          tunnel: w1491 -> [w1942]
          frame #0 {
            n849 = property on="IO paramaters loaded from file" class="Bool (strict)"() -> ("Value"=w1496:bool)  [unwired: 2 in, 2 out]
            n850 = Or(x="Set IO config", y=w1496) -> (x .or. y?=w1497:bool)
            n851 = case shown="True" w1497 {
              tunnel: w1496 -> [_ w1501]
              frame False {
              }
              frame True {
                w1513 = u16 4 ("y")
                n852 = global read "SW_Globals.vi" "IO parameters cluster"() -> (w1507:T2)
                n853 = local read "Sync capability"() -> (w1506:u8)
                n854 = case shown="False" w1501 {
                  tunnel: w1507 -> [w1533 w1536]
                  tunnel: w1506 -> [w1534 _]
                  tunnel: [w1532 w1537] -> w1505
                  tunnel: [w1531 w1535] -> w1504
                  frame False {
                    n855 = call "HW_set_IO_ports_3-pos.vi"("Sync capability"=w1534, "Sync parameters cluster input"=w1533) -> ("Sync parameters cluster output"=w1532:T2)
                    n856 = Equal?(x=w1533, y=w1532) -> (x = y?=w1531:T50)
                  }
                  frame True {
                    n857 = property on="IO parameters loaded cluster" class="Clust (strict)"() -> ("Value"=w1537:T2)  [unwired: 2 in, 2 out]
                    n858 = Equal?(x=w1536, y=w1537) -> (x = y?=w1535:T50)
                  }
                }
                n859 = Greater Than 0?(x=w1506) -> (x > 0?=w1516:bool)
                n860 = global read "SW_Globals.vi" "VISA resource name"() -> (w1509:refnum<visa-resource-name>)
                n861 = Unbundle By Name(w1505) -> ("IO 1 configuration"=w1511:u16, "IO 2 configuration"=w1512:u16)
                n862 = global write "SW_Globals.vi" "IO parameters cluster"(w1505) -> ()
                n863 = Cluster To Array(cluster=w1505) -> (array=w1500:u16[])
                n864 = call "SW_get_IO_ports_representation.vi"("Sync parameters cluster input"=w1505) -> ("IO status indicator"=w1528:T37)
                n865 = call "SW_get_config_for_Start_Stop_pulses.vi"("Sync parameters cluster input"=w1505) -> ("Start/Stop out pulses config"=w1522:u32, "Start/Stop in config"=w1521:u32, "Start/Stop in config bin"=w1520:bool[], "Start/Stop out pulses config bin"=w1519:bool[])
                n866 = call "SW_get_config_of_Zones_and_IO.vi"("Sync parameters cluster input"=w1505) -> ("Zones out config bin"=w1518:bool[], "Ports IO config (OUT is FALSE)"=w1517:bool[], "IO inversion config."=w1508:u16)  [unwired: 1 out]
                n867 = property on="Start/Stop out pulses config" class="DigNum (strict)"("Value"=w1522) -> ()  [unwired: 2 in, 2 out]
                n868 = property on="Start/Stop in config" class="DigNum (strict)"("Value"=w1521) -> ()  [unwired: 2 in, 2 out]
                n869 = global write "SW_Globals.vi" "IO ports config"(w1517) -> ()
                n870 = global write "SW_Globals.vi" "IO inversion config."(w1508) -> ()
                n871 = global write "SW_Globals.vi" "Zones out config bin"(w1518) -> ()
                n872 = Equal?(x=w1511, y=w1513) -> (x = y?=w1514:bool)
                n873 = Equal?(x=w1512, y=w1513) -> (x = y?=w1515:bool)
                n874 = call "HW_Set_IO_Dir_on_ECU.vi"("IO ports config"=w1517, "VISA resource name"=w1509, "IO inversion config."=w1508) -> ("error out"=w1510:errorcluster)  [unwired: 1 in, 1 out]
                n875 = Cluster To Array(cluster=w1504) -> (array=w1526:bool[])
                n876 = To Variant(anything=w1528) -> (Variant=w1527:variant)
                n877 = Flatten To JSON(anything=w1500) -> (JSON string=w1530:string, 11:w1529:errorcluster)  [unwired: 2 in]
                n878 = global write "SW_Globals.vi" "Start/Stop in config bin"(w1520) -> ()
                n879 = case shown="True" w1516 {
                  tunnel: w1509 -> [_ w1540]
                  tunnel: w1510 -> [_ w1541]
                  tunnel: w1514 -> [_ w1539]
                  tunnel: w1515 -> [_ w1538]
                  frame False {
                  }
                  frame True {
                    n880 = call "HW_Set_SYNC_Status.vi"("error in (no error)"=w1541, "SYNC 2"=w1539, "SYNC 1"=w1538, "VISA Resource name IN"=w1540) -> ()  [unwired: 6 in, 2 out]
                  }
                }
                n881 = property on="IO status indicator" class="Clust"("Value"=w1527) -> ()  [unwired: 2 in, 2 out]
                n882 = property on="IO parameters string" class="Str"(error in=w1529, "Value"=w1530) -> ()  [unwired: 1 in, 2 out]
                n883 = Not(x=w1526) -> (.not. x?=w1525:bool[])
                n884 = global write "SW_Globals.vi" "Start/Stop out pulses config bin"(w1519) -> ()
                n885 = Boolean Array To Number(Boolean array=w1525) -> (number=w1524:u32)
                n886 = Not(x=w1501) -> (.not. x?=w1502:bool)
                n887 = Greater Than 0?(x=w1524) -> (x > 0?=w1523:bool)
                n888 = And(x=w1523, y=w1502) -> (x .and. y?=w1503:bool)
                n889 = case shown="True" w1503 {
                  frame False {
                    n890 = property on="IO paramaters loaded from file" class="Bool (strict)"("Value"=FALSE ("IO paramaters loaded from file")) -> ()  [unwired: 2 in, 2 out]
                  }
                  frame True {
                    n891 = property on="IO paramaters loaded from file" class="Bool (strict)"("Value"=FALSE ("IO paramaters loaded from file")) -> ()  [unwired: 2 in, 2 out]
                    n892 = property on="Changed IO" class="Bool (strict)"("Val(Sgnl)"=TRUE ("Value (Signaling)")) -> ()  [unwired: 2 in, 2 out]
                  }
                }
              }
            }
          }
          frame #1 {
            n893 = event shown="[2] \"N segments BORDER\", \"N segments MIDFIELD\": Value Change" {
              selector: _ -> [_ _ _ _ _ _ _ _ _]
              dyn-events: _ -> [_ _ _ _ _ _ _ _ _]
              timeout: 1 -> [_ _ _ _ _ _ _ _ _]
              event Timeout {
                n894 = event-data() -> ()  [unwired: 1 in, 3 out]
              }
              event "Segments diagram": Mouse Down {
                n895 = event-data() -> ("Coords"=→"Coords":T4, "Button"=→"Button":u16)  [unwired: 1 in, 6 out]
              }
              event "N segments BORDER", "N segments MIDFIELD": Value Change {
                n896 = event-data() -> ()  [unwired: 1 in, 6 out]
                n897 = global read "SW_Globals.vi" "IO parameters cluster"() -> (w1558:T2)
                n898 = Unbundle By Name(w1558) -> ("SYNC configuration"=w1557:u16, "IO 1 configuration"=w1554:u16, "IO 2 configuration"=w1553:u16)
                n899 = property on="N segments BORDER" class="DigNum (strict)"() -> (error out=w1563:errorcluster, "Value"=w1566:u8)  [unwired: 2 in, 1 out]
                n900 = call "SW_Gen_Available_TTL_outputs_array.vi"("IO 2 configuration"=w1553, "IO 1 configuration"=w1554, "SYNC configuration"=w1557) -> ("Available TTL outputs array"=w1552:cluster{"String":string, "Value":i32}[])
                n901 = property on="N segments MIDFIELD" class="DigNum (strict)"(error in=w1563) -> (error out=w1562:errorcluster, "Value"=w1565:u8)  [unwired: 1 in, 1 out]
                n902 = Index Array(array=w1552, index=0) -> (element=w1555:cluster{"String":string, "Value":i32})
                n903 = global read "SW_Globals.vi" "Zone-based stimulus presets"() -> (w1560:T51)
                n904 = property on="Zone-based stimulus setup" class="RadioBtnsControl (strict)"(error in=w1562) -> ("Controls[]"=w1564:refnum<vi>[])  [unwired: 1 in, 2 out]
                n905 = property on="TTL out" class="Ring (strict)"("StringsAndValues[]"=w1552) -> ()  [unwired: 2 in, 2 out]
                n906 = Compound Arithmetic op=ADD(w1566, w1565, u8 1 ("value")) -> (w1561:u8)
                n907 = Unbundle By Name(w1555) -> ("Value"=w1559:i32)
                n908 = for {
                  tunnel: w1564 -> [w1583] mode=indexing
                  tunnel: w1561 -> [w1574]
                  tunnel: w1560 -> [w1579]
                  tunnel: w1559 -> [w1578]
                  tunnel: [w1577] -> w1550 mode=indexing
                  i -> [w1573]
                  n909 = Increment(x=w1573) -> (x+1=w1575:i32)
                  n910 = Greater Or Equal?(x=w1574, y=w1575) -> (x >= y?=w1572:bool)
                  n911 = Select(t=T12."Enabled" ("Disabled"), s=w1572, f=T12."Disabled and Grayed Out") -> (s? t:f=w1581:T12)
                  n912 = property class="Ctl"(reference=w1583, "DisabledEnum"=w1581) -> (reference out=w1576:refnum<vi>)  [unwired: 1 in, 1 out]
                  n913 = case shown="True" w1572 {
                    tunnel: w1579 -> [_ w1593]
                    tunnel: w1578 -> [w1591 _]
                    tunnel: [w1589 w1592] -> w1577
                    tunnel: w1576 -> [w1584 _]
                    frame False {
                      w1586 = refnum<vi> refnum  # Boolean
                      n914 = Bundle By Name(cluster=T47 {"Event type"=0, "Cond., s"=0.0, "Stim., s"=0.0, "Set/Clear"=FALSE, "TTL out N"=1, "Stim. has been set"=FALSE} ("Cluster of the stimuls settings"), "TTL out N"=w1591) -> (w1589:T47)
                      n915 = To More Specific Class(target class=w1586, reference=w1584) -> (specific class reference=w1585:refnum<vi>)  [unwired: 1 in, 1 out]
                      n916 = property class="Bool"(reference=w1585, "Colors [4]"=T11 [{"Numeric Control"=12369084, "Numeric Control"=12369084}, {"Numeric Control"=6603023, "Numeric Control"=6603023}, {"Numeric Control"=1976113, "Numeric Control"=1976113}, {"Numeric Control"=2575993, "Numeric Control"=2575993}] ("Colors [4] 2"), "Value"=FALSE) -> ()  [unwired: 1 in, 2 out]
                    }
                    frame True {
                      n917 = Index Array(array=w1593) -> (element=w1592:T47)  [unwired: 1 in]
                    }
                  }
                }
                n918 = for {
                  tunnel: w1550 -> [w1571] mode=indexing
                  tunnel: [w1568] -> w1551 mode=indexing if=w1569
                  i -> [w1570]
                  n919 = Unbundle By Name(w1571) -> ("Stim. has been set"=w1569:bool)
                  n920 = To Unsigned Byte Integer(number=w1570) -> (unsigned 8bit integer=w1568:u8)
                }
                n921 = global write "SW_Globals.vi" "Zone-based stimulus presets"(w1550) -> ()
                n922 = property on="Stimulus presets" class="Arr (strict)"("Value"=w1550) -> ()  [unwired: 2 in, 2 out]
                n923 = global write "SW_Globals.vi" "Regions to track"(w1551) -> ()
              }
              event "Zone-based stimulus setup": Value Change {
                n924 = event-data() -> ("NewVal"=w1595:T8)  [unwired: 1 in, 5 out]
                n925 = To Unsigned Byte Integer(number=w1595) -> (unsigned 8bit integer=w1594:u8)
                n926 = case shown="1.." w1594 {
                  selector: w1594 -> [w1596 w1599]
                  frame 0, Default {
                    n927 = Build Array(w1596) -> (w1598:u8[])
                    n928 = property on="Stimulus presets" class="Arr (strict)"("Index Values"=w1598, "DisabledEnum"=T12."Disabled and Grayed Out" ("Disabled")) -> ()  [unwired: 2 in, 2 out]
                  }
                  frame 1.. {
                    n929 = Build Array(w1599) -> (w1601:u8[])
                    n930 = property on="Stimulus presets" class="Arr (strict)"("Index Values"=w1601, "DisabledEnum"=T12."Enabled" ("Disabled")) -> ()  [unwired: 2 in, 2 out]
                  }
                }
              }
              event "Stimulus presets", "Adv. Stim. set": Value Change {
                n931 = event-data() -> ()  [unwired: 1 in, 6 out]
                n932 = property on="Stimulus presets" class="Arr (strict)"() -> ("Value"=w1605:T7)  [unwired: 2 in, 2 out]
                n933 = disable-structure shown="Disabled" {
                  frame Disabled {
                    n934 = case shown="1" {
                      selector: _ -> [_ _ _ _ _ _ _ _ _ _ _ _ _ _]
                      tunnel: _ -> [_ w1632 w1636 w1640 w1644 w1648 w1652 w1656 w1660 w1664 w1668 w1672 w1676 w1680]
                      frame 0, Default {
                      }
                      frame 1 {
                        n935 = property on="Colors for Stim. setup" class="Arr (strict)"() -> ("Value"=w1631:T3)  [unwired: 2 in, 2 out]
                        n936 = Select(t=w1631, s=w1632, f=T11 [{"Numeric Control"=12369084, "Numeric Control"=12369084}, {"Numeric Control"=6603023, "Numeric Control"=6603023}, {"Numeric Control"=1976113, "Numeric Control"=1976113}, {"Numeric Control"=2575993, "Numeric Control"=2575993}] ("Colors [4] 2")) -> (s? t:f=w1634:T11)
                        n937 = property on="Zone 01" class="Bool (strict)"("Colors [4]"=w1634) -> ()  [unwired: 2 in, 2 out]
                      }
                      frame 2 {
                        n938 = property on="Colors for Stim. setup" class="Arr (strict)"() -> ("Value"=w1635:T3)  [unwired: 2 in, 2 out]
                        n939 = Select(t=w1635, s=w1636, f=T11 [{"Numeric Control"=12369084, "Numeric Control"=12369084}, {"Numeric Control"=6603023, "Numeric Control"=6603023}, {"Numeric Control"=1976113, "Numeric Control"=1976113}, {"Numeric Control"=2575993, "Numeric Control"=2575993}] ("Colors [4] 2")) -> (s? t:f=w1638:T11)
                        n940 = property on="Zone 02" class="Bool (strict)"("Colors [4]"=w1638) -> ()  [unwired: 2 in, 2 out]
                      }
                      frame 3 {
                        n941 = property on="Colors for Stim. setup" class="Arr (strict)"() -> ("Value"=w1639:T3)  [unwired: 2 in, 2 out]
                        n942 = Select(t=w1639, s=w1640, f=T11 [{"Numeric Control"=12369084, "Numeric Control"=12369084}, {"Numeric Control"=6603023, "Numeric Control"=6603023}, {"Numeric Control"=1976113, "Numeric Control"=1976113}, {"Numeric Control"=2575993, "Numeric Control"=2575993}] ("Colors [4] 2")) -> (s? t:f=w1642:T11)
                        n943 = property on="Zone 03" class="Bool (strict)"("Colors [4]"=w1642) -> ()  [unwired: 2 in, 2 out]
                      }
                      frame 4 {
                        n944 = property on="Colors for Stim. setup" class="Arr (strict)"() -> ("Value"=w1643:T3)  [unwired: 2 in, 2 out]
                        n945 = Select(t=w1643, s=w1644, f=T11 [{"Numeric Control"=12369084, "Numeric Control"=12369084}, {"Numeric Control"=6603023, "Numeric Control"=6603023}, {"Numeric Control"=1976113, "Numeric Control"=1976113}, {"Numeric Control"=2575993, "Numeric Control"=2575993}] ("Colors [4] 2")) -> (s? t:f=w1646:T11)
                        n946 = property on="Zone 04" class="Bool (strict)"("Colors [4]"=w1646) -> ()  [unwired: 2 in, 2 out]
                      }
                      frame 5 {
                        n947 = property on="Colors for Stim. setup" class="Arr (strict)"() -> ("Value"=w1647:T3)  [unwired: 2 in, 2 out]
                        n948 = Select(t=w1647, s=w1648, f=T11 [{"Numeric Control"=12369084, "Numeric Control"=12369084}, {"Numeric Control"=6603023, "Numeric Control"=6603023}, {"Numeric Control"=1976113, "Numeric Control"=1976113}, {"Numeric Control"=2575993, "Numeric Control"=2575993}] ("Colors [4] 2")) -> (s? t:f=w1650:T11)
                        n949 = property on="Zone 05" class="Bool (strict)"("Colors [4]"=w1650) -> ()  [unwired: 2 in, 2 out]
                      }
                      frame 6 {
                        n950 = property on="Colors for Stim. setup" class="Arr (strict)"() -> ("Value"=w1651:T3)  [unwired: 2 in, 2 out]
                        n951 = Select(t=w1651, s=w1652, f=T11 [{"Numeric Control"=12369084, "Numeric Control"=12369084}, {"Numeric Control"=6603023, "Numeric Control"=6603023}, {"Numeric Control"=1976113, "Numeric Control"=1976113}, {"Numeric Control"=2575993, "Numeric Control"=2575993}] ("Colors [4] 2")) -> (s? t:f=w1654:T11)
                        n952 = property on="Zone 06" class="Bool (strict)"("Colors [4]"=w1654) -> ()  [unwired: 2 in, 2 out]
                      }
                      frame 7 {
                        n953 = property on="Colors for Stim. setup" class="Arr (strict)"() -> ("Value"=w1655:T3)  [unwired: 2 in, 2 out]
                        n954 = Select(t=w1655, s=w1656, f=T11 [{"Numeric Control"=12369084, "Numeric Control"=12369084}, {"Numeric Control"=6603023, "Numeric Control"=6603023}, {"Numeric Control"=1976113, "Numeric Control"=1976113}, {"Numeric Control"=2575993, "Numeric Control"=2575993}] ("Colors [4] 2")) -> (s? t:f=w1658:T11)
                        n955 = property on="Zone 07" class="Bool (strict)"("Colors [4]"=w1658) -> ()  [unwired: 2 in, 2 out]
                      }
                      frame 8 {
                        n956 = property on="Colors for Stim. setup" class="Arr (strict)"() -> ("Value"=w1659:T3)  [unwired: 2 in, 2 out]
                        n957 = Select(t=w1659, s=w1660, f=T11 [{"Numeric Control"=12369084, "Numeric Control"=12369084}, {"Numeric Control"=6603023, "Numeric Control"=6603023}, {"Numeric Control"=1976113, "Numeric Control"=1976113}, {"Numeric Control"=2575993, "Numeric Control"=2575993}] ("Colors [4] 2")) -> (s? t:f=w1662:T11)
                        n958 = property on="Zone 08" class="Bool (strict)"("Colors [4]"=w1662) -> ()  [unwired: 2 in, 2 out]
                      }
                      frame 9 {
                        n959 = property on="Colors for Stim. setup" class="Arr (strict)"() -> ("Value"=w1663:T3)  [unwired: 2 in, 2 out]
                        n960 = Select(t=w1663, s=w1664, f=T11 [{"Numeric Control"=12369084, "Numeric Control"=12369084}, {"Numeric Control"=6603023, "Numeric Control"=6603023}, {"Numeric Control"=1976113, "Numeric Control"=1976113}, {"Numeric Control"=2575993, "Numeric Control"=2575993}] ("Colors [4] 2")) -> (s? t:f=w1666:T11)
                        n961 = property on="Zone 09" class="Bool (strict)"("Colors [4]"=w1666) -> ()  [unwired: 2 in, 2 out]
                      }
                      frame 10 {
                        n962 = property on="Colors for Stim. setup" class="Arr (strict)"() -> ("Value"=w1667:T3)  [unwired: 2 in, 2 out]
                        n963 = Select(t=w1667, s=w1668, f=T11 [{"Numeric Control"=12369084, "Numeric Control"=12369084}, {"Numeric Control"=6603023, "Numeric Control"=6603023}, {"Numeric Control"=1976113, "Numeric Control"=1976113}, {"Numeric Control"=2575993, "Numeric Control"=2575993}] ("Colors [4] 2")) -> (s? t:f=w1670:T11)
                        n964 = property on="Zone 10" class="Bool (strict)"("Colors [4]"=w1670) -> ()  [unwired: 2 in, 2 out]
                      }
                      frame 11 {
                        n965 = property on="Colors for Stim. setup" class="Arr (strict)"() -> ("Value"=w1671:T3)  [unwired: 2 in, 2 out]
                        n966 = Select(t=w1671, s=w1672, f=T11 [{"Numeric Control"=12369084, "Numeric Control"=12369084}, {"Numeric Control"=6603023, "Numeric Control"=6603023}, {"Numeric Control"=1976113, "Numeric Control"=1976113}, {"Numeric Control"=2575993, "Numeric Control"=2575993}] ("Colors [4] 2")) -> (s? t:f=w1674:T11)
                        n967 = property on="Zone 11" class="Bool (strict)"("Colors [4]"=w1674) -> ()  [unwired: 2 in, 2 out]
                      }
                      frame 12 {
                        n968 = property on="Colors for Stim. setup" class="Arr (strict)"() -> ("Value"=w1675:T3)  [unwired: 2 in, 2 out]
                        n969 = Select(t=w1675, s=w1676, f=T11 [{"Numeric Control"=12369084, "Numeric Control"=12369084}, {"Numeric Control"=6603023, "Numeric Control"=6603023}, {"Numeric Control"=1976113, "Numeric Control"=1976113}, {"Numeric Control"=2575993, "Numeric Control"=2575993}] ("Colors [4] 2")) -> (s? t:f=w1678:T11)
                        n970 = property on="Zone 12" class="Bool (strict)"("Colors [4]"=w1678) -> ()  [unwired: 2 in, 2 out]
                      }
                      frame 13 {
                        n971 = property on="Colors for Stim. setup" class="Arr (strict)"() -> ("Value"=w1679:T3)  [unwired: 2 in, 2 out]
                        n972 = Select(t=w1679, s=w1680, f=T11 [{"Numeric Control"=12369084, "Numeric Control"=12369084}, {"Numeric Control"=6603023, "Numeric Control"=6603023}, {"Numeric Control"=1976113, "Numeric Control"=1976113}, {"Numeric Control"=2575993, "Numeric Control"=2575993}] ("Colors [4] 2")) -> (s? t:f=w1682:T11)
                        n973 = property on="Zone 13" class="Bool (strict)"("Colors [4]"=w1682) -> ()  [unwired: 2 in, 2 out]
                      }
                    }
                  }
                  frame Enabled {
                  }
                }
                n974 = property on="Stimulus presets" class="Arr (strict)"() -> ("Index Values"=w1620:u32[])  [unwired: 2 in, 2 out]
                n975 = Index Array(array=w1620, index=0) -> (element=w1606:u32)
                n976 = Index Array(array=w1605, index=w1606) -> (element=w1614:T52)
                n977 = property on="Zone-based stimulus setup" class="RadioBtnsControl (strict)"() -> ("Value"=w1618:T8)  [unwired: 2 in, 2 out]
                n978 = Unbundle By Name(w1614) -> ("Set/Clear"=w1615:bool, "Time, s"=w1610:sgl, "Stimulus, s"=w1608:sgl)
                n979 = Format Into String(w1618) -> ()  [unwired: 3 in, 2 out]
                n980 = Greater Than 0?(x=w1610) -> (x > 0?=w1617:bool)
                n981 = Greater Than 0?(x=w1608) -> (x > 0?=w1616:bool)
                n982 = expression code="floor(x * 100) / 100"(w1610) -> (w1609:sgl)
                n983 = expression code="floor(x * 100) / 100"(w1608) -> (w1607:sgl)
                n984 = To Unsigned Byte Integer(number=w1618) -> (unsigned 8bit integer=w1603:u8)
                n985 = Compound Arithmetic op=AND(w1615, w1617, w1616) -> (w1604:bool)
                n986 = Greater Than 0?(x=w1603) -> (x > 0?=w1602:bool)
                n987 = Bundle By Name(cluster=w1614, "Stim. has been set"=w1604, "Set/Clear"=w1604, "Time, s"=w1609, "Stimulus, s"=w1607) -> (w1613:T52)
                n988 = case shown="True" w1602 {
                  tunnel: w1604 -> [_ w1624]
                  tunnel: w1603 -> [_ w1623]
                  frame False {
                  }
                  frame True {
                    w1628 = refnum<vi> refnum  # Boolean
                    n989 = property on="Colors for Stim. setup" class="Arr (strict)"() -> ("Value"=w1625:T3)  [unwired: 2 in, 2 out]
                    n990 = Decrement(x=w1623) -> (x-1=w1622:u8)
                    n991 = Select(t=w1625, s=w1624, f=T11 [{"Numeric Control"=12369084, "Numeric Control"=12369084}, {"Numeric Control"=6603023, "Numeric Control"=6603023}, {"Numeric Control"=1976113, "Numeric Control"=1976113}, {"Numeric Control"=2575993, "Numeric Control"=2575993}] ("Colors [4] 2")) -> (s? t:f=w1630:T11)
                    n992 = property on="Zone-based stimulus setup" class="RadioBtnsControl (strict)"() -> ("Controls[]"=w1621:refnum<vi>[])  [unwired: 2 in, 2 out]
                    n993 = Index Array(array=w1621, index=w1622) -> (element=w1627:refnum<vi>)
                    n994 = To More Specific Class(target class=w1628, reference=w1627) -> (specific class reference=w1629:refnum<vi>)  [unwired: 1 in, 1 out]
                    n995 = property class="Bool"(reference=w1629, "Colors [4]"=w1630) -> ()  [unwired: 1 in, 2 out]
                  }
                }
                n996 = Replace Array Subset(array=w1605, new element=w1613, index=w1606) -> (w1611:T7)
                n997 = global write "SW_Globals.vi" "Zone-based stimulus presets"(w1611) -> ()
                n998 = property on="Stimulus presets" class="Arr (strict)"("Value"=w1611) -> ()  [unwired: 2 in, 2 out]
                n999 = for {
                  tunnel: w1611 -> [w1686] mode=indexing
                  tunnel: [w1683] -> w1612 mode=indexing if=w1684
                  i -> [w1685]
                  n1000 = Unbundle By Name(w1686) -> ("Stim. has been set"=w1684:bool)
                  n1001 = To Unsigned Byte Integer(number=w1685) -> (unsigned 8bit integer=w1683:u8)
                }
                n1002 = global write "SW_Globals.vi" "Regions to track"(w1612) -> ()
              }
              event "Reset stimuli", "Changed IO": Value Change {
                n1003 = event-data() -> ("OldVal"=w1688:bool, "NewVal"=w1689:bool)  [unwired: 1 in, 4 out]
                n1004 = property on="Reset stimuli" class="Bool (strict)"("Value"=w1688) -> ()  [unwired: 2 in, 2 out]
                n1005 = property on="Changed IO" class="Bool (strict)"("Value"=FALSE ("Changed IO")) -> ()  [unwired: 2 in, 2 out]
                n1006 = case shown="True" w1689 {
                  selector: w1689 -> [_ w1713]
                  frame False {
                  }
                  frame True {
                    w1701 = T11 [{"Numeric Control"=9868950, "Numeric Control"=15790320}, {"Numeric Control"=8388608, "Numeric Control"=8388608}, {"Numeric Control"=4934475, "Numeric Control"=7895160}, {"Numeric Control"=994319, "Numeric Control"=1657881}]  # TTL IO In colors
                    w1702 = T11 [{"Numeric Control"=9868950, "Numeric Control"=15790320}, {"Numeric Control"=1988894, "Numeric Control"=3381555}, {"Numeric Control"=4934475, "Numeric Control"=7895160}, {"Numeric Control"=994319, "Numeric Control"=1657881}]  # TTL IO Out colors
                    n1007 = global write "SW_Globals.vi" "Regions to track"(u8[] []) -> ()
                    n1008 = global read "SW_Globals.vi" "IO ports config"() -> (w1700:bool[])
                    n1009 = Index Array(array=w1700, index=1) -> (element=w1705:bool)
                    n1010 = Index Array(array=w1700, index=2) -> (element=w1704:bool)
                    n1011 = Index Array(array=w1700, index=3) -> (element=w1703:bool)
                    n1012 = Index Array(array=w1700, index=0) -> (element=w1706:bool)
                    n1013 = Select(t=w1701, s=w1705, f=w1702) -> (s? t:f=w1698:T11)
                    n1014 = Select(t=w1701, s=w1704, f=w1702) -> (s? t:f=w1697:T11)
                    n1015 = Select(t=w1701, s=w1703, f=w1702) -> (s? t:f=w1696:T11)
                    n1016 = Select(t=w1701, s=w1706, f=w1702) -> (s? t:f=w1699:T11)
                    n1017 = property on="TTL IO 2 (analysis)" class="Bool"("Colors [4]"=w1698) -> ()  [unwired: 2 in, 2 out]
                    n1018 = property on="TTL IO 2 (recording)" class="Bool (strict)"("Colors [4]"=w1698) -> ()  [unwired: 2 in, 2 out]
                    n1019 = property on="TTL IO 3 (analysis)" class="Bool"("Colors [4]"=w1697) -> ()  [unwired: 2 in, 2 out]
                    n1020 = property on="TTL IO 3 (recording)" class="Bool (strict)"("Colors [4]"=w1697) -> ()  [unwired: 2 in, 2 out]
                    n1021 = property on="TTL IO 4 (analysis)" class="Bool"("Colors [4]"=w1696) -> ()  [unwired: 2 in, 2 out]
                    n1022 = property on="TTL IO 4 (recording)" class="Bool (strict)"("Colors [4]"=w1696) -> ()  [unwired: 2 in, 2 out]
                    n1023 = property on="TTL IO 1 (analysis)" class="Bool"("Colors [4]"=w1699) -> ()  [unwired: 2 in, 2 out]
                    n1024 = property on="TTL IO 1 (recording)" class="Bool (strict)"("Colors [4]"=w1699) -> ()  [unwired: 2 in, 2 out]
                    n1025 = global read "SW_Globals.vi" "IO parameters cluster"() -> (w1712:T2)
                    n1026 = Unbundle By Name(w1712) -> ("SYNC configuration"=w1711:u16, "IO 1 configuration"=w1691:u16, "IO 2 configuration"=w1690:u16)
                    n1027 = call "SW_Gen_Available_TTL_outputs_array.vi"("IO 2 configuration"=w1690, "IO 1 configuration"=w1691, "SYNC configuration"=w1711) -> ("Available TTL outputs array"=w1695:cluster{"String":string, "Value":i32}[])
                    n1028 = property on="TTL out" class="Ring (strict)"("StringsAndValues[]"=w1695) -> ()  [unwired: 2 in, 2 out]
                    n1029 = disable-structure shown="Disabled" {
                      frame Disabled {
                        n1030 = case shown="6" {
                          selector: _ -> [_ _ _ _ _ _ _ _ _ _ _ _ _ _]
                          frame 0, Default {
                          }
                          frame 1 {
                            n1031 = property on="Zone 01" class="Bool (strict)"("Colors [4]"=T11 [{"Numeric Control"=12369084, "Numeric Control"=12369084}, {"Numeric Control"=6603023, "Numeric Control"=6603023}, {"Numeric Control"=1976113, "Numeric Control"=1976113}, {"Numeric Control"=2575993, "Numeric Control"=2575993}] ("Colors [4] 2"), "Value"=FALSE) -> ()  [unwired: 2 in, 2 out]
                          }
                          frame 2 {
                            n1032 = property on="Zone 02" class="Bool (strict)"("Colors [4]"=T11 [{"Numeric Control"=12369084, "Numeric Control"=12369084}, {"Numeric Control"=6603023, "Numeric Control"=6603023}, {"Numeric Control"=1976113, "Numeric Control"=1976113}, {"Numeric Control"=2575993, "Numeric Control"=2575993}] ("Colors [4] 2"), "Value"=FALSE) -> ()  [unwired: 2 in, 2 out]
                          }
                          frame 3 {
                            n1033 = property on="Zone 03" class="Bool (strict)"("Colors [4]"=T11 [{"Numeric Control"=12369084, "Numeric Control"=12369084}, {"Numeric Control"=6603023, "Numeric Control"=6603023}, {"Numeric Control"=1976113, "Numeric Control"=1976113}, {"Numeric Control"=2575993, "Numeric Control"=2575993}] ("Colors [4] 2"), "Value"=FALSE) -> ()  [unwired: 2 in, 2 out]
                          }
                          frame 4 {
                            n1034 = property on="Zone 04" class="Bool (strict)"("Colors [4]"=T11 [{"Numeric Control"=12369084, "Numeric Control"=12369084}, {"Numeric Control"=6603023, "Numeric Control"=6603023}, {"Numeric Control"=1976113, "Numeric Control"=1976113}, {"Numeric Control"=2575993, "Numeric Control"=2575993}] ("Colors [4] 2"), "Value"=FALSE) -> ()  [unwired: 2 in, 2 out]
                          }
                          frame 5 {
                            n1035 = property on="Zone 05" class="Bool (strict)"("Colors [4]"=T11 [{"Numeric Control"=12369084, "Numeric Control"=12369084}, {"Numeric Control"=6603023, "Numeric Control"=6603023}, {"Numeric Control"=1976113, "Numeric Control"=1976113}, {"Numeric Control"=2575993, "Numeric Control"=2575993}] ("Colors [4] 2"), "Value"=FALSE) -> ()  [unwired: 2 in, 2 out]
                          }
                          frame 6 {
                            n1036 = property on="Zone 06" class="Bool (strict)"("Colors [4]"=T11 [{"Numeric Control"=12369084, "Numeric Control"=12369084}, {"Numeric Control"=6603023, "Numeric Control"=6603023}, {"Numeric Control"=1976113, "Numeric Control"=1976113}, {"Numeric Control"=2575993, "Numeric Control"=2575993}] ("Colors [4] 2"), "Value"=FALSE) -> ()  [unwired: 2 in, 2 out]
                          }
                          frame 7 {
                            n1037 = property on="Zone 07" class="Bool (strict)"("Colors [4]"=T11 [{"Numeric Control"=12369084, "Numeric Control"=12369084}, {"Numeric Control"=6603023, "Numeric Control"=6603023}, {"Numeric Control"=1976113, "Numeric Control"=1976113}, {"Numeric Control"=2575993, "Numeric Control"=2575993}] ("Colors [4] 2"), "Value"=FALSE) -> ()  [unwired: 2 in, 2 out]
                          }
                          frame 8 {
                            n1038 = property on="Zone 08" class="Bool (strict)"("Colors [4]"=T11 [{"Numeric Control"=12369084, "Numeric Control"=12369084}, {"Numeric Control"=6603023, "Numeric Control"=6603023}, {"Numeric Control"=1976113, "Numeric Control"=1976113}, {"Numeric Control"=2575993, "Numeric Control"=2575993}] ("Colors [4] 2"), "Value"=FALSE) -> ()  [unwired: 2 in, 2 out]
                          }
                          frame 9 {
                            n1039 = property on="Zone 09" class="Bool (strict)"("Colors [4]"=T11 [{"Numeric Control"=12369084, "Numeric Control"=12369084}, {"Numeric Control"=6603023, "Numeric Control"=6603023}, {"Numeric Control"=1976113, "Numeric Control"=1976113}, {"Numeric Control"=2575993, "Numeric Control"=2575993}] ("Colors [4] 2"), "Value"=FALSE) -> ()  [unwired: 2 in, 2 out]
                          }
                          frame 10 {
                            n1040 = property on="Zone 10" class="Bool (strict)"("Colors [4]"=T11 [{"Numeric Control"=12369084, "Numeric Control"=12369084}, {"Numeric Control"=6603023, "Numeric Control"=6603023}, {"Numeric Control"=1976113, "Numeric Control"=1976113}, {"Numeric Control"=2575993, "Numeric Control"=2575993}] ("Colors [4] 2"), "Value"=FALSE) -> ()  [unwired: 2 in, 2 out]
                          }
                          frame 11 {
                            n1041 = property on="Zone 11" class="Bool (strict)"("Colors [4]"=T11 [{"Numeric Control"=12369084, "Numeric Control"=12369084}, {"Numeric Control"=6603023, "Numeric Control"=6603023}, {"Numeric Control"=1976113, "Numeric Control"=1976113}, {"Numeric Control"=2575993, "Numeric Control"=2575993}] ("Colors [4] 2"), "Value"=FALSE) -> ()  [unwired: 2 in, 2 out]
                          }
                          frame 12 {
                            n1042 = property on="Zone 12" class="Bool (strict)"("Colors [4]"=T11 [{"Numeric Control"=12369084, "Numeric Control"=12369084}, {"Numeric Control"=6603023, "Numeric Control"=6603023}, {"Numeric Control"=1976113, "Numeric Control"=1976113}, {"Numeric Control"=2575993, "Numeric Control"=2575993}] ("Colors [4] 2"), "Value"=FALSE) -> ()  [unwired: 2 in, 2 out]
                          }
                          frame 13 {
                            n1043 = property on="Zone 13" class="Bool (strict)"("Colors [4]"=T11 [{"Numeric Control"=12369084, "Numeric Control"=12369084}, {"Numeric Control"=6603023, "Numeric Control"=6603023}, {"Numeric Control"=1976113, "Numeric Control"=1976113}, {"Numeric Control"=2575993, "Numeric Control"=2575993}] ("Colors [4] 2"), "Value"=FALSE) -> ()  [unwired: 2 in, 2 out]
                          }
                        }
                      }
                      frame Enabled {
                      }
                    }
                    n1044 = Index Array(array=w1695, index=0) -> (element=w1693:cluster{"String":string, "Value":i32})
                    n1045 = Unbundle By Name(w1693) -> ("Value"=w1692:i32)
                    n1046 = for {
                      N: 14 -> [_]
                      tunnel: [w1750] -> w1718 mode=indexing
                      tunnel: [w1747] -> w1714
                      tunnel: w1713 -> [w1747]
                      tunnel: w1692 -> [w1748]
                      i -> [w1746]
                      n1047 = Greater Than 0?(x=w1746) -> (x > 0?=w1745:bool)
                      n1048 = case shown="True" w1745 {
                        tunnel: w1746 -> [_ w1754]
                        frame False {
                        }
                        frame True {
                          w1757 = refnum<vi> refnum  # Boolean
                          n1049 = Decrement(x=w1754) -> (x-1=w1753:i32)
                          n1050 = property on="Zone-based stimulus setup" class="RadioBtnsControl (strict)"() -> ("Controls[]"=w1755:refnum<vi>[])  [unwired: 2 in, 2 out]
                          n1051 = Index Array(array=w1755, index=w1753) -> (element=w1756:refnum<vi>)
                          n1052 = To More Specific Class(target class=w1757, reference=w1756) -> (specific class reference=w1758:refnum<vi>)  [unwired: 1 in, 1 out]
                          n1053 = property class="Bool"(reference=w1758, "Colors [4]"=T11 [{"Numeric Control"=12369084, "Numeric Control"=12369084}, {"Numeric Control"=6603023, "Numeric Control"=6603023}, {"Numeric Control"=1976113, "Numeric Control"=1976113}, {"Numeric Control"=2575993, "Numeric Control"=2575993}] ("Colors [4] 2"), "Value"=FALSE) -> ()  [unwired: 1 in, 2 out]
                        }
                      }
                      n1054 = Bundle By Name(cluster=T47 {"Event type"=0, "Cond., s"=0.0, "Stim., s"=0.0, "Set/Clear"=FALSE, "TTL out N"=1, "Stim. has been set"=FALSE} ("Cluster of the stimuls settings"), "TTL out N"=w1748) -> (w1750:T47)
                    }
                    n1055 = global write "SW_Globals.vi" "Zone-based stimulus presets"(w1718) -> ()
                    n1056 = property on="Stimulus presets" class="Arr (strict)"("Value"=w1718) -> (error out=w1715:errorcluster)  [unwired: 2 in, 1 out]
                    n1057 = property on="Reset STIM" class="Bool (strict)"(error in=w1715, "Val(Sgnl)"=w1714) -> ()  [unwired: 1 in, 2 out]
                  }
                }
              }
              event "Reset regions": Value Change {
                n1058 = event-data() -> ("OldVal"=w1759:bool, "NewVal"=w1760:bool)  [unwired: 1 in, 4 out]
                n1059 = property on="Reset regions" class="Bool (strict)"("Value"=w1759) -> ()  [unwired: 2 in, 2 out]
                n1060 = case shown="True" w1760 {
                  selector: w1760 -> [_ w1762]
                  frame False {
                  }
                  frame True {
                    n1061 = local read "Cage diameter, mm"() -> (w1763:u16)
                    n1062 = case shown="240" w1763 {
                      tunnel: w1762 -> [w1764 w1771 w1778 w1785 w1792 w1799]
                      tunnel: [w1764 w1771 w1778 w1785 w1792 w1799] -> w1761
                      frame 180, Default {
                        n1063 = local write "N segments BORDER"(u8 4 ("N segments")) -> ()
                        n1064 = local write "N segments MIDFIELD"(u8 2 ("N segments")) -> ()
                        n1065 = local write "Starting angle BORDER"(i16 0 ("Starting angle")) -> ()
                        n1066 = local write "Starting angle MIDFIELD"(i16 0 ("Starting angle")) -> ()
                        n1067 = local write "Radius, mm CENTER"(u16 30 ("Radius, mm")) -> ()
                        n1068 = local write "Radius, mm MIDFIELD"(u16 75 ("Radius, mm")) -> ()
                      }
                      frame 240 {
                        n1069 = local write "N segments BORDER"(u8 4 ("N segments")) -> ()
                        n1070 = local write "N segments MIDFIELD"(u8 2 ("N segments")) -> ()
                        n1071 = local write "Starting angle BORDER"(i16 0 ("Starting angle")) -> ()
                        n1072 = local write "Starting angle MIDFIELD"(i16 0 ("Starting angle")) -> ()
                        n1073 = local write "Radius, mm CENTER"(u16 32 ("Radius, mm")) -> ()
                        n1074 = local write "Radius, mm MIDFIELD"(u16 75 ("Radius, mm")) -> ()
                      }
                      frame 290 {
                        n1075 = local write "N segments BORDER"(u8 4 ("N segments")) -> ()
                        n1076 = local write "N segments MIDFIELD"(u8 2 ("N segments")) -> ()
                        n1077 = local write "Starting angle BORDER"(i16 0 ("Starting angle")) -> ()
                        n1078 = local write "Starting angle MIDFIELD"(i16 0 ("Starting angle")) -> ()
                        n1079 = local write "Radius, mm CENTER"(u16 48 ("Radius, mm")) -> ()
                        n1080 = local write "Radius, mm MIDFIELD"(u16 121 ("Radius, mm")) -> ()
                      }
                      frame 325 {
                        n1081 = local write "N segments BORDER"(u8 4 ("N segments")) -> ()
                        n1082 = local write "N segments MIDFIELD"(u8 2 ("N segments")) -> ()
                        n1083 = local write "Starting angle BORDER"(i16 0 ("Starting angle")) -> ()
                        n1084 = local write "Starting angle MIDFIELD"(i16 0 ("Starting angle")) -> ()
                        n1085 = local write "Radius, mm CENTER"(u16 50 ("Radius, mm")) -> ()
                        n1086 = local write "Radius, mm MIDFIELD"(u16 148 ("Radius, mm")) -> ()
                      }
                      frame 327 {
                        n1087 = local write "N segments BORDER"(u8 4 ("N segments")) -> ()
                        n1088 = local write "N segments MIDFIELD"(u8 2 ("N segments")) -> ()
                        n1089 = local write "Starting angle BORDER"(i16 0 ("Starting angle")) -> ()
                        n1090 = local write "Starting angle MIDFIELD"(i16 0 ("Starting angle")) -> ()
                        n1091 = local write "Radius, mm CENTER"(u16 50 ("Radius, mm")) -> ()
                        n1092 = local write "Radius, mm MIDFIELD"(u16 150 ("Radius, mm")) -> ()
                      }
                      frame 333 {
                        n1093 = local write "N segments BORDER"(u8 4 ("N segments")) -> ()
                        n1094 = local write "N segments MIDFIELD"(u8 2 ("N segments")) -> ()
                        n1095 = local write "Starting angle BORDER"(i16 0 ("Starting angle")) -> ()
                        n1096 = local write "Starting angle MIDFIELD"(i16 0 ("Starting angle")) -> ()
                        n1097 = local write "Radius, mm CENTER"(u16 50 ("Radius, mm")) -> ()
                        n1098 = local write "Radius, mm MIDFIELD"(u16 152 ("Radius, mm")) -> ()
                      }
                    }
                    n1099 = property on="Reset REG" class="Bool (strict)"("Val(Sgnl)"=w1761) -> ()  [unwired: 2 in, 2 out]
                  }
                }
              }
              event "Set advanced stimulus": Value Change {
                n1100 = event-data() -> ("OldVal"=w1807:bool)  [unwired: 1 in, 5 out]
                n1101 = property on="Set advanced stimulus" class="Bool (strict)"("Value"=w1807) -> (error out=w1809:errorcluster)  [unwired: 2 in, 1 out]
                n1102 = property on="Adv. Stim. set" class="Bool (strict)"(error in=w1809, "Value"=w1807) -> (error out=w1808:errorcluster)  [unwired: 1 in, 1 out]
                n1103 = flat-sequence {
                  tunnel: w1808 -> [_]
                  tunnel: [w1810] -> w1806
                  tunnel: w1806 -> [w1825]
                  frame #0 {
                    n1104 = property on="Stimulus presets" class="Arr (strict)"() -> ("Value"=w1811:T7)  [unwired: 2 in, 2 out]
                    n1105 = local read "N segments MIDFIELD"() -> (w1822:u8)
                    n1106 = local read "N segments BORDER"() -> (w1823:u8)
                    n1107 = global read "SW_Globals.vi" "Speed detection threshold, mm/s"() -> (w1816:dbl)
                    n1108 = global read "SW_Globals.vi" "Run time threshold, s"() -> (w1817:dbl)
                    n1109 = global read "SW_Globals.vi" "Run time pause, s"() -> (w1818:dbl)
                    n1110 = Compound Arithmetic op=ADD(w1823, w1822, u8 1 ("value")) -> (w1820:u8)
                    n1111 = global read "SW_Globals.vi" "Run time stim, s"() -> (w1819:dbl)
                    n1112 = call "SW_Set_Adv_Stimulus_interface.vi"("Zone-based stimulus presents"=w1811, "Total amount of segments"=w1820, "Run time stim, s"=w1819, "Run time pause, s"=w1818, "Run time threshold, s"=w1817, "Speed detection threshold, mm/s"=w1816) -> ("Modified Zone-based stimulus presents"=w1810:T7, "Out Run time stim, s"=w1815:dbl, "Out Run time pause, s"=w1814:dbl, "Out Run time threshold, s"=w1813:dbl, "Out Speed detection threshold, mm/s"=w1812:dbl)  [unwired: 4 in, 1 out]
                    n1113 = property on="Stimulus presets" class="Arr (strict)"("Value"=w1810) -> ()  [unwired: 2 in, 2 out]
                    n1114 = global write "SW_Globals.vi" "Speed detection threshold, mm/s"(w1812) -> ()
                    n1115 = global write "SW_Globals.vi" "Run time stim, s"(w1815) -> ()
                    n1116 = global write "SW_Globals.vi" "Run time pause, s"(w1814) -> ()
                    n1117 = global write "SW_Globals.vi" "Run time threshold, s"(w1813) -> ()
                  }
                  frame #1 {
                    n1118 = for {
                      tunnel: [w1830] -> w1824 mode=indexing if=w1828
                      tunnel: w1825 -> [w1829] mode=indexing
                      i -> [w1827]
                      n1119 = Unbundle By Name(w1829) -> ("Stim. has been set"=w1828:bool)
                      n1120 = Greater Than 0?(x=w1827) -> (x > 0?=w1826:bool)
                      n1121 = case shown="True" w1826 {
                        tunnel: w1828 -> [_ w1841]
                        tunnel: w1827 -> [_ w1832]
                        frame False {
                        }
                        frame True {
                          w1836 = refnum<vi> refnum  # Boolean
                          n1122 = Decrement(x=w1832) -> (x-1=w1831:i32)
                          n1123 = property on="Colors for Stim. setup" class="Arr (strict)"() -> ("Value"=w1840:T3)  [unwired: 2 in, 2 out]
                          n1124 = Select(t=w1840, s=w1841, f=T11 [{"Numeric Control"=12369084, "Numeric Control"=12369084}, {"Numeric Control"=6603023, "Numeric Control"=6603023}, {"Numeric Control"=1976113, "Numeric Control"=1976113}, {"Numeric Control"=2575993, "Numeric Control"=2575993}] ("Colors [4] 2")) -> (s? t:f=w1834:T11)
                          n1125 = property on="Zone-based stimulus setup" class="RadioBtnsControl (strict)"() -> ("Controls[]"=w1838:refnum<vi>[])  [unwired: 2 in, 2 out]
                          n1126 = Index Array(array=w1838, index=w1831) -> (element=w1837:refnum<vi>)
                          n1127 = To More Specific Class(target class=w1836, reference=w1837) -> (specific class reference=w1835:refnum<vi>)  [unwired: 1 in, 1 out]
                          n1128 = property class="Bool"(reference=w1835, "Colors [4]"=w1834, "Value"=FALSE) -> ()  [unwired: 1 in, 2 out]
                        }
                      }
                      n1129 = To Unsigned Byte Integer(number=w1827) -> (unsigned 8bit integer=w1830:u8)
                    }
                    n1130 = global write "SW_Globals.vi" "Regions to track"(w1824) -> ()
                  }
                  frame #2 {
                    n1131 = property on="Adv. Stim. set" class="Bool (strict)"("Val(Sgnl)"=TRUE ("Value (Signaling)")) -> ()  [unwired: 2 in, 2 out]
                  }
                }
              }
              event "Load settings": Value Change {
                (unwired) "*.trset; *.tdms" ("default name")
                w1856 = T53 2 items=["User Home"=0, "User Desktop"=1, "User Documents"=2, "User Application Data"=3, "User Preferences"=4, "User Temporary"=5, "Public Documents"=6, "Public Application Data"=7, "Public Preferences"=8, "Public Cache"=13, "System Core Libraries"=9, "System Installed Libraries"=10, "Application Files"=11, "Boot Volume Root"=12] ("system directory type")
                n1132 = event-data() -> ("OldVal"=w1861:bool)  [unwired: 1 in, 5 out]
                n1133 = property on="Load settings" class="Bool (strict)"("Value"=w1861) -> ()  [unwired: 2 in, 2 out]
                n1134 = call <vilib>:"Get System Directory.vi"("system directory type"=w1856) -> ("system directory"=w1852:path)  [unwired: 10 in]
                n1135 = Build Path(base path=w1852, name or relative path="MHC_Tracker" ("string")) -> (appended path=w1853:path)
                n1136 = call <vilib>:"Check if File or Folder Exists.vi"("path"=w1853) -> ("file or folder exists?"=w1854:bool)  [unwired: 8 in, 2 out]
                n1137 = Select(t=w1853, s=w1854, f=w1852) -> (s? t:f=w1851:path)
                n1138 = call "Load Settings"("start path"=w1851, "prompt"="Please choose file to load settings from", "button label"="Load", "pattern (all files)"="*.trset; *.tdms" ("default name"), "pattern label"="Settings or track") -> ("selected path"=w1846:path, "exists"=w1848:bool, "cancelled"=w1849:bool, "error out"=w1845:errorcluster)  [unwired: 7 in]
                n1139 = Not(x=w1849) -> (.not. x?=w1850:bool)
                n1140 = And(x=w1848, y=w1850) -> (x .and. y?=w1847:bool)
                n1141 = case shown="True" w1847 {
                  tunnel: w1846 -> [_ w1886]
                  tunnel: w1845 -> [w1862 w1887]
                  tunnel: [w1862 w1865] -> w1844
                  tunnel: [FALSE ("IO paramaters loaded") TRUE ("IO paramaters loaded")] -> w1843
                  frame False {
                  }
                  frame True {
                    n1142 = local read "Current User"() -> (w1888:string)
                    n1143 = call "SW_Load_settings_from_previous_experiments.vi"("File to load data from"=w1886, "User Name"=w1888, "error in (no error)"=w1887) -> ("Settings cluster out"=w1885:T35, "IO parameters cluster"=→"IO parameters loaded cluster":T2, "Stimulus presets array"=w1867:T36, "error out"=w1865:errorcluster)  [unwired: 4 in]
                    n1144 = Unbundle By Name(w1885) -> ("Name prefix"=w1884:string, "N segments MIDFIELD"=w1871:u8, "N segments BORDER"=w1883:u8, "Radius, mm CENTER"=w1882:u16, "Radius, mm MIDFIELD"=w1881:u16, "Starting angle MIDFIELD"=w1880:i16, "Starting angle BORDER"=w1879:i16, "Cage diameter, mm"=w1878:u16, "Bridge swap"=w1877:bool, "Bridge V. offset"=w1876:sgl, "Twisted neck"=w1874:bool, "Offset H."=w1875:sgl, "\"Stop at\" enabled"=w1873:bool, "Stop at"=w1872:dbl, "Data filtering"=w1866:u16)
                    n1145 = property on="Bridge swap" class="Bool (strict)"("Value"=w1877) -> ()  [unwired: 2 in, 2 out]
                    n1146 = local write "Twisted neck"(w1874) -> ()
                    n1147 = local write "Data filtering"(w1866) -> ()
                    n1148 = local write "Bridge offset"(w1876) -> ()
                    n1149 = local write "Radius, mm CENTER"(w1882) -> ()
                    n1150 = local write "Radius, mm MIDFIELD"(w1881) -> ()
                    n1151 = local write "Cage diameter, mm"(w1878) -> ()
                    n1152 = local write "\"Stop at\" enabled"(w1873) -> ()
                    n1153 = local write "Stop record at"(w1872) -> ()
                    n1154 = local write "N segments BORDER"(w1883) -> ()
                    n1155 = local write "Name Prefix"(w1884) -> ()
                    n1156 = local write "Starting angle MIDFIELD"(w1880) -> ()
                    n1157 = local write "Starting angle BORDER"(w1879) -> ()
                    n1158 = local write "Bridge horizontal offset"(w1875) -> ()
                    n1159 = property on="N segments MIDFIELD" class="DigNum (strict)"("Val(Sgnl)"=w1871) -> (error out=w1869:errorcluster)  [unwired: 2 in, 1 out]
                    n1160 = property on="Stimulus presets" class="Arr (strict)"(error in=w1869, "Value"=w1867) -> ()  [unwired: 1 in, 2 out]
                    n1161 = for {
                      tunnel: [w1893] -> w1868 mode=indexing if=w1891
                      tunnel: w1867 -> [w1892] mode=indexing
                      i -> [w1890]
                      n1162 = Unbundle By Name(w1892) -> ("Stim. has been set"=w1891:bool)
                      n1163 = Greater Than 0?(x=w1890) -> (x > 0?=w1889:bool)
                      n1164 = case shown="True" w1889 {
                        tunnel: w1891 -> [_ w1904]
                        tunnel: w1890 -> [_ w1895]
                        frame False {
                        }
                        frame True {
                          w1899 = refnum<vi> refnum  # Boolean
                          n1165 = Decrement(x=w1895) -> (x-1=w1894:i32)
                          n1166 = property on="Colors for Stim. setup" class="Arr (strict)"() -> ("Value"=w1903:T3)  [unwired: 2 in, 2 out]
                          n1167 = Select(t=w1903, s=w1904, f=T11 [{"Numeric Control"=12369084, "Numeric Control"=12369084}, {"Numeric Control"=6603023, "Numeric Control"=6603023}, {"Numeric Control"=1976113, "Numeric Control"=1976113}, {"Numeric Control"=2575993, "Numeric Control"=2575993}] ("Colors [4] 2")) -> (s? t:f=w1897:T11)
                          n1168 = property on="Zone-based stimulus setup" class="RadioBtnsControl (strict)"() -> ("Controls[]"=w1901:refnum<vi>[])  [unwired: 2 in, 2 out]
                          n1169 = Index Array(array=w1901, index=w1894) -> (element=w1900:refnum<vi>)
                          n1170 = To More Specific Class(target class=w1899, reference=w1900) -> (specific class reference=w1898:refnum<vi>)  [unwired: 1 in, 1 out]
                          n1171 = property class="Bool"(reference=w1898, "Colors [4]"=w1897, "Value"=FALSE) -> ()  [unwired: 1 in, 2 out]
                        }
                      }
                      n1172 = To Unsigned Byte Integer(number=w1890) -> (unsigned 8bit integer=w1893:u8)
                    }
                    n1173 = global write "SW_Globals.vi" "Regions to track"(w1868) -> ()
                    "Settings load path" <- w1886
                  }
                }
                n1174 = property on="IO paramaters loaded from file" class="Bool (strict)"(error in=w1844, "Value"=w1843) -> ()  [unwired: 1 in, 2 out]
              }
            }
            "Adv. Stim. set" <- FALSE ("Adv. Stim. set")
          }
          frame #2 {
            # "Segments scheme can be reset here"
            n1175 = First Call?() -> (First Call?: T/F=w1907:bool)
            n1176 = case shown="True" w1907 {
              selector: w1907 -> [_ w1910]
              tunnel: [_ w1909] -> w1908
              frame False {
              }
              frame True {
                n1177 = property on="Init plot" class="Bool (strict)"("Val(Sgnl)"=w1910) -> (error out=w1909:errorcluster)  [unwired: 2 in, 1 out]
              }
            }
            n1178 = event shown="[0] \"Init plot\", \"Zone-based stimulus setup\", \"N segments MIDFIELD\", \"N segments BORDER\", \"Starting angle MIDFIELD\", \"Starting angle BORDER\", \"Radius, mm MIDFIELD\", \"Radius, mm CENTER\", \"Cage diameter, mm\", \"Reset stimuli\", \"Reset regions\", \"Reset REG\", \"Reset STIM\", \"Adv. Stim. set\": Value Change" {
              selector: _ -> [_ _]
              dyn-events: _ -> [_ _]
              timeout: 1 -> [_ _]
              tunnel: w1908 -> [_ _]
              event "Init plot", "Zone-based stimulus setup", "N segments MIDFIELD", "N segments BORDER", "Starting angle MIDFIELD", "Starting angle BORDER", "Radius, mm MIDFIELD", "Radius, mm CENTER", "Cage diameter, mm", "Reset stimuli", "Reset regions", "Reset REG", "Reset STIM", "Adv. Stim. set": Value Change {
                n1179 = event-data() -> ()  [unwired: 1 in, 6 out]
                n1180 = local read "Cage diameter, mm"() -> (w1911:u16)
                n1181 = case "Let's set flag for alternative magnets orintation" shown="333" w1911 {
                  frame 180, Default {
                    n1182 = global write "SW_Globals.vi" "Alternative magnets orientation"(FALSE ("Alternative magnets orientation")) -> ()
                  }
                  frame 240 {
                    n1183 = global write "SW_Globals.vi" "Alternative magnets orientation"(FALSE ("Alternative magnets orientation")) -> ()
                  }
                  frame 290 {
                    n1184 = global write "SW_Globals.vi" "Alternative magnets orientation"(FALSE ("Alternative magnets orientation")) -> ()
                  }
                  frame 325 {
                    n1185 = global write "SW_Globals.vi" "Alternative magnets orientation"(FALSE ("Alternative magnets orientation")) -> ()
                  }
                  frame 327 {
                    n1186 = global write "SW_Globals.vi" "Alternative magnets orientation"(TRUE ("Alternative magnets orientation")) -> ()
                  }
                  frame 333 {
                    n1187 = global write "SW_Globals.vi" "Alternative magnets orientation"(FALSE ("Alternative magnets orientation")) -> ()
                  }
                }
                n1188 = global read "SW_Globals.vi" "Regions to track"() -> (w1933:u8[])
                n1189 = To Unsigned Byte Integer(number="Zone-based stimulus setup") -> (unsigned 8bit integer=w1934:u8)
                n1190 = Bundle("N segments BORDER"="N segments BORDER", "Starting angle BORDER"="Starting angle BORDER", "N segments MIDFIELD"="N segments MIDFIELD", "Starting angle MIDFIELD"="Starting angle MIDFIELD", "Radius, mm MIDFIELD"="Radius, mm MIDFIELD", u8 1, "Radius, mm CENTER"="Radius, mm CENTER", "Cage diameter, mm"=w1911, 10) -> (w1921:T54)  [unwired: 1 in]
                n1191 = property on="Segments diagram" class="Pict"() -> ("Bounds"=w1931:T19)  [unwired: 2 in, 2 out]
                n1192 = Build Array(w1934) -> (w1930:u8[])
                n1193 = Build Array (concatenate)(w1930, w1933) -> (w1932:u8[])
                n1194 = call "SW_Gen_Check_segments_parameters.vi"("Image plotting parameters"=w1921) -> ("Corrected image plotting parameters"=w1920:T55)  [unwired: 2 in]
                n1195 = Unbundle By Name(w1920) -> ("N segments BORDER"=w1919:u8, "N segments MIDFIELD"=w1917:u8, "Radius, mm MIDFIELD"=w1916:u16, "Radius, mm CENTER"=w1918:u16)
                n1196 = call "SW_Generate_Segmented_Plot_v3.vi"("Draw Area Size"=w1931, "Regions to mark set"=w1932, "Regions to mark selected"=w1930, "Input cluster of parameters"=w1920) -> ("Zones layout output"=w1913:picture, "No zones image"=w1912:picture, "Array of the pixel to color correspondences"=w1914:u32[][], "Array of the segment to color correspondences"=w1915:u32[][])  [unwired: 6 in, 2 out]
                "Segments diagram" <- w1913
                n1197 = property on="N segments BORDER" class="DigNum (strict)"("Value"=w1919) -> ()  [unwired: 2 in, 2 out]
                n1198 = property on="N segments MIDFIELD" class="DigNum (strict)"("Value"=w1917) -> ()  [unwired: 2 in, 2 out]
                n1199 = property on="Radius, mm MIDFIELD" class="DigNum (strict)"("Value"=w1916) -> ()  [unwired: 2 in, 2 out]
                n1200 = property on="Radius, mm CENTER" class="DigNum (strict)"("Value"=w1918) -> ()  [unwired: 2 in, 2 out]
                n1201 = global write "SW_Globals.vi" "Diagram"(w1913) -> ()
                n1202 = global write "SW_Globals.vi" "Full track with zones"(w1913) -> ()
                n1203 = global write "SW_Globals.vi" "Diagram no zones"(w1912) -> ()
                n1204 = global write "SW_Globals.vi" "Full track with no zones"(w1912) -> ()
                n1205 = global write "SW_Globals.vi" "Array of the pixel to color correspondences"(w1914) -> ()
                n1206 = global write "SW_Globals.vi" "Array of the segment to color correspondences"(w1915) -> ()
              }
              event Timeout {
                n1207 = event-data() -> ()  [unwired: 1 in, 3 out]
              }
            }
          }
          frame #3 {
            # "Save settings and set important variables before actual start of the recording. Also initial \"Play\" command is sent from here."
            n1208 = Build Array("Start Tracking button", "Jump to Analysis") -> (w1945:bool[])
            n1209 = Boolean Array To Number(Boolean array=w1945) -> (number=w1943:u32)
            n1210 = case shown="1" w1943 {
              tunnel: w1947 -> [_ w2015 w2145]
              tunnel: w1942 -> [_ w1963 _]
              frame 0, Default {
              }
              frame 1 {
                w1964 = T56 {"Zone[1]"=FALSE, "Zone[2]"=FALSE, "Zone[3]"=FALSE, "Zone[4]"=FALSE, "Zone[5]"=FALSE, "Zone[6]"=FALSE, "Zone[7]"=FALSE, "Zone[8]"=FALSE, "Zone[9]"=FALSE, "Zone[10]"=FALSE, "Zone[11]"=FALSE, "Zone[12]"=FALSE, "Zone[13]"=FALSE} ("Zones presence indicator")
                w2049 = enum32{"Settings", "Recording", "Analysis"}."Recording" ("Main tab control")
                w2053 = enum32{"Settings", "Recording", "Analysis"}."Analysis" ("Main tab control")
                w2062 = enum32{"Settings", "Recording", "Analysis"}."Settings" ("Main tab control")
                n1211 = flat-sequence {
                  tunnel: w2015 -> [w2109]
                  tunnel: w1963 -> [w2103]
                  tunnel: [w2109] -> w2014
                  tunnel: w2014 -> [w2111]
                  tunnel: [w2111] -> w1969
                  tunnel: [w2114] -> w1956
                  tunnel: w1969 -> [w2121]
                  frame #0 {
                    n1212 = Unbundle By Name(w2103) -> ("Play/Pause status"=w2107:refnum<notifier>, "Recording now"=w2102:refnum<notifier>, "(Final) Data file is saved"=w2099:refnum<notifier>, "Data loaded"=w2097:refnum<notifier>, "Temp file ready for processing"=w2096:refnum<notifier>, "Has been recorded"=w2093:refnum<notifier>)  [unwired: 1 out]
                    n1213 = Send Notification(notification=FALSE, notifier=w2102) -> ()  [unwired: 1 in, 2 out]
                    n1214 = Send Notification(notification=FALSE, notifier=w2099) -> ()  [unwired: 1 in, 2 out]
                    n1215 = Send Notification(notification=FALSE, notifier=w2097) -> ()  [unwired: 1 in, 2 out]
                    n1216 = Send Notification(notification=FALSE, notifier=w2096) -> ()  [unwired: 1 in, 2 out]
                    n1217 = Send Notification(notification=FALSE, notifier=w2093) -> ()  [unwired: 1 in, 2 out]
                    n1218 = Select(t="Play", s=TRUE, f="Pause") -> (s? t:f=w2106:string)
                    n1219 = Send Notification(notification=w2106, notifier=w2107) -> ()  [unwired: 1 in, 2 out]
                  }
                  frame #1 {
                    n1220 = Wait (ms)(milliseconds to wait=u32 1500) -> ()  [unwired: 1 out]
                  }
                  frame #2 {
                    n1221 = global write "SW_Globals.vi" "Incrementally save First Call"(TRUE ("Incrementally save First Call")) -> ()
                    n1222 = property on="Jump to Analysis" class="Bool (strict)"(error in=w2121, "Value"=FALSE ("Jump to Analysis")) -> (error out=w2119:errorcluster)  [unwired: 1 in, 1 out]
                    n1223 = global read "SW_Globals.vi" "Zones allocation array"() -> (w2123:i32[])
                    n1224 = property on="Record start First Call" class="Bool (strict)"(error in=w2119, "Value"=TRUE ("Record start First Call")) -> (error out=w2117:errorcluster)  [unwired: 1 in, 1 out]
                    n1225 = Array Size(array=w2123) -> (size(s)=w2122:i32)
                    n1226 = Initialize Array(0 ("element"), w2122) -> (w2125:i32[])
                    n1227 = property on="Temp file ready" class="Bool (strict)"(error in=w2117, "Value"=FALSE ("Temp file ready")) -> (error out=w2115:errorcluster)  [unwired: 1 in, 1 out]
                    n1228 = global write "SW_Globals.vi" "Zones allocation array"(w2125) -> ()
                    n1229 = property on="Save files First Call" class="Bool (strict)"(error in=w2115, "Value"=TRUE ("Save files First Call")) -> (error out=w2114:errorcluster)  [unwired: 1 in, 1 out]
                  }
                }
                n1230 = property on="Additional record settings" class="Bool (strict)"(error in=w1956, "DisabledEnum"=T12."Enabled" ("Disabled"), "BoolText.Text"="Set" ("Boolean Text.Text")) -> (error out=w1955:errorcluster)  [unwired: 1 in, 1 out]
                n1231 = property on="Pane" class="Pane"(error in=w1955) -> (error out=w1993:errorcluster, "Decos[]"=w1994:refnum<vi>[])  [unwired: 1 in, 1 out]
                n1232 = Index Array(array=w1994, index=2) -> (element=w1999:refnum<vi>)
                n1233 = property class="Decor"(reference=w1999, error in=w1993, "Visible"=FALSE) -> (error out=w1992:errorcluster)  [unwired: 1 out]
                n1234 = Index Array(array=w1994, index=1) -> (element=w1996:refnum<vi>)
                n1235 = property class="Decor"(reference=w1996, error in=w1992, "Visible"=TRUE) -> (error out=w1991:errorcluster)  [unwired: 1 out]
                n1236 = property on="Main tab control" class="TabCtl (strict)"(error in=w1991, "Value"=w2062) -> (error out=w2058:errorcluster, "Pages"=w2063:refnum<vi>[])  [unwired: 1 in, 1 out]
                n1237 = To Long Integer(number=w2062) -> (32bit integer=w2061:i32)
                n1238 = Index Array(array=w2063, index=w2061) -> (element=w2060:refnum<vi>)
                n1239 = property class="Page"(reference=w2060, error in=w2058, "PageEnb"=T32."Page Disabled & Grayed" ("Page Enabled State")) -> (error out=w2051:errorcluster)  [unwired: 1 out]
                n1240 = property on="Main tab control" class="TabCtl (strict)"(error in=w2051, "Value"=w2053) -> (error out=w2057:errorcluster, "Pages"=w2052:refnum<vi>[])  [unwired: 1 in, 1 out]
                n1241 = To Long Integer(number=w2053) -> (32bit integer=w2054:i32)
                n1242 = Index Array(array=w2052, index=w2054) -> (element=w2055:refnum<vi>)
                n1243 = property class="Page"(reference=w2055, error in=w2057, "PageEnb"=T32."Page Disabled & Grayed" ("Page Enabled State")) -> (error out=w2044:errorcluster)  [unwired: 1 out]
                n1244 = property on="Main tab control" class="TabCtl (strict)"(error in=w2044, "Value"=w2049) -> (error out=w2045:errorcluster, "Pages"=w2050:refnum<vi>[])  [unwired: 1 in, 1 out]
                n1245 = To Long Integer(number=w2049) -> (32bit integer=w2048:i32)
                n1246 = local read "Settings file refnum out"() -> (w2043:T5)
                n1247 = local read "N segments MIDFIELD"() -> (w2041:u8)
                n1248 = Index Array(array=w2050, index=w2048) -> (element=w2047:refnum<vi>)
                n1249 = local read "Current User"() -> (w1971:string)
                n1250 = local read "N segments BORDER"() -> (w2036:u8)
                n1251 = property class="Page"(reference=w2047, error in=w2045, "PageEnb"=T32."Page Enabled" ("Page Enabled State")) -> (error out=w2040:errorcluster)  [unwired: 1 out]
                n1252 = local read "Radius, mm CENTER"() -> (w2035:u16)
                n1253 = call <vilib>:"Write Key (I32).vi"("section"=w1971, "error in (no error)"=w2040, "value"=w2041, "key"="Amount of midfield segments", "refnum"=w2043) -> ("error out"=w2038:errorcluster, "refnum out"=w2037:T5)  [unwired: 4 in, 1 out]
                n1254 = local read "Radius, mm MIDFIELD"() -> (w2028:u16)
                n1255 = call <vilib>:"Write Key (I32).vi"("section"=w1971, "error in (no error)"=w2038, "value"=w2036, "key"="Amount of border segments", "refnum"=w2037) -> ("error out"=w2032:errorcluster, "refnum out"=w2033:T5)  [unwired: 4 in, 1 out]
                n1256 = local read "Starting angle MIDFIELD"() -> (w2027:i16)
                n1257 = call <vilib>:"Write Key (I32).vi"("section"=w1971, "error in (no error)"=w2032, "value"=w2035, "key"="Center segment outer radius, mm", "refnum"=w2033) -> ("error out"=w2029:errorcluster, "refnum out"=w2030:T5)  [unwired: 4 in, 1 out]
                n1258 = local read "Starting angle BORDER"() -> (w2020:i16)
                n1259 = call <vilib>:"Write Key (I32).vi"("section"=w1971, "error in (no error)"=w2029, "value"=w2028, "key"="Midfield segments outer radius, mm", "refnum"=w2030) -> ("error out"=w2024:errorcluster, "refnum out"=w2025:T5)  [unwired: 4 in, 1 out]
                n1260 = local read "Cage diameter, mm"() -> (w2001:u16)
                n1261 = call <vilib>:"Write Key (I32).vi"("section"=w1971, "error in (no error)"=w2024, "value"=w2027, "key"="Midfield segments starting angle", "refnum"=w2025) -> ("error out"=w2022:errorcluster, "refnum out"=w2021:T5)  [unwired: 4 in, 1 out]
                n1262 = global read "SW_Globals.vi" "Zone-based stimulus presets"() -> (w1962:T51)
                n1263 = call <vilib>:"Write Key (I32).vi"("section"=w1971, "error in (no error)"=w2022, "value"=w2020, "key"="Border segments starting angle", "refnum"=w2021) -> ("error out"=w2019:errorcluster, "refnum out"=w2018:T5)  [unwired: 4 in, 1 out]
                n1264 = call <vilib>:"Write Key (I32).vi"("section"=w1971, "error in (no error)"=w2019, "value"=w2001, "key"="Cage diameter, mm", "refnum"=w2018) -> ("error out"=w1959:errorcluster, "refnum out"=w1968:T5)  [unwired: 4 in, 1 out]
                n1265 = for {
                  tunnel: w1962 -> [w2076] mode=indexing
                  tunnel: w1968 -> [w2069]
                  tunnel: [w2073] -> w1974
                  tunnel: w1971 -> [w2067]
                  i -> [w2072]
                  n1266 = Unbundle By Name(w2076) -> ("Stim. has been set"=w2074:bool)
                  n1267 = Flatten To JSON(anything=w2076) -> (JSON string=w2075:string, 11:w2065:errorcluster)  [unwired: 2 in]
                  n1268 = Format Value(string ("")="Zone " ("string"), format string="%02d", value (0)=w2072) -> (output string=w2066:string)
                  n1269 = call <vilib>:"Remove Key.vi"("section"=w2067, "error in (no error)"=w2065, "key"=w2066, "refnum"=w2069) -> ("error out"=w2064:errorcluster, "refnum out"=w2068:T5)  [unwired: 5 in, 1 out]
                  n1270 = case shown="True" w2074 {
                    tunnel: w2075 -> [_ w2083]
                    tunnel: w2064 -> [_ w2082]
                    tunnel: [w2077 w2081] -> w2073
                    tunnel: w2067 -> [_ w2080]
                    tunnel: w2066 -> [_ w2079]
                    tunnel: w2068 -> [w2077 w2078]
                    frame False {
                    }
                    frame True {
                      n1271 = call <vilib>:"Write Key (String).vi"("section"=w2080, "error in (no error)"=w2082, "value"=w2083, "key"=w2079, "refnum"=w2078) -> ("refnum out"=w2081:T5)  [unwired: 4 in, 2 out]
                    }
                  }
                }
                n1272 = global read "SW_Globals.vi" "IO parameters cluster"() -> (w1961:T2)
                n1273 = local read "N segments MIDFIELD"() -> (w1976:u8)
                n1274 = local read "N segments BORDER"() -> (w1977:u8)
                n1275 = property on="Zones presence indicator" class="Clust"() -> ("Controls[]"=w2013:refnum<vi>[])  [unwired: 2 in, 2 out]
                n1276 = Cluster To Array(cluster=w1961) -> (array=w1953:u16[])
                n1277 = Flatten To JSON(anything=w1953, error in (no error)=w1959) -> (JSON string=w1960:string, 11:w1958:errorcluster)  [unwired: 1 in]
                n1278 = Compound Arithmetic op=ADD(w1977, w1976, u8 1 ("value")) -> (w2010:u8)
                n1279 = Increment(x=w2010) -> (x+1=w2009:u8)
                n1280 = for {
                  tunnel: w2013 -> [w2092] mode=indexing
                  tunnel: w2010 -> [w2086]
                  tunnel: [w2084] -> w1965
                  i -> [w2091]
                  n1281 = Increment(x=w2091) -> (x+1=w2085:i32)
                  n1282 = Less Or Equal?(x=w2085, y=w2086) -> (x <= y?=w2090:bool)
                  n1283 = Select(t=T12."Disabled" ("Disabled"), s=w2090, f=T12."Disabled and Grayed Out" ("Disabled")) -> (s? t:f=w2088:T12)
                  n1284 = property class="Ctl"(reference=w2092, "DisabledEnum"=w2088) -> (error out=w2084:errorcluster)  [unwired: 1 in, 1 out]
                }
                n1285 = call <vilib>:"Write Key (String).vi"("section"=w1971, "error in (no error)"=w1958, "value"=w1960, "key"="IO ports configuration", "refnum"=w1974) -> ("error out"=w1973:errorcluster, "refnum out"=w1972:T5)  [unwired: 4 in, 1 out]
                n1286 = global write "SW_Globals.vi" "Active segments amount"(w2010) -> ()
                n1287 = local read "Starting angle MIDFIELD"() -> (w1981:i16)
                n1288 = local read "Starting angle BORDER"() -> (w1982:i16)
                n1289 = local read "Radius, mm MIDFIELD"() -> (w1980:u16)
                n1290 = local read "Radius, mm CENTER"() -> (w1978:u16)
                n1291 = local read "Cage diameter, mm"() -> (w1975:u16)
                n1292 = call <vilib>:"Close Config Data.vi"("error in (no error)"=w1973, "refnum"=w1972) -> ("error out"=w2016:errorcluster)  [unwired: 8 in, 1 out]
                n1293 = Bundle By Name(cluster=T21 {"Minimum"=0.0, "Maximum"=14.0, "Increment"=1.0, "Minor Increment"=1.0, "Start"=0.0} ("X Scale.Range"), "Maximum"=w2009) -> (w1952:T21)
                n1294 = property on="Diagram at recording" class="Pict"(error in=w2016) -> ("Bounds"=w1990:T19)  [unwired: 1 in, 2 out]
                n1295 = property on="Histograms (normalized)" class="WFGraph (strict)"("XScale.Range"=w1952, "Caption.Text"="Zone preference (normalized)" ("Label.Text"), "XScale.ScaleFit"=u8 2 ("X Scale.Scale Fit"), "XScale.Ofst&Mult"=T30 {"Offset"=1.0, "Multiplier"=0.0} ("X Scale.Offset and Multiplier"), "YScale.Mapping Mode"=u8 0 ("Y Scale.Mapping Mode")) -> ()  [unwired: 2 in, 2 out]
                n1296 = Bundle By Name(cluster=T20 {"Amount of border segments"=8, "Border segments starting angle"=0, "Amount of midfield segments"=4, "Midfield segments starting angle"=0, "Midfield segments outer radius, mm"=60, "Amount of central segments"=1, "Center segment outer radius, mm"=30, "Diameter of the cage, mm"=180, "R-gap between segments, mm"=10} ("Input cluster of parameters"), "Amount of border segments"=w1977, "Border segments starting angle"=w1982, "Amount of midfield segments"=w1976, "Midfield segments starting angle"=w1981, "Midfield segments outer radius, mm"=w1980, "Amount of central segments"=u8 1, "Center segment outer radius, mm"=w1978, "Diameter of the cage, mm"=w1975) -> (w1983:T20)
                n1297 = global read "SW_Globals.vi" "Regions to track"() -> (w1989:u8[])
                n1298 = call "SW_Generate_Segmented_Plot_v3.vi"("Draw Area Size"=w1990, "Regions to mark set"=w1989, "Input cluster of parameters"=w1983) -> ("Zones layout output"=w1966:picture, "No zones image"=w1967:picture, "Array of the pixel to color correspondences"=w1985:u32[][], "Array of the segment to color correspondences"=w1988:u32[][], "Cluster of image geometrical and scaling parameters"=w1987:T27)  [unwired: 7 in, 1 out]
                n1299 = global write "SW_Globals.vi" "Diagram"(w1966) -> ()
                n1300 = global write "SW_Globals.vi" "Full track with zones"(w1966) -> ()
                n1301 = Unbundle By Name(w1987) -> ("Pixels per mm"=→"Pixels per mm":dbl)
                n1302 = global write "SW_Globals.vi" "Diagram no zones"(w1967) -> ()
                n1303 = global write "SW_Globals.vi" "Full track with no zones"(w1967) -> ()
                n1304 = local write "Diagram at recording"(w1966) -> ()
                n1305 = global write "SW_Globals.vi" "Array of the pixel to color correspondences"(w1985) -> ()
                n1306 = global write "SW_Globals.vi" "Array of the segment to color correspondences"(w1988) -> ()
                n1307 = Array Size(array=w1985) -> (size(s)=w2006:i32[])
                n1308 = Index Array(array=w2006, index=0) -> (element=w2005:i32)
                n1309 = Index Array(array=w2006, index=1) -> (element=w2004:i32)
                n1310 = Initialize Array(u32 0 ("element"), w2005, w2004) -> (w2002:u32[][])
                n1311 = property on="Zones presence indicator" class="Clust"(error in=w1965, "Value"=w1964) -> ()  [unwired: 1 in, 2 out]
                n1312 = global write "SW_Globals.vi" "Zones presence indicator"(w1964) -> ()
                n1313 = global write "SW_Globals.vi" "Array of the presence count"(w2002) -> ()
              }
              frame 2 {
                w2131 = T12."Disabled and Grayed Out" ("Disabled")
                w2132 = FALSE ("Zones an.")
                w2151 = enum32{"Settings", "Recording", "Analysis"}."Analysis" ("Main tab control")
                w2155 = enum32{"Settings", "Recording", "Analysis"}."Recording" ("Main tab control")
                w2164 = enum32{"Settings", "Recording", "Analysis"}."Settings" ("Main tab control")
                n1314 = property on="Main tab control" class="TabCtl (strict)"(error in=w2145, "Value"=w2164) -> (error out=w2160:errorcluster, "Pages"=w2165:refnum<vi>[])  [unwired: 1 in, 1 out]
                n1315 = To Long Integer(number=w2164) -> (32bit integer=w2163:i32)
                n1316 = Index Array(array=w2165, index=w2163) -> (element=w2162:refnum<vi>)
                n1317 = property class="Page"(reference=w2162, error in=w2160, "PageEnb"=T32."Page Disabled & Grayed" ("Page Enabled State")) -> (error out=w2153:errorcluster)  [unwired: 1 out]
                n1318 = property on="Main tab control" class="TabCtl (strict)"(error in=w2153, "Value"=w2155) -> (error out=w2159:errorcluster, "Pages"=w2154:refnum<vi>[])  [unwired: 1 in, 1 out]
                n1319 = To Long Integer(number=w2155) -> (32bit integer=w2156:i32)
                n1320 = Index Array(array=w2154, index=w2156) -> (element=w2157:refnum<vi>)
                n1321 = property class="Page"(reference=w2157, error in=w2159, "PageEnb"=T32."Page Disabled & Grayed" ("Page Enabled State")) -> (error out=w2146:errorcluster)  [unwired: 1 out]
                n1322 = property on="Main tab control" class="TabCtl (strict)"(error in=w2146, "Value"=w2151) -> (error out=w2147:errorcluster, "Pages"=w2152:refnum<vi>[])  [unwired: 1 in, 1 out]
                n1323 = To Long Integer(number=w2151) -> (32bit integer=w2150:i32)
                n1324 = Index Array(array=w2152, index=w2150) -> (element=w2149:refnum<vi>)
                n1325 = property class="Page"(reference=w2149, error in=w2147, "PageEnb"=T32."Page Enabled" ("Page Enabled State")) -> (error out=w2144:errorcluster)  [unwired: 1 out]
                n1326 = property on="Zones (analysis)" class="Bool (strict)"(error in=w2144, "Value"=w2132, "DisabledEnum"=w2131) -> (error out=w2143:errorcluster)  [unwired: 1 in, 1 out]
                n1327 = property on="Show heatmap (analysis)" class="Bool (strict)"("DisabledEnum"=w2131, "Value"=w2132) -> ()  [unwired: 2 in, 2 out]
                n1328 = property on="Show full track (analysis)" class="Bool (strict)"("DisabledEnum"=w2131, "Value"=w2132) -> ()  [unwired: 2 in, 2 out]
                n1329 = property on="Play/Pause" class="Bool (strict)"(error in=w2143, "DisabledEnum"=w2131) -> (error out=w2142:errorcluster)  [unwired: 1 in, 1 out]
                n1330 = property on="Back to Settings" class="Bool (strict)"(error in=w2142, "Visible"=TRUE, "Value"=FALSE ("Back to Settings")) -> (error out=w2137:errorcluster)  [unwired: 1 in, 1 out]
                n1331 = property on="Pane" class="Pane"(error in=w2137) -> (error out=w2130:errorcluster, "Decos[]"=w2133:refnum<vi>[])  [unwired: 1 in, 1 out]
                n1332 = Index Array(array=w2133, index=0) -> (element=w2135:refnum<vi>)
                n1333 = Index Array(array=w2133, index=2) -> (element=w2139:refnum<vi>)
                n1334 = property on="Map index (analysis)" class="DigNum (strict)"(error in=w2130, "Value"=0 ("Map index (analysis)")) -> (error out=w2127:errorcluster)  [unwired: 1 in, 1 out]
                n1335 = property class="Decor"(reference=w2135, "Visible"=TRUE) -> ()  [unwired: 1 in, 2 out]
                n1336 = property class="Decor"(reference=w2139, "Visible"=FALSE) -> ()  [unwired: 1 in, 2 out]
                n1337 = property on="Jump to Analysis" class="Bool (strict)"(error in=w2127, "Value"=FALSE ("Jump to Analysis")) -> ()  [unwired: 1 in, 2 out]
              }
            }
          }
        }
      }
      frame "Recording" {
        w2207 = FALSE ("use system decimal point (T)")
        n1338 = Divide(x=u32 1000, y=w2240) -> (x/y=w2239:dbl)
        n1339 = call <extravilib>:"Read.vi"("channel"=w2228) -> ("element"=w2204:string[][])  [unwired: 5 in, 5 out]
        n1340 = First Call?() -> (First Call?: T/F=w2187:bool)
        n1341 = feedback #9(w2235) -> (w2236:u32)
        n1342 = case shown="True" w2187 {
          tunnel: [w2326 w2327] -> w2166
          frame False {
            n1343 = property on="Type of histogram" class="DigNum (strict)"() -> ("Value"=w2326:u8)  [unwired: 2 in, 2 out]
          }
          frame True {
            w2327 = u8 3 ("Value (Signaling)")
            n1344 = property on="Type of histogram" class="DigNum (strict)"("Val(Sgnl)"=w2327) -> ()  [unwired: 2 in, 2 out]
          }
        }
        n1345 = Tick Count (ms)() -> (millisecond timer value=w2237:u32)
        n1346 = feedback-in #9(w2237) -> ()
        n1347 = call "FL_Last_N_Samples_2D_array_of_strings.vi"("BufferLengthSamples"=u32 5, "Input Array of strings"=w2204) -> ("Output Array of strings"=w2203:string[][])
        n1348 = Subtract(x=w2237, y=w2236) -> (x-y=w2234:u32)
        n1349 = Array Size(array=w2203) -> (size(s)=w2221:i32[])
        n1350 = global read "SW_Globals.vi" "Zones presence indicator"() -> (w2202:T56)
        n1351 = Multiply(x=w2239, y="Trace, s") -> (x*y=w2243:dbl)
        n1352 = Index Array(array=w2221, index=0) -> (element=w2219:i32)
        n1353 = Divide(x=w2234, y=u32 1000) -> (x/y=w2229:dbl)
        n1354 = event shown="[2] \"Histograms (normalized)\": Mouse Down;  \"Type of histogram\": Value Change" {
          selector: _ -> [_ _ _ _]
          dyn-events: _ -> [_ _ _ _]
          timeout: 0 -> [_ _ _ _]
          tunnel: w2166 -> [_ _ w2362 _]
          event Timeout {
            n1355 = event-data() -> ()  [unwired: 1 in, 3 out]
          }
          event "Multiplyer of chart RX": Value Change {
            n1356 = event-data() -> ("NewVal"=w2353:u8)  [unwired: 1 in, 5 out]
            n1357 = Multiply(x=w2353, y=10.0) -> (x*y=w2354:dbl)
            n1358 = property on="Mouse speed" class="WFChart (strict)"() -> (error out=w2355:errorcluster, "XScale.Maximum"=w2358:dbl)  [unwired: 2 in, 1 out]
            n1359 = Subtract(x=w2358, y=w2354) -> (x-y=w2356:dbl)
            n1360 = property on="Mouse speed" class="WFChart (strict)"(error in=w2355, "XScale.Minimum"=w2356) -> ()  [unwired: 1 in, 2 out]
          }
          event "Histograms (normalized)": Mouse Down; "Type of histogram": Value Change {
            n1361 = event-data() -> ()  [unwired: 1 in, 4 out]
            n1362 = Increment(x=w2362) -> (x+1=w2359:u8)
            n1363 = Quotient & Remainder(x=w2359, y=u8 4) -> (x-y*floor(x/y)=w2360:u8)  [unwired: 1 out]
            n1364 = case shown="0, Default" w2360 {
              frame 0, Default {
                w2366 = u8 0 ("X Scale.Display Format:Precision")
                w2374 = FALSE ("Speed distrib. indicator")
                w2365 = u8 1 ("X Scale.Scale Fit")
                w2367 = u32 15790320 ("Plot.Fill/Point Color")
                w2368 = u8 0 ("Y Scale.Mapping Mode")
                w2370 = 0.0 ("X Scale.Offset and Multiplier:Offset")
                w2371 = 1.0 ("X Scale.Offset and Multiplier:Multiplier")
                w2369 = u8 2 ("X Scale.Scale Fit")
                w2372 = "Zone preference (normalized)" ("Label.Text")
                # "Show zones preference"
                n1365 = Wait (ms)(milliseconds to wait=u32 100) -> ()  [unwired: 1 out]
                n1366 = property on="Zones presense indicator" class="Bool (strict)"("Value"=TRUE ("Zones presense indicator")) -> ()  [unwired: 2 in, 2 out]
                n1367 = property on="Run times distrib. indicator" class="Bool (strict)"("Value"=w2374) -> ()  [unwired: 2 in, 2 out]
                n1368 = property on="Run lengts distrib. indicator" class="Bool (strict)"("Value"=w2374) -> ()  [unwired: 2 in, 2 out]
                n1369 = property on="Speed distrib. indicator" class="Bool (strict)"("Value"=w2374) -> ()  [unwired: 2 in, 2 out]
                n1370 = global read "SW_Globals.vi" "Active segments amount"() -> (w2378:u8)
                n1371 = global read "SW_Globals.vi" "Zones normalized allocation array"() -> (w2364:dbl[])
                n1372 = Increment(x=w2378) -> (x+1=w2377:u8)
                n1373 = Bundle By Name(cluster=T21 {"Minimum"=0.0, "Maximum"=14.0, "Increment"=1.0, "Minor Increment"=1.0, "Start"=0.0} ("X Scale.Range"), "Maximum"=w2377) -> (w2373:T21)
                n1374 = Bundle("X Scale.Range"=w2373, "Label.Text"=w2372, "X Scale.Offset and Multiplier:Multiplier"=w2371, "X Scale.Offset and Multiplier:Offset"=w2370, "X Scale.Scale Fit"=w2369, "Y Scale.Mapping Mode"=w2368, "Zones preference empty initialized array"="Zones preference empty initialized array", "Plot.Fill/Point Color"=w2367, "X Scale.Scale Fit"=w2365, "X Scale.Display Format:Precision"=w2366) -> ()  [unwired: 1 in, 1 out]
                n1375 = property on="Histograms (normalized)" class="WFGraph (strict)"("XScale.Range"=w2373, "Caption.Text"=w2372, "XScale.Multiplier"=w2371, "XScale.Offset"=w2370, "XScale.ScaleFit"=w2369, "YScale.Mapping Mode"=w2368, "Value"=w2364, "Plot.Fill/Pt. Color"=w2367, "XScale.ScaleFit"=w2365, "XScale.Precision"=w2366) -> ()  [unwired: 2 in, 2 out]
              }
              frame 1 {
                w2380 = FALSE ("Zones presense indicator")
                # "Speed distribution"
                n1376 = Wait (ms)(milliseconds to wait=u32 100) -> ()  [unwired: 1 out]
                n1377 = property on="Speed distrib. indicator" class="Bool (strict)"("Value"=TRUE ("Speed distrib. indicator")) -> ()  [unwired: 2 in, 2 out]
                n1378 = property on="Run times distrib. indicator" class="Bool (strict)"("Value"=w2380) -> ()  [unwired: 2 in, 2 out]
                n1379 = property on="Run lengts distrib. indicator" class="Bool (strict)"("Value"=w2380) -> ()  [unwired: 2 in, 2 out]
                n1380 = property on="Zones presense indicator" class="Bool (strict)"("Value"=w2380) -> ()  [unwired: 2 in, 2 out]
                n1381 = global read "SW_Globals.vi" "Speed bins array"() -> (w2393:dbl[])
                n1382 = Array Size(array=w2393) -> (size(s)=w2395:i32)
                n1383 = global read "SW_Globals.vi" "Speed distribution array"() -> (w2386:u32[])
                n1384 = Decrement(x=w2395) -> (x-1=w2389:i32)
                n1385 = property on="Histograms (normalized)" class="WFGraph (strict)"("XScale.ScaleFit"=u8 0 ("X Scale.Scale Fit")) -> (error out=w2388:errorcluster)  [unwired: 2 in, 1 out]
                n1386 = Bundle By Name(cluster=T21 {"Minimum"=0.0, "Maximum"=14.0, "Increment"=1.0, "Minor Increment"=1.0, "Start"=0.0} ("X Scale.Range"), "Maximum"=w2389) -> (w2396:T21)
                n1387 = call "CALC_Normalize_1D_Array.vi"("1D array"=w2386) -> ("Normalized 1D array"=w2385:dbl[])  [unwired: 2 in, 1 out]
                n1388 = property on="Histograms (normalized)" class="WFGraph (strict)"(error in=w2388, "XScale.Range"=w2396, "Caption.Text"="Speed histogram (normalized)" ("Label.Text"), "XScale.Multiplier"=36.5 ("X Scale.Offset and Multiplier:Multiplier 2"), "XScale.Offset"=0 ("index"), "YScale.Mapping Mode"=u8 1 ("X Scale.Scale Fit"), "Value"=w2385, "Plot.Fill/Pt. Color"=u32 16777120 ("Plot.Fill/Point Color"), "XScale.ScaleFit"=u8 0 ("X Scale.Scale Fit")) -> ()  [unwired: 1 in, 2 out]
              }
              frame 2 {
                w2398 = FALSE ("Zones presense indicator")
                # "Runing bout distribution"
                n1389 = Wait (ms)(milliseconds to wait=u32 100) -> ()  [unwired: 1 out]
                n1390 = property on="Run lengts distrib. indicator" class="Bool (strict)"("Value"=TRUE ("Speed distrib. indicator")) -> ()  [unwired: 2 in, 2 out]
                n1391 = property on="Run times distrib. indicator" class="Bool (strict)"("Value"=w2398) -> ()  [unwired: 2 in, 2 out]
                n1392 = property on="Speed distrib. indicator" class="Bool (strict)"("Value"=w2398) -> ()  [unwired: 2 in, 2 out]
                n1393 = property on="Zones presense indicator" class="Bool (strict)"("Value"=w2398) -> ()  [unwired: 2 in, 2 out]
                n1394 = global read "SW_Globals.vi" "Run Lengths bins array"() -> (w2404:dbl[])
                n1395 = Array Size(array=w2404) -> (size(s)=w2418:i32)
                n1396 = Decrement(x=w2418) -> (x-1=w2399:i32)
                n1397 = global read "SW_Globals.vi" "Run Lengts distribution array"() -> (w2411:u32[])
                n1398 = property on="Histograms (normalized)" class="WFGraph (strict)"("XScale.ScaleFit"=u8 0 ("X Scale.Scale Fit")) -> (error out=w2413:errorcluster)  [unwired: 2 in, 1 out]
                n1399 = Array Subset(array=w2404, index=0, length=w2399) -> ()  [unwired: 1 out]
                n1400 = Bundle By Name(cluster=T21 {"Minimum"=0.0, "Maximum"=2.0, "Increment"=0.2, "Minor Increment"=0.2, "Start"=0.0} ("X Scale.Range"), "Maximum"=w2399) -> (w2400:T21)
                n1401 = call "CALC_Normalize_1D_Array.vi"("1D array"=w2411) -> ("Normalized 1D array"=w2410:dbl[])  [unwired: 2 in, 1 out]
                n1402 = property on="Histograms (normalized)" class="WFGraph (strict)"(error in=w2413, "XScale.Range"=w2400, "Caption.Text"="Running bout dist. hist. (norm.)" ("Label.Text"), "XScale.Multiplier"=0.2 ("X Scale.Offset and Multiplier:Multiplier 2"), "XScale.Offset"=0.2 ("index"), "YScale.Mapping Mode"=u8 0 ("X Scale.Scale Fit"), "Value"=w2410, "Plot.Fill/Pt. Color"=u32 12320699 ("Plot.Fill/Point Color"), "XScale.ScaleFit"=u8 1 ("X Scale.Scale Fit"), "XScale.Format"=u8 0 ("X Scale.Display Format:Format"), "XScale.Precision"=u8 1 ("X Scale.Display Format:Precision")) -> ()  [unwired: 1 in, 2 out]
              }
              frame 3 {
                w2419 = FALSE ("Zones presense indicator")
                # "Running times distribution"
                n1403 = Wait (ms)(milliseconds to wait=u32 100) -> ()  [unwired: 1 out]
                n1404 = property on="Run times distrib. indicator" class="Bool (strict)"("Value"=TRUE ("Run times distrib. indicator")) -> ()  [unwired: 2 in, 2 out]
                n1405 = property on="Run lengts distrib. indicator" class="Bool (strict)"("Value"=w2419) -> ()  [unwired: 2 in, 2 out]
                n1406 = property on="Speed distrib. indicator" class="Bool (strict)"("Value"=w2419) -> ()  [unwired: 2 in, 2 out]
                n1407 = property on="Zones presense indicator" class="Bool (strict)"("Value"=w2419) -> ()  [unwired: 2 in, 2 out]
                n1408 = global read "SW_Globals.vi" "Run Times bins array"() -> (w2426:dbl[])
                n1409 = Array Size(array=w2426) -> (size(s)=w2439:i32)
                n1410 = Decrement(x=w2439) -> (x-1=w2421:i32)
                n1411 = global read "SW_Globals.vi" "Run Times distribution array"() -> (w2432:u32[])
                n1412 = property on="Histograms (normalized)" class="WFGraph (strict)"("XScale.ScaleFit"=u8 0 ("X Scale.Scale Fit")) -> (error out=w2434:errorcluster)  [unwired: 2 in, 1 out]
                n1413 = Array Subset(array=w2426, index=0, length=w2421) -> ()  [unwired: 1 out]
                n1414 = Bundle By Name(cluster=T21 {"Minimum"=0.0, "Maximum"=2.0, "Increment"=0.2, "Minor Increment"=0.2, "Start"=0.0} ("X Scale.Range"), "Maximum"=w2421) -> (w2422:T21)
                n1415 = call "CALC_Normalize_1D_Array.vi"("1D array"=w2432) -> ("Normalized 1D array"=w2431:dbl[])  [unwired: 2 in, 1 out]
                n1416 = property on="Histograms (normalized)" class="WFGraph (strict)"(error in=w2434, "XScale.Range"=w2422, "Caption.Text"="Run times dist. hist. (norm.)" ("Label.Text"), "XScale.Multiplier"=1.0 ("X Scale.Offset and Multiplier:Multiplier 2"), "XScale.Offset"=0.5 ("index"), "YScale.Mapping Mode"=u8 0 ("X Scale.Scale Fit"), "Value"=w2431, "Plot.Fill/Pt. Color"=u32 16771022 ("Plot.Fill/Point Color"), "XScale.ScaleFit"=u8 1 ("X Scale.Scale Fit"), "XScale.Format"=u8 0 ("X Scale.Display Format:Format"), "XScale.Precision"=u8 1 ("X Scale.Display Format:Precision")) -> ()  [unwired: 1 in, 2 out]
              }
            }
            n1417 = property on="Type of histogram" class="DigNum (strict)"("Value"=w2360) -> ()  [unwired: 2 in, 2 out]
          }
          event "Additional record settings": Value Change {
            n1418 = event-data() -> ("OldVal"=w2457:bool)  [unwired: 1 in, 5 out]
            n1419 = property on="Additional record settings" class="Bool (strict)"("Value"=w2457) -> ()  [unwired: 2 in, 2 out]
            n1420 = property on="Twisted neck" class="Bool (strict)"() -> ("Value"=w2444:bool)  [unwired: 2 in, 2 out]
            n1421 = property on="Bridge horizontal offset" class="DigNum (strict)"() -> ("Value"=w2443:sgl)  [unwired: 2 in, 2 out]
            n1422 = property on="Name Prefix" class="Str"() -> ("Value"=w2442:string)  [unwired: 2 in, 2 out]
            n1423 = property on="Stop record at" class="DigNum (strict)"() -> ("Value"=w2441:dbl)  [unwired: 2 in, 2 out]
            n1424 = property on="Bridge offset" class="DigNum (strict)"() -> ("Value"=w2454:sgl)  [unwired: 2 in, 2 out]
            n1425 = property on="Bridge swap" class="Bool (strict)"() -> ("Value"=w2453:bool)  [unwired: 2 in, 2 out]
            n1426 = property on="\"Stop at\" enabled" class="Bool (strict)"() -> ("Value"=w2440:bool)  [unwired: 2 in, 2 out]
            n1427 = Bundle By Name(cluster=T48 {"Offset V."=0.0, "Offset H."=0.0, "Bridge swap"=FALSE, "Twisted neck"=FALSE, "Name prefix"="SavedTrack", "Stop at"=0.0, "\"Stop at\" enabled"=FALSE} ("Offsets, swaps and rotations in"), "Offset V."=w2454, "Bridge swap"=w2453, "Twisted neck"=w2444, "Name prefix"=w2442, "Stop at"=w2441, "\"Stop at\" enabled"=w2440, "Offset H."=w2443) -> (w2455:T48)
            n1428 = call "SW_Set_Add_Recording_Settings.vi"("Offsets, swaps and rotations in"=w2455) -> ("Offsets, swaps and rotations out"=w2452:T48)  [unwired: 1 in]
            n1429 = Unbundle By Name(w2452) -> ("Offset V."=w2451:sgl, "Offset H."=w2448:sgl, "Bridge swap"=w2450:bool, "Twisted neck"=w2449:bool, "Name prefix"=w2445:string, "Stop at"=w2447:dbl, "\"Stop at\" enabled"=w2446:bool)
            n1430 = property on="\"Stop at\" enabled" class="Bool (strict)"("Value"=w2446) -> ()  [unwired: 2 in, 2 out]
            n1431 = property on="Bridge offset" class="DigNum (strict)"("Value"=w2451) -> ()  [unwired: 2 in, 2 out]
            n1432 = property on="Name Prefix" class="Str"("Value"=w2445) -> ()  [unwired: 2 in, 2 out]
            n1433 = property on="Stop record at" class="DigNum (strict)"("Value"=w2447) -> ()  [unwired: 2 in, 2 out]
            n1434 = property on="Bridge swap" class="Bool (strict)"("Value"=w2450) -> ()  [unwired: 2 in, 2 out]
            n1435 = property on="Bridge horizontal offset" class="DigNum (strict)"("Value"=w2448) -> ()  [unwired: 2 in, 2 out]
            n1436 = property on="Twisted neck" class="Bool (strict)"("Value"=w2449) -> ()  [unwired: 2 in, 2 out]
            n1437 = disable-structure shown="Disabled" {
              disable-tunnel: w2445 -> [w2458 _]
              frame Disabled {
                n1438 = global read "SW_Globals.vi" "Cluster of paths"() -> (w2460:T22)
                n1439 = call "SW_Get_save_paths.vi"("Input cluster of paths"=w2460, "Final file name prefix"=w2458) -> ("Output cluster of paths"=w2459:T22)  [unwired: 2 in, 2 out]
                n1440 = global write "SW_Globals.vi" "Cluster of paths"(w2459) -> ()
              }
              frame Enabled {
              }
            }
          }
        }
        n1441 = Round To Nearest(number=w2243) -> (nearest integer value=w2242:dbl)
        n1442 = Decrement(x=w2219) -> (x-1=w2218:i32)
        n1443 = property on="Zones presence indicator" class="Clust"("Value"=w2202) -> ()  [unwired: 2 in, 2 out]
        n1444 = Index Array(array=w2203, index (row)=w2218) -> (element=w2167:string[])  [unwired: 1 in]
        n1445 = Index Array "Timestamp"(array=w2167, index=4) -> (element=w2216:string)
        n1446 = Index Array "X (filtered)"(array=w2167, index=9) -> (element=w2210:string)
        n1447 = Index Array "Y (filtered)"(array=w2167, index=10) -> (element=w2209:string)
        n1448 = Index Array "w (mouse rot. angle)"(array=w2167, index=8) -> (element=w2208:string)
        n1449 = global read "SW_Globals.vi" "Diagram no zones"() -> (w2249:picture)
        n1450 = String Length(string=w2216) -> (length=w2215:i32)
        n1451 = Fract/Exp String To Number(use system decimal point (T)=w2207, string=w2210) -> (number=w2169:dbl)  [unwired: 2 in, 1 out]
        n1452 = Fract/Exp String To Number(use system decimal point (T)=w2207, string=w2209) -> (number=w2170:dbl)  [unwired: 2 in, 1 out]
        n1453 = global read "SW_Globals.vi" "Diagram"() -> (w2250:picture)
        n1454 = property on="Diagram at recording" class="Pict"() -> ("Bounds"=w2247:T19)  [unwired: 2 in, 2 out]
        n1455 = global read "SW_Globals.vi" "Speed bins array"() -> (w2200:dbl[])
        n1456 = local read "Pixels per mm"() -> (w2248:dbl)
        n1457 = Fract/Exp String To Number(use system decimal point (T)=w2207, string=w2208) -> (number=w2168:dbl)  [unwired: 2 in, 1 out]
        n1458 = Select(t=w2250, s="Zones", f=w2249) -> (s? t:f=w2251:picture)
        n1459 = Greater Than 0?(x=w2215) -> (x > 0?=w2214:bool)
        n1460 = Not(x="Zones") -> (.not. x?=w2245:bool)
        n1461 = call "FL_Calc_speed_on_the_fly.vi"("Y coord, mm"=w2170, "X coord, mm"=w2169, "Time per frame, s"=w2229) -> ("Mouse speed, mm/s"=w2183:dbl)
        "Mouse speed digi" <- w2183
        n1462 = global read "SW_Globals.vi" "Speed distribution array"() -> (w2196:u32[])
        n1463 = case shown="True" w2214 {
          tunnel: [w2331 w2334] -> w2171
          tunnel: w2216 -> [_ w2333]
          frame False {
            n1464 = Get Date/Time In Seconds() -> (seconds since 1Jan1904=w2331:timestamp)
          }
          frame True {
            (unwired) "%<%H:%M:%S%3u%p%d.%m.%Y>T" ("format string")
            n1465 = Get Date/Time In Seconds() -> (seconds since 1Jan1904=w2332:timestamp)
            n1466 = Scan From String(format string="%<%H:%M:%S%,;%3u %d.%m.%Y>T", input string=w2333, default 1=w2332) -> (output 1=w2334:timestamp)  [unwired: 2 in, 3 out]
          }
        }
        n1467 = call "SW_Draw_mouse_br.vi"("Input picture (background)"=w2251, "Size of the image"=w2247, "Pixels per mm"=w2248, "Mouse coord cartesian X, mm"=w2169, "Mouse coord cartesian Y, mm"=w2170, "Mouse angle of rotation, deg"=w2168, "Show mouse lineout"=w2245, "Trace length, samples"=w2242) -> ("Output picture (with mouse overlay)"=→"Diagram at recording":picture)  [unwired: 6 in, 1 out]
        n1468 = call "FL_Get_Histogram_Bin_value.vi"("Current value"=w2183, "Bins array"=w2200) -> ("Bin assignment"=w2199:i32)
        n1469 = global read "SW_Globals.vi" "Run Lengts distribution array"() -> (w2181:u32[])
        n1470 = global read "SW_Globals.vi" "Run Times distribution array"() -> (w2178:u32[])
        n1471 = Index Array(array=w2196, index=w2199) -> (element=w2198:u32)
        n1472 = global read "SW_Globals.vi" "Run Lengths bins array"() -> (w2180:dbl[])
        n1473 = global read "SW_Globals.vi" "Run Times bins array"() -> (w2177:dbl[])
        n1474 = global read "SW_Globals.vi" "Speed detection threshold, mm/s"() -> (w2172:dbl)
        n1475 = Increment(x=w2198) -> (x+1=w2197:u32)
        n1476 = call "FL_Get_Run_Bout_and_Time.vi"("Speed, mm/s"=w2183, "Run Lengts distribution array in"=w2181, "Speed lower threshold, mm/s"=w2172, "Run times distribution array in"=w2178, "Run Lengths bin array"=w2180, "Run times bin array"=w2177) -> ("Run Lengts distribution array out"=w2179:u32[], "Run time, s"=w2174:dbl, "Run times distribution array out"=w2176:u32[])  [unwired: 1 in]
        n1477 = Replace Array Subset(array=w2196, new element=w2197, index=w2199) -> (w2195:u32[])
        n1478 = property on="Type of histogram" class="DigNum (strict)"() -> ("Value"=w2184:u8)  [unwired: 2 in, 2 out]
        n1479 = global write "SW_Globals.vi" "Run time, s"(w2174) -> ()
        n1480 = global write "SW_Globals.vi" "Run Lengts distribution array"(w2179) -> ()
        n1481 = global write "SW_Globals.vi" "Run Times distribution array"(w2176) -> ()
        n1482 = global write "SW_Globals.vi" "Speed distribution array"(w2195) -> ()
        n1483 = call "CALC_Normalize_1D_Array.vi"("1D array"=w2179) -> ("Normalized 1D array"=w2182:dbl[])  [unwired: 2 in, 1 out]
        n1484 = call "CALC_Normalize_1D_Array.vi"("1D array"=w2176) -> ("Normalized 1D array"=w2175:dbl[])  [unwired: 2 in, 1 out]
        n1485 = call "CALC_Normalize_1D_Array.vi"("1D array"=w2195) -> ("Normalized 1D array"=w2185:dbl[])  [unwired: 2 in, 1 out]
        n1486 = case shown="0, Default" w2184 {
          tunnel: [w2322 w2323 w2324 w2325] -> w2186
          tunnel: w2185 -> [_ w2323 _ _]
          tunnel: w2182 -> [_ _ w2324 _]
          tunnel: w2175 -> [_ _ _ w2325]
          frame 0, Default {
            n1487 = global read "SW_Globals.vi" "Zones normalized allocation array"() -> (w2322:dbl[])
          }
          frame 1 {
          }
          frame 2 {
          }
          frame 3 {
          }
        }
        "Histograms (normalized)" <- w2186
        n1488 = Delete From Array(array=w2185, length=1, index=0) -> (array with subset deleted=w2192:dbl[])  [unwired: 1 out]
        n1489 = for {
          tunnel: w2192 -> [w2330] mode=indexing
          shift-right: [w2329] -> w2190
          shift-left: 0.0 -> [w2328]
          n1490 = Add(x=w2328, y=w2330) -> (x+y=w2329:dbl)
        }
        n1491 = Not(x="Exit (recording)") -> (.not. x?=w2224:bool)
        n1492 = And(x=w2224, y="Record/Stop") -> (x .and. y?=w2225:bool)
        n1493 = Multiply(x=w2190, y=100.0) -> (x*y=→"Mouse running, perc. of time":dbl)
        n1494 = Build Array(w2183) -> (w2227:dbl[])
        n1495 = property on="Current Time" class="AbsTime (strict)"("Value"=w2171) -> ()  [unwired: 2 in, 2 out]
        n1496 = Bundle By Name("t0"=w2171, "Y"=w2227) -> (→"Mouse speed":waveform(dbl))  [unwired: 1 in]
        n1497 = case shown="True" w2225 {
          tunnel: w2173 -> [w2463 w2557]
          tunnel: w2171 -> [_ w2556]
          tunnel: w2238 -> [_ w2555]
          tunnel: [w2465 w2553] -> w2230
          tunnel: "Exit (recording)" -> [w2462 _]
          frame False {
            n1498 = Unbundle By Name(w2463) -> ("Has been recorded"=w2467:refnum<notifier>)
            n1499 = Get Notifier Status(notifier=w2467) -> (current notification=w2461:bool, error out=w2466:errorcluster)  [unwired: 1 in, 3 out]
            n1500 = Or(x=w2462, y=w2461) -> (x .or. y?=w2464:bool)
            n1501 = case shown="True" w2464 {
              tunnel: w2463 -> [_ w2530]
              tunnel: w2466 -> [_ w2509]
              tunnel: [FALSE FALSE] -> w2465
              tunnel: w2461 -> [_ w2489]
              frame False {
                w2468 = FALSE ("Show full track (analysis)")
                n1502 = property on="Start TTL is fired" class="Bool (strict)"("Value"=FALSE ("Start TTL is fired")) -> ()  [unwired: 2 in, 2 out]
                n1503 = property on="Stop TTL is fired" class="Bool (strict)"("Value"=FALSE ("Start TTL is fired")) -> ()  [unwired: 2 in, 2 out]
                n1504 = property on="Show full track (analysis)" class="Bool (strict)"("Value"=w2468) -> ()  [unwired: 2 in, 2 out]
                n1505 = property on="Show heatmap (analysis)" class="Bool (strict)"("Value"=w2468) -> ()  [unwired: 2 in, 2 out]
                n1506 = disable-structure shown="Disabled" {
                  frame Disabled {
                    n1507 = global read "SW_Globals.vi" "Cluster of paths"() -> (w2481:T22)
                    n1508 = Unbundle By Name(w2481) -> ("Path to the settings file"=w2474:path)
                    n1509 = property on="Bridge swap" class="Bool (strict)"() -> (error out=w2475:errorcluster, "Value"=w2472:bool)  [unwired: 2 in, 1 out]
                    n1510 = local read "Current User"() -> (w2473:string)
                    n1511 = call <vilib>:"Open Config Data.vi"("error in (no error)"=w2475, "create file if necessary (T)"=w2472, "configuration file path"=w2474) -> ("error out"=w2478:errorcluster, "refnum"=w2480:T5)  [unwired: 6 in, 1 out]
                    n1512 = call <vilib>:"Write Key (Boolean).vi"("section"=w2473, "error in (no error)"=w2478, "key"="Bridge swap?", "refnum"=w2480) -> ("error out"=w2477:errorcluster, "refnum out"=w2479:T5)  [unwired: 5 in, 1 out]
                    n1513 = call <vilib>:"Close Config Data.vi"("error in (no error)"=w2477, "refnum"=w2479) -> ()  [unwired: 8 in, 2 out]
                  }
                  frame Enabled {
                  }
                }
              }
              frame True {
                w2515 = enum32{"Settings", "Recording", "Analysis"}."Analysis" ("Main tab control")
                w2519 = enum32{"Settings", "Recording", "Analysis"}."Recording" ("Main tab control")
                w2528 = enum32{"Settings", "Recording", "Analysis"}."Settings" ("Main tab control")
                n1514 = flat-sequence {
                  tunnel: w2530 -> [w2538]
                  tunnel: w2509 -> [w2534]
                  tunnel: [w2531] -> w2508
                  tunnel: [w2540] -> w2484
                  tunnel: w2508 -> [w2540]
                  frame #0 {
                    n1515 = Unbundle By Name(w2538) -> ("Play/Pause status"=w2539:refnum<notifier>, "Recording now"=w2536:refnum<notifier>)
                    n1516 = Send Notification(notification=FALSE, notifier=w2536, error in (no error)=w2534) -> (error out=w2532:errorcluster)  [unwired: 1 out]
                    n1517 = Send Notification(notification="Pause" ("f"), notifier=w2539) -> (error out=w2533:errorcluster)  [unwired: 1 in, 1 out]
                    n1518 = Merge Errors(w2533, w2532) -> (w2531:errorcluster)
                  }
                  frame #1 {
                    n1519 = Wait (ms)(milliseconds to wait=u32 500) -> ()  [unwired: 1 out]
                  }
                }
                n1520 = property on="Additional record settings" class="Bool (strict)"(error in=w2484, "BoolText.Text"="Set" ("Boolean Text.Text")) -> (error out=w2483:errorcluster)  [unwired: 1 in, 1 out]
                n1521 = property on="Exit (recording)" class="Bool"(error in=w2483, "DisabledEnum"=T12."Enabled" ("Disabled")) -> (error out=w2507:errorcluster)  [unwired: 1 in, 1 out]
                n1522 = property on="Main tab control" class="TabCtl (strict)"(error in=w2507, "Value"=w2528) -> (error out=w2524:errorcluster, "Pages"=w2529:refnum<vi>[])  [unwired: 1 in, 1 out]
                n1523 = To Long Integer(number=w2528) -> (32bit integer=w2527:i32)
                n1524 = Index Array(array=w2529, index=w2527) -> (element=w2526:refnum<vi>)
                n1525 = property class="Page"(reference=w2526, error in=w2524, "PageEnb"=T32."Page Disabled & Grayed" ("Page Enabled State")) -> (error out=w2517:errorcluster)  [unwired: 1 out]
                n1526 = property on="Main tab control" class="TabCtl (strict)"(error in=w2517, "Value"=w2519) -> (error out=w2523:errorcluster, "Pages"=w2518:refnum<vi>[])  [unwired: 1 in, 1 out]
                n1527 = To Long Integer(number=w2519) -> (32bit integer=w2520:i32)
                n1528 = Index Array(array=w2518, index=w2520) -> (element=w2521:refnum<vi>)
                n1529 = property class="Page"(reference=w2521, error in=w2523, "PageEnb"=T32."Page Disabled & Grayed" ("Page Enabled State")) -> (error out=w2510:errorcluster)  [unwired: 1 out]
                n1530 = property on="Main tab control" class="TabCtl (strict)"(error in=w2510, "Value"=w2515) -> (error out=w2511:errorcluster, "Pages"=w2516:refnum<vi>[])  [unwired: 1 in, 1 out]
                n1531 = To Long Integer(number=w2515) -> (32bit integer=w2514:i32)
                n1532 = Index Array(array=w2516, index=w2514) -> (element=w2513:refnum<vi>)
                n1533 = property class="Page"(reference=w2513, error in=w2511, "PageEnb"=T32."Page Enabled" ("Page Enabled State")) -> (error out=w2496:errorcluster)  [unwired: 1 out]
                n1534 = property on="Pane" class="Pane"(error in=w2496) -> (error out=w2495:errorcluster, "Decos[]"=w2497:refnum<vi>[])  [unwired: 1 in, 1 out]
                n1535 = Index Array(array=w2497, index=1) -> (element=w2502:refnum<vi>)
                n1536 = property class="Decor"(reference=w2502, error in=w2495, "Visible"=FALSE) -> (error out=w2494:errorcluster)  [unwired: 1 out]
                n1537 = Index Array(array=w2497, index=0) -> (element=w2499:refnum<vi>)
                n1538 = property class="Decor"(reference=w2499, error in=w2494, "Visible"=TRUE) -> (error out=w2493:errorcluster)  [unwired: 1 out]
                n1539 = property on="Back to Settings" class="Bool (strict)"(error in=w2493, "Visible"=TRUE) -> (error out=w2486:errorcluster)  [unwired: 1 in, 1 out]
                n1540 = Select(t=T12."Enabled" ("Disabled"), s=w2489, f=T12."Disabled and Grayed Out" ("Disabled")) -> (s? t:f=w2488:T12)
                n1541 = property on="Show heatmap (analysis)" class="Bool (strict)"(error in=w2486, "DisabledEnum"=w2488) -> (error out=w2491:errorcluster)  [unwired: 1 in, 1 out]
                n1542 = property on="Show full track (analysis)" class="Bool (strict)"(error in=w2491, "DisabledEnum"=w2488) -> (error out=w2490:errorcluster)  [unwired: 1 in, 1 out]
                n1543 = property on="Map index (analysis)" class="DigNum (strict)"(error in=w2490, "Value"=0 ("Map index (analysis)")) -> ()  [unwired: 1 in, 2 out]
              }
            }
          }
          frame True {
            n1544 = flat-sequence {
              tunnel: w2556 -> [w2567]
              tunnel: [w2574] -> w2558
              tunnel: w2557 -> [w2571]
              tunnel: w2556 -> [w2569]
              tunnel: [w2569] -> w2554
              tunnel: w2555 -> [w2568]
              tunnel: [w2566] -> w2553
              frame #0 {
                n1545 = case shown="True" "Record start First Call" {
                  tunnel: w2567 -> [_ w2657]
                  tunnel: [w2579 w2657] -> w2574
                  tunnel: [_ w2672] -> w2570
                  tunnel: w2568 -> [_ w2678]
                  tunnel: [FALSE TRUE] -> w2566
                  frame False {
                    n1546 = global read "SW_Globals.vi" "Recording start timestamp"() -> (w2579:timestamp)
                  }
                  frame True {
                    w2599 = FALSE ("use system decimal point (T)")
                    w2639 = 400
                    w2638 = "NI_MinimumBufferSize"
                    w2619 = T12."Disabled and Grayed Out" ("Disabled")
                    n1547 = property on="Record start First Call" class="Bool (strict)"("Value"=FALSE ("Record start First Call")) -> ()  [unwired: 2 in, 2 out]
                    n1548 = property on="Stimulus presets" class="Arr (strict)"() -> ("Value"=w2649:T7)  [unwired: 2 in, 2 out]
                    n1549 = for {
                      tunnel: w2649 -> [w2703] mode=indexing
                      shift-right: [w2696] -> w2647
                      shift-left: string[] [] -> [w2695]
                      i -> [w2702]
                      n1550 = Unbundle By Name(w2703) -> ("Stim. has been set"=w2699:bool)
                      n1551 = Flatten To JSON(anything=w2703) -> (JSON string=w2697:string)  [unwired: 2 in, 1 out]
                      n1552 = Format Value(string ("")="Zone " ("string"), format string="%02d", value (0)=w2702) -> (output string=w2698:string)
                      n1553 = case shown="True" w2699 {
                        tunnel: w2698 -> [_ w2710]
                        tunnel: w2697 -> [_ w2708]
                        tunnel: [w2704 w2706] -> w2696
                        tunnel: w2695 -> [w2704 w2705]
                        frame False {
                        }
                        frame True {
                          n1554 = Concatenate Strings(w2710, ": " ("string"), w2708) -> (w2707:string)
                          n1555 = Build Array (concatenate)(w2705, w2707) -> (w2706:string[])
                        }
                      }
                    }
                    n1556 = property on="\"Stop at\" enabled" class="Bool (strict)"() -> ("Value"=w2594:bool)  [unwired: 2 in, 2 out]
                    n1557 = property on="Stop record at" class="DigNum (strict)"() -> ("Value"=w2597:dbl)  [unwired: 2 in, 2 out]
                    n1558 = property on="Bridge horizontal offset" class="DigNum (strict)"() -> ("Value"=w2607:sgl)  [unwired: 2 in, 2 out]
                    n1559 = property on="Twisted neck" class="Bool (strict)"() -> ("Value"=w2612:bool)  [unwired: 2 in, 2 out]
                    n1560 = local read "Starting angle MIDFIELD"() -> (w2664:i16)
                    n1561 = local read "Starting angle BORDER"() -> (w2667:i16)
                    n1562 = local read "N segments MIDFIELD"() -> (w2665:u8)
                    n1563 = local read "Radius, mm MIDFIELD"() -> (w2663:u16)
                    n1564 = local read "N segments BORDER"() -> (w2666:u8)
                    n1565 = local read "Radius, mm CENTER"() -> (w2661:u16)
                    n1566 = local read "Cage diameter, mm"() -> (w2645:u16)
                    n1567 = property on="IO parameters string" class="Str"() -> ("Value"=w2646:string)  [unwired: 2 in, 2 out]
                    n1568 = property on="Bridge offset" class="DigNum (strict)"() -> ("Value"=w2621:sgl)  [unwired: 2 in, 2 out]
                    n1569 = property on="Bridge swap" class="Bool (strict)"() -> ("Value"=w2620:bool)  [unwired: 2 in, 2 out]
                    n1570 = property on="Data filtering" class="Ring (strict)"() -> ("Value"=w2580:u16)  [unwired: 2 in, 2 out]
                    n1571 = local read "Current User"() -> (w2584:string)
                    n1572 = property on="Name Prefix" class="Str"() -> ("Value"=w2603:string)  [unwired: 2 in, 2 out]
                    n1573 = Bundle By Name ("Geometrical parameters")(cluster=T49 {"N segments BORDER"=0, "Starting angle BORDER"=0, "N segments MIDFIELD"=0, "Starting angle MIDFIELD"=0, "Radius, mm MIDFIELD"=0, "Amount of central segments"=0, "Radius, mm CENTER"=0, "Bridge swap"=FALSE, "Bridge V. offset"=0.0, "Twisted neck"=FALSE, "Offset H."=0.0, "Zones configuration"=[], "IO parameters string"="[12,1,1,0,0,0]", "Cage diameter, mm"=180, "Name prefix"="SavedTrack", "Stop at"=0.0, "\"Stop at\" enabled"=FALSE, "Data filtering"=0} ("Parameters"), "N segments BORDER"=w2666, "Starting angle BORDER"=w2667, "N segments MIDFIELD"=w2665, "Starting angle MIDFIELD"=w2664, "Radius, mm MIDFIELD"=w2663, "Amount of central segments"=u8 1, "Radius, mm CENTER"=w2661, "Bridge V. offset"=w2621, "Bridge swap"=w2620, "Zones configuration"=w2647, "IO parameters string"=w2646, "Cage diameter, mm"=w2645, "Twisted neck"=w2612, "Offset H."=w2607, "Name prefix"=w2603, "Stop at"=w2597, "\"Stop at\" enabled"=w2594, "Data filtering"=w2580) -> (w2650:T49)
                    n1574 = global read "SW_Globals.vi" "Cluster of paths"() -> (w2674:T22)
                    n1575 = local read "Current User"() -> (w2658:string)
                    n1576 = call "SW_Get_save_paths.vi"("Input cluster of paths"=w2674, "Final file name prefix"=w2603) -> ("error out"=w2602:errorcluster, "Saved track name"=w2659:string, "Output cluster of paths"=w2591:T22)  [unwired: 2 in]
                    n1577 = Format Date/Time String(seconds (now)=w2657, UTC format=FALSE) -> (date/time string=w2656:string)  [unwired: 1 in]
                    n1578 = Flatten To JSON(enable LabVIEW extensions? (T)=TRUE, anything=w2650) -> (JSON string=w2653:string, 11:w2644:errorcluster)  [unwired: 1 in]
                    n1579 = Unbundle By Name(w2591) -> ("TDMS file reference"=w2634:refnum<k34>, "Path to the settings file"=w2630:path, "Recording settings output path"=w2588:path)
                    n1580 = call <vilib>:"Open Config Data.vi"("create file if necessary (T)"=TRUE, "configuration file path"=w2630) -> ("error out"=w2626:errorcluster, "refnum"=w2628:T5)  [unwired: 7 in, 1 out]
                    n1581 = call <vilib>:"Write Key (Boolean).vi"("section"=w2584, "error in (no error)"=w2626, "value"=w2620, "key"="Bridge swap?", "refnum"=w2628) -> ("error out"=w2624:errorcluster, "refnum out"=w2625:T5)  [unwired: 4 in, 1 out]
                    n1582 = call <vilib>:"Write Key (Double).vi"("use system decimal point (T)"=w2599, "precision (6)"=i16 2, "section"=w2584, "error in (no error)"=w2624, "value"=w2621, "key"="Bridge offset", "refnum"=w2625) -> ("error out"=w2614:errorcluster, "refnum out"=w2615:T5)  [unwired: 2 in, 1 out]
                    n1583 = call <vilib>:"Write Key (Boolean).vi"("section"=w2584, "error in (no error)"=w2614, "value"=w2612, "key"="Twisted neck", "refnum"=w2615) -> ("error out"=w2611:errorcluster, "refnum out"=w2610:T5)  [unwired: 4 in, 1 out]
                    n1584 = call <vilib>:"Write Key (Double).vi"("use system decimal point (T)"=w2599, "precision (6)"=i16 2, "section"=w2584, "error in (no error)"=w2611, "value"=w2607, "key"="Offset H.", "refnum"=w2610) -> ("error out"=w2606:errorcluster, "refnum out"=w2605:T5)  [unwired: 2 in, 1 out]
                    n1585 = call <vilib>:"Write Key (String).vi"("section"=w2584, "error in (no error)"=w2606, "value"=w2603, "key"="Name prefix", "refnum"=w2605) -> ("error out"=w2600:errorcluster, "refnum out"=w2601:T5)  [unwired: 4 in, 1 out]
                    n1586 = call <vilib>:"Write Key (Double).vi"("use system decimal point (T)"=w2599, "precision (6)"=i16 2, "section"=w2584, "error in (no error)"=w2600, "value"=w2597, "key"="Stop at", "refnum"=w2601) -> ("error out"=w2596:errorcluster, "refnum out"=w2595:T5)  [unwired: 2 in, 1 out]
                    n1587 = call <vilib>:"Write Key (Boolean).vi"("section"=w2584, "error in (no error)"=w2596, "value"=w2594, "key"="\"Stop at\" enabled", "refnum"=w2595) -> ("error out"=w2586:errorcluster, "refnum out"=w2583:T5)  [unwired: 4 in, 1 out]
                    n1588 = global write "SW_Globals.vi" "Cluster of paths"(w2591) -> ()
                    n1589 = Build Array(w2659, w2658, w2656, w2653) -> (w2655:string[])
                    n1590 = call <vilib>:"Write Key (U32).vi"("section"=w2584, "error in (no error)"=w2586, "value"=w2580, "key"="Data filtering", "refnum"=w2583) -> ("error out"=w2585:errorcluster, "refnum out"=w2582:T5)  [unwired: 4 in, 1 out]
                    n1591 = call <vilib>:"Close Config Data.vi"("error in (no error)"=w2585, "refnum"=w2582) -> ("error out"=w2616:errorcluster, "file path"=w2590:path)  [unwired: 8 in]
                    n1592 = Copy(9:TRUE ("overwrite (F)"), 10:w2588, 11:w2590) -> (0:w2587:errorcluster)  [unwired: 2 in, 2 out]
                    n1593 = Flush Queue(queue=w2678) -> (error out=w2676:errorcluster)  [unwired: 1 in, 2 out]
                    n1594 = TDMS Set Properties(5:w2655, 7:string[] ["Title", "Author", "DateTime", "Description", ""] ("property names"), 8:w2644, 11:w2634) -> (0:w2640:errorcluster, 3:w2643:refnum<k34>)  [unwired: 2 in, 2 out]
                    n1595 = for {
                      tunnel: w2643 -> [w2694]
                      tunnel: string[] ["X1_raw", "Y1_raw", "X2_raw", "Y2_raw"] ("Columns Names") -> [w2693] mode=indexing
                      tunnel: "Raw_data" ("group name in (Untitled)") -> [w2692]
                      tunnel: w2638 -> [w2691]
                      tunnel: w2639 -> [w2690]
                      tunnel: w2640 -> [w2689]
                      tunnel: [w2688] -> w2637
                      tunnel: [w2687] -> w2636
                      n1596 = TDMS Set Properties(5:w2690, 7:w2691, 8:w2689, 9:w2693, 10:w2692, 11:w2694) -> (0:w2687:errorcluster, 3:w2688:refnum<k34>)  [unwired: 2 out]
                    }
                    n1597 = for {
                      tunnel: string[] ["Absolute_timestamp", "Relative_timestamp", "Key", "R", "phi", "alpha", "X", "Y", "w", "Speed_mm_per_s", "Current_zone", "TTL_inputs", "TTL_outputs", "Zones_preference", "Frame_OK"] ("appended array") -> [w2686] mode=indexing
                      tunnel: "Data" ("group name in (Untitled)") -> [w2685]
                      tunnel: w2638 -> [w2684]
                      tunnel: w2639 -> [w2683]
                      tunnel: w2636 -> [w2682]
                      tunnel: w2637 -> [w2681]
                      tunnel: [w2680] -> w2635
                      tunnel: [w2679] -> _
                      n1598 = TDMS Set Properties(5:w2683, 7:w2684, 8:w2682, 9:w2686, 10:w2685, 11:w2681) -> (0:w2680:errorcluster, 3:w2679:refnum<k34>)  [unwired: 2 out]
                    }
                    n1599 = Merge Errors(w2587, w2676, w2602, w2635, w2616) -> (w2671:errorcluster)
                    n1600 = property on="Data filtering" class="Ring (strict)"(error in=w2671, "DisabledEnum"=T12."Disabled and Grayed Out" ("Disabled")) -> (error out=w2670:errorcluster)  [unwired: 1 in, 1 out]
                    n1601 = property on="Exit (recording)" class="Bool"(error in=w2670, "DisabledEnum"=T12."Enabled" ("Disabled")) -> (error out=w2617:errorcluster)  [unwired: 1 in, 1 out]
                    n1602 = property on="Additional recording settings" class="Bool (strict)"(error in=w2617, "DisabledEnum"=w2619) -> (error out=w2618:errorcluster)  [unwired: 1 in, 1 out]
                    n1603 = property on="Bridge swap" class="Bool (strict)"(error in=w2618, "DisabledEnum"=w2619) -> (error out=w2673:errorcluster)  [unwired: 1 in, 1 out]
                    n1604 = property on="Bridge offset" class="DigNum (strict)"(error in=w2673, "DisabledEnum"=w2619) -> (error out=w2672:errorcluster)  [unwired: 1 in, 1 out]
                    n1605 = global write "SW_Globals.vi" "Start time is set"(FALSE ("Start time is set")) -> ()
                  }
                }
                n1606 = Unbundle By Name(w2571) -> ("Recording now"=w2573:refnum<notifier>, "Has been recorded"=w2577:refnum<notifier>)
                n1607 = Send Notification(notification=TRUE, notifier=w2573, error in (no error)=w2570) -> ()  [unwired: 2 out]
                n1608 = Send Notification(notification=TRUE, notifier=w2577, error in (no error)=w2570) -> (error out=w2575:errorcluster)  [unwired: 1 out]
                n1609 = property on="Record timestamp" class="DigNum (strict)"(error in=w2575, "DisabledEnum"=T12."Enabled" ("Disabled")) -> ()  [unwired: 1 in, 2 out]
              }
            }
            n1610 = Subtract(x=w2554, y=w2558) -> (x-y=w2544:dbl)
            "Record timestamp" <- w2544
            n1611 = property on="Stop record at" class="DigNum (strict)"() -> ("Value"=w2543:dbl)  [unwired: 2 in, 2 out]
            n1612 = Subtract(x=w2543, y=w2544) -> (x-y=w2542:dbl)
            n1613 = Round Toward +Infinity(x=w2542) -> (ceil(x): smallest int >= x=w2545:dbl)
            n1614 = feedback-in #10(w2545) -> ()
            n1615 = feedback #10(0.0) -> (w2549:dbl)
            n1616 = Not Equal?(x=w2549, y=w2545) -> (x != y?=w2548:bool)
            n1617 = property on="\"Stop at\" enabled" class="Bool (strict)"() -> ("Value"=w2546:bool)  [unwired: 2 in, 2 out]
            n1618 = And(x=w2546, y=w2548) -> (x .and. y?=w2547:bool)
            n1619 = Greater Or Equal?(x=w2544, y=w2543) -> (x >= y?=w2552:bool)
            n1620 = case shown="True" w2547 {
              tunnel: w2545 -> [_ w2561]
              frame False {
              }
              frame True {
                n1621 = Format Date/Time String() -> ()  [unwired: 3 in, 1 out]
                n1622 = Format Date/Time String(time format string (%c)="%H:%M:%S" ("format string"), seconds (now)=w2561, UTC format=TRUE) -> (date/time string=w2560:string)
                n1623 = property on="Additional record settings" class="Bool (strict)"("BoolText.Text"=w2560) -> ()  [unwired: 2 in, 2 out]
              }
            }
            n1624 = And(x=w2552, y=w2546) -> (x .and. y?=w2551:bool)
            n1625 = case shown="True" w2551 {
              frame False {
              }
              frame True {
                n1626 = property on="Record/Stop" class="Bool (strict)"("Val(Sgnl)"=FALSE ("Record/Stop")) -> ()  [unwired: 2 in, 2 out]
              }
            }
          }
        }
        n1627 = disable-structure shown="Disabled" {
          disable-tunnel: w2170 -> [w2308 _]
          disable-tunnel: w2169 -> [w2307 _]
          disable-tunnel: w2168 -> [w2306 _]
          disable-tunnel: w2167 -> [w2305 _]
          frame Disabled {
            w2269 = FALSE ("use system decimal point (T)")
            w2260 = "\t"
            w2278 = i16 3 ("precision (6)")
            n1628 = property on="Mouse speed digi" class="DigNum (strict)"() -> ("Value"=w2259:dbl)  [unwired: 2 in, 2 out]
            n1629 = Number To Fractional String(use system decimal point (T)=TRUE, number=w2259, precision (6)=i16 3) -> (F-format string=w2256:string)  [unwired: 1 in]
            n1630 = Index Array "R"(array=w2305, index=6) -> (element=w2263:string)
            n1631 = Index Array "phi"(array=w2305, index=7) -> (element=w2280:string)
            n1632 = Fract/Exp String To Number(use system decimal point (T)=FALSE, string=w2280) -> (number=w2273:dbl)  [unwired: 2 in, 1 out]
            n1633 = Greater Than 0?(x=w2273) -> (x > 0?=w2277:bool)
            n1634 = Select(t=-180.0, s=w2277, f=180.0) -> (s? t:f=w2274:dbl)
            n1635 = Add(x=w2274, y=w2273) -> (x+y=w2272:dbl)
            n1636 = Select(t=w2272, f=w2273) -> (s? t:f=w2282:dbl)  [unwired: 1 in]
            n1637 = Fract/Exp String To Number(use system decimal point (T)=w2269, string=w2263) -> (number=w2271:dbl)  [unwired: 2 in, 1 out]
            n1638 = global read "SW_Globals.vi" "Current zone"() -> (w2266:u8)
            n1639 = Negate(x=w2308) -> (-x=w2293:dbl)
            n1640 = Negate(x=w2307) -> (-x=w2294:dbl)
            n1641 = Number To Fractional String(use system decimal point (T)=FALSE, number=w2282, precision (6)=w2278) -> (F-format string=w2267:string)  [unwired: 1 in]
            n1642 = Number To Fractional String(use system decimal point (T)=w2269, number=w2271, precision (6)=i16 3) -> (F-format string=w2268:string)  [unwired: 1 in]
            n1643 = property on="Record timestamp" class="DigNum (strict)"() -> ("Value"=w2295:dbl)  [unwired: 2 in, 2 out]
            n1644 = Select(t=w2293, f=w2308) -> (s? t:f=w2286:dbl)  [unwired: 1 in]
            n1645 = Select(t=w2294, f=w2307) -> (s? t:f=w2287:dbl)  [unwired: 1 in]
            n1646 = Number To Fractional String(use system decimal point (T)=FALSE, number=w2287, precision (6)=w2278) -> (F-format string=w2298:string)  [unwired: 1 in]
            n1647 = Number To Fractional String(use system decimal point (T)=FALSE, number=w2286, precision (6)=w2278) -> (F-format string=w2297:string)  [unwired: 1 in]
            n1648 = Number To Fractional String(use system decimal point (T)=FALSE, number=w2266, precision (6)=i16 0) -> (F-format string=w2261:string)  [unwired: 1 in]
            n1649 = Greater Than 0?(x=w2306) -> (x > 0?=w2292:bool)
            n1650 = Select(t=-180.0, s=w2292, f=180.0) -> (s? t:f=w2289:dbl)
            n1651 = Format Date/Time String(time format string (%c)="%H:%M:%S%.;%3u " ("format string"), seconds (now)=w2295, UTC format=TRUE) -> (date/time string=w2302:string)
            n1652 = Add(x=w2289, y=w2306) -> (x+y=w2288:dbl)
            n1653 = Select(t=w2288, f=w2306) -> (s? t:f=w2285:dbl)  [unwired: 1 in]
            n1654 = Number To Fractional String(use system decimal point (T)=FALSE, number=w2285, precision (6)=w2278) -> (F-format string=w2296:string)  [unwired: 1 in]
            n1655 = Concatenate Strings(w2302, w2260, w2298, w2260, w2297, w2260, w2296, w2260, w2268, w2260, w2267, w2260, w2256, w2260, w2261, "\r\n") -> (w2252:string)
            n1656 = property on="Output to the external terminal" class="Str"("Value"=w2252) -> ()  [unwired: 2 in, 2 out]
            n1657 = property on="Streaming" class="Bool (strict)"() -> ("Value"=w2253:bool)  [unwired: 2 in, 2 out]
            n1658 = case shown="True" w2253 {
              tunnel: [w2317 w2321] -> _
              tunnel: w2252 -> [_ w2320]
              tunnel: [_ w2319] -> w2254
              frame False {
                n1659 = property on="Serial OUT name" class="VISAName"() -> ("Value"=w2317:refnum<visa-resource-name>)  [unwired: 2 in, 2 out]
              }
              frame True {
                n1660 = VISA Write(write buffer=w2320) -> (VISA resource name out=w2321:refnum<visa-resource-name>, return count=w2318:u32, error out=w2319:errorcluster)  [unwired: 2 in]
              }
            }
            n1661 = case shown="Error" w2254 {
              tunnel: [TRUE ("write status") FALSE ("write status")] -> w2255
              frame No Error {
              }
              frame Error {
                w2314 = u32 0
                n1662 = feedback #11(w2314) -> (w2311:u32)
                n1663 = Increment(x=w2311) -> (x+1=w2313:u32)
                n1664 = Greater?(x=w2313, y=u32 15) -> (0:w2315:bool)
                n1665 = Select(t=w2314, s=w2315, f=w2313) -> (s? t:f=w2312:u32)
                n1666 = feedback-in #11(w2312) -> ()
              }
            }
            "write status" <- w2255
          }
          frame Enabled {
          }
        }
        n1667 = Or(x="Reset barplot", y=w2230) -> (x .or. y?=w2231:bool)
        n1668 = case shown="True" w2230 {
          frame False {
          }
          frame True {
            w2336 = waveform(dbl)[] [] ("History Data")
            n1669 = property on="Mouse speed" class="WFChart (strict)"("History Data"=w2336) -> ()  [unwired: 2 in, 2 out]
            n1670 = property on="Mouse speed 2" class="WFChart (strict)"("History Data"=w2336) -> ()  [unwired: 2 in, 2 out]
          }
        }
        n1671 = case shown="True" w2231 {
          frame False {
          }
          frame True {
            n1672 = global read "SW_Globals.vi" "Speed distribution array"() -> (w2347:u32[])
            n1673 = global read "SW_Globals.vi" "Zones allocation array"() -> (w2350:i32[])
            n1674 = global read "SW_Globals.vi" "Run Lengts distribution array"() -> (w2344:u32[])
            n1675 = global read "SW_Globals.vi" "Run Times distribution array"() -> (w2337:u32[])
            n1676 = Array Size(array=w2350) -> (size(s)=w2352:i32)
            n1677 = Array Size(array=w2347) -> (size(s)=w2345:i32)
            n1678 = Array Size(array=w2337) -> (size(s)=w2338:i32)
            n1679 = Array Size(array=w2344) -> (size(s)=w2343:i32)
            n1680 = Initialize Array(0 ("element"), w2352) -> (w2349:i32[])
            n1681 = Initialize Array(u32 0 ("element"), w2345) -> (w2348:u32[])
            n1682 = global write "SW_Globals.vi" "Zones allocation array"(w2349) -> ()
            n1683 = global write "SW_Globals.vi" "Speed distribution array"(w2348) -> ()
            n1684 = Initialize Array(u32 0 ("element"), w2338) -> (w2340:u32[])
            n1685 = Initialize Array(u32 0 ("element"), w2343) -> (w2341:u32[])
            n1686 = global write "SW_Globals.vi" "Run Times distribution array"(w2340) -> ()
            n1687 = global write "SW_Globals.vi" "Run Lengts distribution array"(w2341) -> ()
          }
        }
      }
      frame "Analysis" {
        n1688 = Unbundle By Name(w2728) -> ("Has been recorded"=w2730:refnum<notifier>)
        n1689 = disable-structure shown="Enabled" {
          frame Enabled {
            n1690 = event shown="[2] \"Back to Settings\": Value Change" {
              selector: _ -> [_ _ _]
              dyn-events: _ -> [_ _ _]
              timeout: 0 -> [_ _ _]
              event Timeout {
                n1691 = event-data() -> ()  [unwired: 1 in, 3 out]
              }
              event "Play/Pause": Value Change {
                n1692 = event-data() -> ("NewVal"=w2745:bool)  [unwired: 1 in, 5 out]
                n1693 = case shown="True" w2745 {
                  frame False {
                    n1694 = property on="Back to Settings" class="Bool (strict)"("DisabledEnum"=T12."Enabled" ("Disabled")) -> ()  [unwired: 2 in, 2 out]
                  }
                  frame True {
                    n1695 = property on="Back to Settings" class="Bool (strict)"("DisabledEnum"=T12."Disabled and Grayed Out" ("Disabled")) -> ()  [unwired: 2 in, 2 out]
                  }
                }
              }
              event "Back to Settings": Value Change {
                n1696 = event-data() -> ("NewVal"=w2748:bool)  [unwired: 1 in, 5 out]
                n1697 = case shown="True" w2748 {
                  frame False {
                  }
                  frame True {
                    w2752 = FALSE ("Stopped")
                    w2768 = FALSE ("Visible")
                    w2788 = enum32{"Settings", "Recording", "Analysis"}."Settings" ("Main tab control")
                    w2784 = enum32{"Settings", "Recording", "Analysis"}."Recording" ("Main tab control")
                    w2775 = enum32{"Settings", "Recording", "Analysis"}."Analysis" ("Main tab control")
                    n1698 = property on="Diagram at recording" class="Pict" props=["Bounds"]() -> (error out=w2772:errorcluster)  [unwired: 2 in, 2 out]
                    n1699 = property on="Main tab control" class="TabCtl (strict)"(error in=w2772, "Value"=w2775) -> (error out=w2779:errorcluster, "Pages"=w2774:refnum<vi>[])  [unwired: 1 in, 1 out]
                    n1700 = To Long Integer(number=w2775) -> (32bit integer=w2776:i32)
                    n1701 = Index Array(array=w2774, index=w2776) -> (element=w2777:refnum<vi>)
                    n1702 = property class="Page"(reference=w2777, error in=w2779, "PageEnb"=T32."Page Disabled & Grayed" ("Page Enabled State")) -> (error out=w2786:errorcluster)  [unwired: 1 out]
                    n1703 = property on="Main tab control" class="TabCtl (strict)"(error in=w2786, "Value"=w2784) -> (error out=w2780:errorcluster, "Pages"=w2785:refnum<vi>[])  [unwired: 1 in, 1 out]
                    n1704 = To Long Integer(number=w2784) -> (32bit integer=w2783:i32)
                    n1705 = Index Array(array=w2785, index=w2783) -> (element=w2782:refnum<vi>)
                    n1706 = property class="Page"(reference=w2782, error in=w2780, "PageEnb"=T32."Page Disabled & Grayed" ("Page Enabled State")) -> (error out=w2793:errorcluster)  [unwired: 1 out]
                    n1707 = property on="Main tab control" class="TabCtl (strict)"(error in=w2793, "Value"=w2788) -> (error out=w2792:errorcluster, "Pages"=w2787:refnum<vi>[])  [unwired: 1 in, 1 out]
                    n1708 = To Long Integer(number=w2788) -> (32bit integer=w2789:i32)
                    n1709 = Index Array(array=w2787, index=w2789) -> (element=w2790:refnum<vi>)
                    n1710 = property class="Page"(reference=w2790, error in=w2792, "PageEnb"=T32."Page Enabled" ("Page Enabled State")) -> (error out=w2773:errorcluster)  [unwired: 1 out]
                    n1711 = global read "SW_Globals.vi" "Cluster of paths"() -> (w2771:T22)
                    n1712 = property on="Back to Settings" class="Bool (strict)"(error in=w2773, "Visible"=w2768, "Value"=w2768) -> (error out=w2758:errorcluster)  [unwired: 1 in, 1 out]
                    n1713 = Unbundle By Name(w2771) -> ("Path to the settings file"=w2770:path)
                    n1714 = property on="Pane" class="Pane"(error in=w2758) -> (error out=w2760:errorcluster, "Decos[]"=w2761:refnum<vi>[])  [unwired: 1 in, 1 out]
                    n1715 = global read "SW_Globals.vi" "VISA resource name"() -> (w2749:refnum<visa-resource-name>)
                    n1716 = Index Array(array=w2761, index=0) -> (element=w2766:refnum<vi>)
                    n1717 = property class="Decor"(reference=w2766, error in=w2760, "Visible"=FALSE) -> (error out=w2759:errorcluster)  [unwired: 1 out]
                    n1718 = Index Array(array=w2761, index=2) -> (element=w2763:refnum<vi>)
                    n1719 = property class="Decor"(reference=w2763, error in=w2759, "Visible"=TRUE) -> (error out=w2757:errorcluster)  [unwired: 1 out]
                    n1720 = call <vilib>:"Open Config Data.vi"("error in (no error)"=w2757, "configuration file path"=w2770) -> ("error out"=w2750:errorcluster, "refnum"=w2769:T5)  [unwired: 7 in, 1 out]
                    n1721 = call "HW_Make_sure_stop_Acq_and_null_IO_ports.vi"("error In"=w2750, "VISA Resource name IN"=w2749) -> ()  [unwired: 2 out]
                    n1722 = local write "Settings file refnum out"(w2769) -> ()
                    n1723 = global write "SW_Globals.vi" "TTL recording start signal has been successfully reset"(FALSE ("TTL recording start signal has been successfully reset")) -> ()
                    n1724 = global write "SW_Globals.vi" "Recording has been stopped with TTL"(FALSE ("Recording has been started with TTL")) -> ()
                    n1725 = global write "SW_Globals.vi" "Recording has been started with TTL"(FALSE ("Recording has been started with TTL")) -> ()
                    n1726 = local write "Record timestamp"(0.0 ("Record timestamp")) -> ()
                    n1727 = local write "Reset starting pulse"(w2752) -> ()
                    n1728 = local write "TTL is long enough"(w2752) -> ()
                    n1729 = local write "Stopped"(TRUE ("Stopped")) -> ()
                    n1730 = local write "Record"(w2752) -> ()
                    n1731 = local write "Started"(w2752) -> ()
                  }
                }
              }
            }
          }
          frame Disabled {
          }
        }
        n1732 = Unbundle By Name(w2728) -> ("Data loaded"=w2737:refnum<notifier>)
        n1733 = Get Notifier Status(notifier=w2730) -> (current notification=w2727:bool)  [unwired: 1 in, 4 out]
        n1734 = Get Notifier Status(notifier=w2737) -> (current notification=w2735:bool)  [unwired: 1 in, 4 out]
        n1735 = Not(x=w2727) -> (.not. x?=w2729:bool)
        n1736 = Or(x=w2729, y=w2735) -> (x .or. y?=w2731:bool)
        n1737 = And(x=w2735, y="Play/Pause") -> (x .and. y?=w2738:bool)
        n1738 = Not(x="Play/Pause") -> (.not. x?=w2733:bool)
        n1739 = global read "SW_Globals.vi" "Density map with no zones and with full track"() -> (w2712:picture)
        n1740 = global read "SW_Globals.vi" "Density map with zones and full track"() -> (w2711:picture)
        n1741 = And(x=w2731, y=w2733) -> (x .and. y?=w2732:bool)
        n1742 = global read "SW_Globals.vi" "Density map with zones"() -> (w2713:picture)
        n1743 = global read "SW_Globals.vi" "Full track with no zones"() -> (w2716:picture)
        n1744 = global read "SW_Globals.vi" "Density map no zones"() -> (w2714:picture)
        n1745 = global read "SW_Globals.vi" "Full track with zones"() -> (w2715:picture)
        n1746 = global read "SW_Globals.vi" "Diagram no zones"() -> (w2718:picture)
        n1747 = case shown="True" w2732 {
          tunnel: w2728 -> [_ w2796]
          frame False {
          }
          frame True {
            n1748 = case "Open new file" shown="True" "Open File" {
              tunnel: w2796 -> [_ w2800]
              frame False {
              }
              frame True {
                n1749 = global read "SW_Globals.vi" "Cluster of paths"() -> (w2801:T22)
                n1750 = Unbundle By Name(w2801) -> ("Path to TDMS file"=w2811:path)
                n1751 = Strip Path(path=w2811) -> (stripped path=w2810:path)  [unwired: 1 out]
                n1752 = Strip Path(path=w2810) -> (stripped path=w2807:path)  [unwired: 1 out]
                n1753 = call "File Dialog"("start path"=w2807, "button label"="Open track", "pattern (all files)"="*.csv; *.tdms") -> ("selected path"=w2802:path, "exists"=w2806:bool, "cancelled"=w2804:bool, "error out"=w2799:errorcluster)  [unwired: 9 in]
                n1754 = Not(x=w2804) -> (.not. x?=w2805:bool)
                n1755 = And(x=w2806, y=w2805) -> (x .and. y?=w2803:bool)
                n1756 = case shown="True" w2803 {
                  tunnel: w2802 -> [_ w2816]
                  tunnel: w2801 -> [_ w2815]
                  tunnel: w2800 -> [_ w2813]
                  tunnel: w2799 -> [_ _]
                  frame False {
                  }
                  frame True {
                    n1757 = flat-sequence {
                      tunnel: w2816 -> [w2830]
                      tunnel: [w2829] -> w2814
                      tunnel: [w2818] -> w2812
                      tunnel: w2815 -> [w2836]
                      tunnel: w2814 -> [w2835]
                      tunnel: w2812 -> [w2833]
                      tunnel: w2813 -> [w2843]
                      frame #0 {
                        n1758 = call <vilib>:"Get File Extension.vi"("file"=w2830) -> ("filename without extension"=w2823:string, "lowercase file extension"=w2822:string)  [unwired: 6 in, 3 out]
                        n1759 = Concatenate Strings(w2823, ".trset" ("string")) -> (w2831:string)
                        n1760 = Strip Path(path=w2830) -> (stripped path=w2824:path)  [unwired: 1 out]
                        n1761 = Concatenate Strings(w2823, ".tdms" ("string")) -> (w2826:string)
                        n1762 = Concatenate Strings(w2823, ".csv" ("string")) -> (w2825:string)
                        n1763 = Build Path(base path=w2824, name or relative path=w2831) -> (appended path=w2829:path)
                        "Settings file path" <- w2829
                        n1764 = Build Path(base path=w2824, name or relative path=w2826) -> (appended path=w2819:path)
                        n1765 = Build Path(base path=w2824, name or relative path=w2825) -> (appended path=w2817:path)
                        n1766 = Equal?(x=w2822, y="tdms") -> (x = y?=w2820:bool)
                        n1767 = Select(t=w2819, s=w2820, f=w2817) -> (s? t:f=w2818:path)
                        "Track path" <- w2830
                      }
                      frame #1 {
                        n1768 = Bundle By Name(cluster=w2836, "Path to TDMS file"=w2833, "Recording settings output path"=w2835) -> (w2834:T22)
                        n1769 = global write "SW_Globals.vi" "Cluster of paths"(w2834) -> ()
                      }
                      frame #2 {
                        n1770 = Unbundle By Name(w2843) -> ("(Final) Data file is saved"=w2839:refnum<notifier>, "Data loaded"=w2842:refnum<notifier>, "Has been recorded"=w2837:refnum<notifier>)
                        n1771 = Send Notification(notification=TRUE, notifier=w2839) -> ()  [unwired: 1 in, 2 out]
                        n1772 = Send Notification(notification=FALSE, notifier=w2842) -> ()  [unwired: 1 in, 2 out]
                        n1773 = Send Notification(notification=TRUE, notifier=w2837) -> ()  [unwired: 1 in, 2 out]
                      }
                    }
                  }
                }
              }
            }
            n1774 = property on="Open File" class="Bool"("DisabledEnum"=T12."Enabled" ("Disabled")) -> (error out=w2794:errorcluster)  [unwired: 2 in, 1 out]
            n1775 = property on="Timeline" class="Slide (strict)"(error in=w2794, "DisabledEnum"=T12."Disabled and Grayed Out" ("Disabled")) -> ()  [unwired: 1 in, 2 out]
          }
        }
        n1776 = global read "SW_Globals.vi" "Diagram"() -> (w2717:picture)
        n1777 = Build Array(w2718, w2717, w2716, w2715, w2714, w2713, w2712, w2711) -> (w2724:picture[])
        n1778 = Index Array(array=w2724, index="Map index (analysis)") -> (element=w2723:picture)
        n1779 = case shown="True" w2738 {
          tunnel: w2723 -> [w2844 w2894]
          tunnel: "Zones (analysis)" -> [_ w2893]
          tunnel: [w2844 w2892] -> w2736
          tunnel: w2726 -> [_ w2873]
          frame False {
          }
          frame True {
            n1780 = disable-structure shown="Disabled" {
              frame Disabled {
                (unwired) "%<%H:%M:%S%3u%p%d.%m.%Y>T" ("format string")
                n1781 = Get Date/Time In Seconds() -> (seconds since 1Jan1904=w2910:timestamp)
                n1782 = Scan From String(default 1=w2910) -> ()  [unwired: 5 in, 3 out]
              }
              frame Enabled {
              }
            }
            n1783 = Divide(x=u32 1000, y=w2873) -> (x/y=w2875:dbl)
            n1784 = Multiply(x=w2875, y="Trace in analysis, s") -> (x*y=w2868:dbl)
            n1785 = local read "Absolute timestamp (rec)"() -> (w2882:dbl[])
            n1786 = local read "Relative timestamp (rec)"() -> (w2890:dbl[])
            n1787 = local read "alpha rot. angle"() -> (w2905:dbl[])
            n1788 = local read "Index of the last recorded timepoint"() -> (w2886:i32)
            n1789 = local read "TTL outputs"() -> (w2865:u8[])
            n1790 = local read "TTL inputs"() -> (w2866:u8[])
            n1791 = local read "Zones preference array (loaded)"() -> (w2878:dbl[][])
            n1792 = property on="Timeline" class="Slide (strict)"("DisabledEnum"=T12."Enabled" ("Disabled")) -> (error out=w2883:errorcluster)  [unwired: 2 in, 1 out]
            n1793 = property on="Open File" class="Bool"(error in=w2883, "DisabledEnum"=T12."Disabled and Grayed Out" ("Disabled")) -> ()  [unwired: 1 in, 2 out]
            n1794 = local read "X coord"() -> (w2907:dbl[])
            n1795 = local read "Y coord"() -> (w2906:dbl[])
            n1796 = feedback #12(0.0125 ("String")) -> (w2899:dbl)
            n1797 = Select(t=FALSE, s=w2893, f=TRUE) -> (s? t:f=w2851:bool)
            n1798 = feedback #13(0) -> (w2864:u32)
            n1799 = Index Array(array=w2905, index=w2864) -> (element=w2846:dbl)
            n1800 = Index Array(array=w2882, index=w2864) -> (element=w2881:dbl)
            n1801 = Index Array(array=w2866, index=w2864) -> (element=w2854:u8)
            n1802 = Index Array(array=w2865, index=w2864) -> (element=w2853:u8)
            n1803 = Index Array(array=w2890, index=w2864) -> (element=w2849:dbl)
            n1804 = feedback-in #12(w2849) -> ()
            n1805 = Add(x=w2854, y=w2853) -> (x+y=w2852:u8)
            n1806 = property on="Recorded timestamp" class="DigNum (strict)"("Value"=w2849) -> ()  [unwired: 2 in, 2 out]
            n1807 = Subtract(x=w2849, y=w2899) -> (x-y=w2898:dbl)
            n1808 = Index Array(array=w2878, index (row)=w2864) -> (element=→"Zones allocation (normalized) in analysis":dbl[])  [unwired: 1 in]
            n1809 = Index Array(array=w2907, index=w2864) -> (element=w2848:dbl)
            n1810 = Index Array(array=w2906, index=w2864) -> (element=w2847:dbl)
            n1811 = Number To Boolean Array(number=w2852) -> (Boolean array=w2855:bool[])
            n1812 = To Time Stamp(1:w2881) -> (0:w2880:timestamp)
            n1813 = property on="Recorded at time" class="AbsTime (strict)"("Value"=w2880) -> ()  [unwired: 2 in, 2 out]
            n1814 = call "FL_Calc_speed_on_the_fly.vi"("Y coord, mm"=w2847, "X coord, mm"=w2848, "Time per frame, s"=w2898) -> ("Mouse speed, mm/s"=w2896:dbl)
            "Mouse speed digi 2" <- w2896
            n1815 = To Time Stamp(1:w2849) -> (0:w2900:timestamp)
            n1816 = Build Array(w2896) -> (w2901:dbl[])
            n1817 = Index Array(array=w2855, index=3) -> (element=→"TTL IO 4 (analysis)":bool)
            n1818 = Index Array(array=w2855, index=0) -> (element=→"TTL IO 1 (analysis)":bool)
            n1819 = Index Array(array=w2855, index=1) -> (element=→"TTL IO 2 (analysis)":bool)
            n1820 = Index Array(array=w2855, index=2) -> (element=→"TTL IO 3 (analysis)":bool)
            n1821 = Bundle By Name("t0"=w2900, "Y"=w2901) -> (→"Mouse speed 2":waveform(dbl))  [unwired: 1 in]
            n1822 = feedback #14(u16 3 ("Value")) -> (w2872:u16)
            n1823 = event shown="[2] \"Diagram at analysis\": Mouse Up" {
              selector: _ -> [_ _ _ _]
              dyn-events: _ -> [_ _ _ _]
              timeout: 1 -> [_ _ _ _]
              tunnel: w2849 -> [w2919 _ _ _]
              tunnel: w2864 -> [w2918 _ w2933 w2941]
              tunnel: [w2917 w2929 w2933 w2941] -> w2889
              tunnel: w2890 -> [_ _ _ _]
              tunnel: w2886 -> [_ w2922 _ _]
              tunnel: [w2911 w2920 w2932 w2940] -> w2870
              tunnel: w2872 -> [_ w2920 w2932 w2940]
              event Timeout {
                n1824 = event-data() -> ()  [unwired: 1 in, 3 out]
                n1825 = property on="Timeline" class="Slide (strict)"("Value"=w2919) -> ()  [unwired: 2 in, 2 out]
                n1826 = property on="Speed" class="Ring (strict)"() -> ("RingText.Text"=w2915:string, "Strings []"=w2916:string[], "StringsAndValues[]"=w2913:T57)  [unwired: 2 in, 2 out]
                n1827 = Search 1D Array(1D array=w2916, element=w2915) -> (index of element=w2914:i32)  [unwired: 1 in]
                n1828 = Index Array(array=w2913, index=w2914) -> (element=w2912:cluster{"String":string, "Value":u16})
                n1829 = Unbundle(w2912) -> ("Value"=w2911:u16)  [unwired: 1 out]
                n1830 = Add(x=w2911, y=w2918) -> (x+y=w2917:u32)
              }
              event "Timeline": Value Change {
                n1831 = event-data() -> ("NewVal"=w2927:dbl)  [unwired: 1 in, 5 out]
                n1832 = property on="Timeline" class="Slide (strict)"() -> ("Scale.Maximum"=w2928:dbl, "Scale.Minimum"=w2926:dbl)  [unwired: 2 in, 2 out]
                n1833 = Subtract(x=w2927, y=w2926) -> (x-y=w2925:dbl)
                n1834 = Subtract(x=w2928, y=w2926) -> (x-y=w2924:dbl)
                n1835 = Divide(x=w2925, y=w2924) -> (x/y=w2923:dbl)
                "ceil(x): smallest int >= x" <- w2923
                n1836 = Multiply(x=w2923, y=w2922) -> (x*y=w2921:dbl)
                n1837 = To Unsigned Long Integer(number=w2921) -> (unsigned 32bit integer=w2929:u32)
              }
              event "Diagram at analysis": Mouse Up {
                n1838 = event-data() -> ("Coords"=w2930:T4, "Button"=w2931:u16)  [unwired: 1 in, 6 out]
                n1839 = case shown="1" w2931 {
                  tunnel: w2930 -> [_ w2936]
                  frame 0, Default {
                  }
                  frame 1 {
                    n1840 = property on="Diagram at analysis" class="Pict"() -> ("Bounds"=w2938:T19, "Position"=w2937:T58)  [unwired: 2 in, 2 out]
                    n1841 = local read "Pixels per mm"() -> (w2939:dbl)
                    n1842 = Subtract(x=w2936, y=w2937) -> (x-y=w2935:T4)
                    n1843 = call "GET_Click_Coords.vi"("Screen coords in, pix"=w2935, "Size of the image"=w2938, "Pixels per mm"=w2939) -> ("Click coords, mm"=→"Click coords, mm":T59)  [unwired: 12 in]
                  }
                }
              }
              event "Multiplyer of chart RX 2": Value Change {
                n1844 = event-data() -> ("NewVal"=w2942:u8)  [unwired: 1 in, 5 out]
                n1845 = property on="Mouse speed 2" class="WFChart (strict)"() -> (error out=w2944:errorcluster, "XScale.Maximum"=w2947:dbl)  [unwired: 2 in, 1 out]
                n1846 = Multiply(x=w2942, y=10.0) -> (x*y=w2943:dbl)
                n1847 = Subtract(x=w2947, y=w2943) -> (x-y=w2945:dbl)
                n1848 = property on="Mouse speed 2" class="WFChart (strict)"(error in=w2944, "XScale.Minimum"=w2945) -> ()  [unwired: 1 in, 2 out]
              }
            }
            n1849 = feedback-in #14(w2870) -> ()
            n1850 = Greater Or Equal?(x=w2889, y=w2886) -> (x >= y?=w2879:bool)
            n1851 = Divide(x=w2870, y=u16 3) -> (x/y=w2867:dbl)
            n1852 = Select(t=u32 0, s=w2879, f=w2889) -> (s? t:f=w2888:u32)
            n1853 = feedback-in #13(w2888) -> ()
            n1854 = property on="Diagram at analysis" class="Pict"() -> ("Bounds"=w2909:T19)  [unwired: 2 in, 2 out]
            n1855 = local read "Pixels per mm"() -> (w2908:dbl)
            n1856 = Divide(x=w2868, y=w2867) -> (x/y=w2845:dbl)
            n1857 = Round To Nearest(number=w2845) -> (nearest integer value=w2850:dbl)
            n1858 = call "SW_Draw_mouse_br.vi"("Input picture (background)"=w2894, "Size of the image"=w2909, "Pixels per mm"=w2908, "Mouse coord cartesian X, mm"=w2848, "Mouse coord cartesian Y, mm"=w2847, "Mouse angle of rotation, deg"=w2846, "Show mouse lineout"=w2851, "Trace length, samples"=w2850) -> ("Output picture (with mouse overlay)"=w2892:picture)  [unwired: 6 in, 1 out]
          }
        }
        "Diagram at analysis" <- w2736
        n1859 = event shown="[1] \"Zones (analysis)\", \"Show full track (analysis)\", \"Show heatmap (analysis)\": Value Change" {
          selector: _ -> [_ _]
          dyn-events: _ -> [_ _]
          timeout: 0 -> [_ _]
          tunnel: "Zones (analysis)" -> [_ w2743]
          tunnel: "Show full track (analysis)" -> [_ w2742]
          tunnel: "Show heatmap (analysis)" -> [_ w2740]
          event Timeout {
            n1860 = event-data() -> ()  [unwired: 1 in, 3 out]
          }
          event "Zones (analysis)", "Show full track (analysis)", "Show heatmap (analysis)": Value Change {
            n1861 = event-data() -> ()  [unwired: 1 in, 6 out]
            n1862 = Build Array(w2743, w2742, w2740) -> (w2741:bool[])
            n1863 = Boolean Array To Number(Boolean array=w2741) -> (number=w2739:u32)
            n1864 = property on="Map index (analysis)" class="DigNum (strict)"("Value"=w2739) -> ()  [unwired: 2 in, 2 out]
          }
        }
      }
    }
    n1865 = Get Notifier Status(notifier=w1477, error in (no error)=w1478) -> (current notification=w1479:bool)  [unwired: 4 out]
    n1866 = Or(x="Stop Button", y=w1479) -> (x .or. y?=w1480:bool)
    n1867 = node-c288() -> ()  [unwired: 1 in, 1 out]
  }
  n1868 = node-c288(w41) -> ()  [unwired: 1 out]
  "Reset starting pulse" <- FALSE ("Reset starting pulse")
  "TTL is long enough" <- FALSE ("TTL is long enough")
  "Started" <- FALSE ("Started")
  "Stopped" <- TRUE ("Stopped")
  "Record" <- FALSE ("Record")
